vi "myRIO_BRig_RT_v0,86_PortC.vi"() -> ()   [LabVIEW 2014]
uses:
  myRIO_BRig_RT__Case_Exp_stateList.ctl
  myRIO_BRig_RT__Case_NonExp_stateList.ctl
  <vilib>/Platform/TimedLoop/XDataNode/timing_clust.ctl
  <vilib>/Platform/TimedLoop/XDataNode/nitl_modes.ctl
  <vilib>/Platform/TimedLoop/XDataNode/wakeup.ctl
  <vilib>/WebDAVClient/Advanced/SessionHandle.ctl
  <vilib>/myRIO/Common/Instrument Driver Framework/myRIO v1.0/UART/vis/myRIO v1.0 Close UART.vi
  <vilib>/FPGAPlugInAG/myRIO-1900/niLvFpga_Open_myRIO-1900.vi
  <vilib>/rvi/interface/common/dynamic/niFpgaDynamicAddResources.vi
  <vilib>/Utility/error.llb/Error Cluster From Error Code.vi
  <vilib>/rvi/errors/niLvFpgaAdjustHostInterfaceError.vi
  <vilib>/FPGAPlugInAG/Dynamic/niLvFpga_Close_Dynamic.vi
  <vilib>/myRIO/Common/Instrument Driver Framework/Utilities/vis/FPGA Ref Manager.vi
  <vilib>/myRIO/Common/Instrument Driver Framework/myRIO v1.0/myRIO v1.0 Reset FPGA.vi
  <vilib>/myRIO/Common/Instrument Driver Framework/myRIO v1.0/IRQ/vis/myRIO v1.0 IRQ Info FGV.vi
  <vilib>/myRIO/Common/Instrument Driver Framework/myRIO v1.0/IRQ/vis/myRIO v1.0 Timer IRQ Info FGV.vi
  <vilib>/myRIO/Common/Instrument Driver Framework/myRIO v1.0/IRQ/vis/myRIO v1.0 ISR Agent.vi
  <vilib>/rvi/interface/nirviOpenFPGA/nirviOpenFPGA.xnode
  myRIO_BRig_FPGA_v3,81__PortC__build.lvbitx
  myRIO_BRig_FPGA_v3,81__PortC.vi
  <vilib>/rvi/interface/nirviReadWriteControl/nirviReadWriteControl.xnode
  <vilib>/Platform/TimedLoop/XDataNode/XDataNode.xnode
  <vilib>/rvi/interface/nirviCloseFPGA/nirviCloseFPGA.xnode
  <vilib>/Platform/TimedLoop/XDataNode/XDNodeRunTimeDep.lvlib
  <vilib>/rvi/interface/Simulation/niFpgaSimulationCallBeginRW.vi
  <vilib>/myRIO/Instrument Drivers/Utilities/Utilities.lvlib
  <vilib>/WebDAVClient/NI_WebDAV.lvlib
  NiFpgaLv.dll
panel:
  in  "Laser2_baseline":bool
  in  "Laser1_baseline":bool
  in  "CueLed_baseline":bool
  out "allReward_R":bool
  out "allReward_L":bool
  in  "I_allReward":bool caption="NonSpecific Lick Direction"
  in  "Tcycle_Reward_max_R":u16=1000 caption="Max" min=5 max=5000 step=5
  in  "Tcycle_Reward_min_R":u16=1000 caption="Min" min=5 max=5000 step=5
  in  "Tcycle_Reward_step_R":u16=1000 caption="Penalty" min=1 max=10000 step=1
  in  "Tcycle_Reward_max_L":u16=1000 caption="Max" min=5 max=5000 step=5
  in  "Tcycle_Reward_min_L":u16=1000 caption="Min" min=5 max=5000 step=5
  in  "Tcycle_Reward_step_L":u16=1000 caption="Penalty" min=1 max=10000 step=1
  in  "MTrig_CueLed":bool
  out "Threshold":bool
  out "tLoop":dbl
  in  "Tcycle_Cue_LED_max":u16=1000 caption="Max" min=5 max=5000 step=5
  in  "Tcycle_Cue_LED_min":u16=1000 caption="Min" min=5 max=5000 step=5
  in  "Tcycle_CuePenalty_LED":u16=1000 caption="Penalty" min=1 max=10000 step=1
  out "power_l2":dbl
  in  "MTrig_Laser_Switch":bool
  in  "Cue1Param_AudioLed_Count_NS":u16
  in  "Cue1Param_AudioLed_Count_Switch":u16
  in  "Cue1Param_AudioLed_Probability_NS":u16
  in  "Cue1Param_CueType_NS":u16(slide) max=3 step=1 scale=0.0..3.0
  in  "Cue1Param_AudioLed_Probability_Switch":u16
  in  "Cue1Param_CueType_Switch":u16(slide) max=3 step=1 scale=0.0..3.0
  in  "CueLed_Freq":dbl=10.0
  in  "CueLed_Tpeak":dbl=2.0
  in  "Laser_power_step_l2":dbl
  in  "Laser_power_max_l2":dbl
  in  "Laser_power_min_l2":dbl
  in  "Laser_Tshutter_l2":dbl=2.0
  in  "Laser_Freq_l2":dbl=10.0
  in  "Laser_Tpeak_l2":dbl=2.0
  in  "Laser_duration_l2":u16
  in  "LC_Sel_Count_NS_l2":u16
  in  "LC_Sel_Count_Switch_l2":u16
  in  "LC_Sel_Probability_NS_l2":u16
  in  "LC_Sel_Block_NS_l2":u16(slide) max=2 step=1 scale=0.0..2.0
  in  "LC_Sel_OnOff_NS_l2":bool
  in  "LC_Sel_Probability_Switch_l2":u16
  in  "LC_Sel_Block_Switch_l2":u16(slide) max=2 step=1 scale=0.0..2.0
  in  "LC_Sel_OnOff_Switch_l2":bool
  in  "LC_Sel_Tdelay_NS_l2":u16
  in  "LC_Sel_Tdelay_Switch_l2":u16
  in  "LC_Cue1_Count_NS_l2":u16
  in  "LC_Cue1_Count_Switch_l2":u16
  in  "LC_Cue1_delayOpt_NS_l2":bool
  in  "LC_ENL1_delayOpt_NS_l2":bool
  in  "LC_ENL1_Count_NS_l2":u16
  in  "LC_ENL1_Count_Switch_l2":u16
  in  "LC_Cue1_delayOpt_Switch_l2":bool
  in  "LC_ENL1_delayOpt_Switch_l2":bool
  in  "LC_Cue1_Probability_NS_l2":u16
  in  "LC_Cue1_Block_NS_l2":u16(slide) max=2 step=1 scale=0.0..2.0
  in  "LC_Cue1_OnOff_NS_l2":bool
  in  "LC_Cue1_Probability_Switch_l2":u16
  in  "LC_Cue1_Block_Switch_l2":u16(slide) max=2 step=1 scale=0.0..2.0
  in  "LC_Cue1_OnOff_Switch_l2":bool
  in  "LC_ENL1_Probability_NS_l2":u16 max=100 step=1
  in  "LC_ENL1_Block_NS_l2":u16(slide) max=2 step=1 scale=0.0..2.0
  in  "LC_ENL1_OnOff_NS_l2":bool
  in  "LC_ENL1_Probability_Switch_l2":u16 max=100 step=1
  in  "LC_ENL1_Block_Switch_l2":u16(slide) max=2 step=1 scale=0.0..2.0
  in  "LC_Cue1_Tdelay_NS_l2":u16
  in  "LC_ENL1_Tdelay_NS_l2":u16
  in  "LC_Cue1_Tdelay_Switch_l2":u16
  in  "LC_ENL1_Tdelay_Switch_l2":u16
  in  "LC_ENL1_OnOff_Switch_l2":bool
  in  "LC_Wrong_Probability_l2":u16
  in  "LC_Wrong_Trial_l2":u16(slide) max=2 step=1 scale=0.0..2.0
  in  "LC_Wrong_Block_l2":u16(slide) max=2 step=1 scale=0.0..2.0
  in  "LC_Wrong_OnOff_l2":bool
  in  "LC_Reward_Probability_l2":u16
  in  "LC_Reward_Trial_l2":u16(slide) max=2 step=1 scale=0.0..2.0
  in  "LC_Reward_Block_l2":u16(slide) max=2 step=1 scale=0.0..2.0
  in  "LC_Reward_OnOff_l2":bool
  in  "LC_Wrong_Tdelay_l2":u16
  in  "LC_Reward_Tdelay_l2":u16
  in  "LC_Sel_Count_NS_l1":u16
  in  "LC_Sel_Count_Switch_l1":u16
  in  "LC_Sel_Probability_NS_l1":u16
  in  "LC_Sel_Block_NS_l1":u16(slide) max=2 step=1 scale=0.0..2.0
  in  "LC_Sel_OnOff_NS_l1":bool
  in  "LC_Sel_Probability_Switch_l1":u16
  in  "LC_Sel_Block_Switch_l1":u16(slide) max=2 step=1 scale=0.0..2.0
  in  "LC_Sel_OnOff_Switch_l1":bool
  in  "LC_Sel_Tdelay_NS_l1":u16
  in  "LC_Sel_Tdelay_Switch_l1":u16
  out "I_connect_TCP":bool
  in  "get_countPerMS":bool
  in  "count_warmup_R_reset":bool
  in  "count_warmup_L_reset":bool
  out "count_warmup_R":u16
  out "count_warmup_L":u16
  out "SolenoidReward":bool
  in  "SolenoidProbability_L":u16=100 caption="Reward Time [ms]" min=1 max=1000 step=1
  in  "SolenoidProbability_R":u16=100 caption="Reward Time [ms]" min=1 max=1000 step=1
  out "power_l1":dbl caption="LaserPower"
  in  "Laser_power_step_l1":dbl
  in  "Laser_power_max_l1":dbl
  in  "Recording":bool
  in  "Laser_power_min_l1":dbl
  in  "FPGA_count2ms":dbl=159.0
  in  "Laser_Tshutter_l1":dbl=2.0
  in  "Laser_Freq_l1":dbl=10.0
  in  "Laser_Tpeak_l1":dbl=2.0
  in  "Laser_duration_l1":u16
  out "error out":errorcluster
  in  "LC_Cue1_Count_NS_l1":u16
  in  "LC_Cue1_Count_Switch_l1":u16
  in  "LC_Cue1_delayOpt_NS_l1":bool
  in  "LC_ENL1_delayOpt_NS_l1":bool
  in  "LC_ENL1_Count_NS_l1":u16
  in  "LC_ENL1_Count_Switch_l1":u16
  in  "LC_Cue1_delayOpt_Switch_l1":bool
  in  "LC_ENL1_delayOpt_Switch_l1":bool
  in  "Tcycle_Cue_Audio_max":u16=1000 caption="Max" min=5 max=5000 step=5
  in  "Tcycle_Cue_Audio_min":u16=1000 caption="Min" min=5 max=5000 step=5
  in  "SendData":bool
  out "cSpout":enum16{"Left", "Right"}(ring) caption="Left or Right Spout"
  out "A4":u32 caption="LickCounter_Right"
  out "A2":u32 caption="LickCounter_Left"
  in  "LR_wrong_Event":bool
  out "SelectWrong":bool
  out "SelectReward":bool
  in  "Left(F)_or_Right(T)":bool
  in  "ignoreWrong":bool
  in  "SelectionState":bool
  in  "LR_wrong_Laser":bool
  in  "LR_reward_Laser":bool
  in  "LR_reward_Event":bool
  out "nRewards_Right":u16 caption="# Rewards Total (Right)"
  out "nRewards_Left":u16 caption="# Rewards Total (Left)"
  out "nRewards_cur":u16 caption="# Rewards in Current Block"
  out "TpB_target":u16 caption="Target Trials Per Block"
  out "cState_NonExp":T1 caption="WarmUp State"
  out "iBlock":u16 caption="Current Block"
  out "cState":T2 caption="Experimental State"
  out "iTrial":u16 caption="Current Trial"
  in  "warmupType":u8(slide) max=2 step=1 scale=0.0..2.0
  in  "TestConnection":bool
  in  "warmup":bool caption="WarmUp"
  in  "Data Set Prefix":string="Exp1_TM2"
  out "Connected To Host?":bool
  in  "Host Password":string="sabalab"
  in  "Host UserName":string="Test2"
  in  "sp_RightSpout":u16(slide)=2 max=2 step=1 scale=0.0..2.0
  in  "sp_LeftSpout":u16(slide)=2 max=2 step=1 scale=0.0..2.0
  in  "BUR_max":u16 caption="Count Reward Structure  (0 = off)"
  in  "LC_Wrong_Probability_l1":u16
  in  "LC_Wrong_Trial_l1":u16(slide) max=2 step=1 scale=0.0..2.0
  in  "LC_Wrong_Block_l1":u16(slide) max=2 step=1 scale=0.0..2.0
  in  "LC_Wrong_OnOff_l1":bool
  in  "LC_Reward_Probability_l1":u16
  in  "LC_Reward_Trial_l1":u16(slide) max=2 step=1 scale=0.0..2.0
  in  "LC_Reward_Block_l1":u16(slide) max=2 step=1 scale=0.0..2.0
  in  "LC_Reward_OnOff_l1":bool
  in  "LC_Cue1_Probability_NS_l1":u16
  in  "LC_Cue1_Block_NS_l1":u16(slide) max=2 step=1 scale=0.0..2.0
  in  "LC_Cue1_OnOff_NS_l1":bool
  in  "LC_Cue1_Probability_Switch_l1":u16
  in  "LC_Cue1_Block_Switch_l1":u16(slide) max=2 step=1 scale=0.0..2.0
  in  "LC_Cue1_OnOff_Switch_l1":bool
  in  "LC_ENL1_Probability_NS_l1":u16 max=100 step=1
  in  "LC_ENL1_Block_NS_l1":u16(slide) max=2 step=1 scale=0.0..2.0
  in  "LC_ENL1_OnOff_NS_l1":bool
  in  "LC_ENL1_Probability_Switch_l1":u16 max=100 step=1
  in  "LC_ENL1_Block_Switch_l1":u16(slide) max=2 step=1 scale=0.0..2.0
  in  "Tcycle_Timeout":u16=1000 caption="Timeout Time [ms]" min=10 max=10000 step=1
  in  "Tcycle_Wrong":u16=1000 caption="Wrong Time [ms]" min=10 max=10000 step=1
  in  "Tcycle_Selection":u16=1000 caption="Answer Time [ms]" min=1 max=10000 step=1
  in  "Tcycle_RewardPost":u16=1000 caption="Consumption Time [ms]" min=250 max=10000 step=250
  in  "TpB_Max_R":u16=4 caption="Max TrialsPerBlock" min=1 max=12 step=1
  in  "TpB_Min_R":u16=4 caption="Min TrialsPerBlock" min=1 max=12 step=1
  in  "TpB_Max_L":u16=4 caption="Max TrialsPerBlock" min=1 max=12 step=1
  in  "TpB_Min_L":u16=4 caption="Min TrialsPerBlock" min=1 max=12 step=1
  in  "BUR_min":u16 caption="Count Reward Structure\n(0 = off)"
  in  "TrialUntilReward":bool caption="Ignore Wrong Selection"
  in  "CueCycles":u16=1 caption="Cue Structure" min=1 max=1 step=1
  in  "MTrig_Laser_Tcycle":u16=10 caption="Time [ms]"
  in  "MTrig_Laser_trig":bool
  in  "MTrig_Audio_trig__R":bool caption="Trigger Audio"
  in  "MTrig_Audio_trig__L":bool caption="Trigger Audio"
  in  "RewCalib_Trig_R":bool caption="Calibrate_R"
  in  "RewCalib_Trig_L":bool caption="Calibrate_L"
  in  "MTrig_Solenoid_Tcycle__R":u16=300 caption="Time [ms]"
  in  "MTrig_Solenoid_Tcycle__L":u16=300 caption="Time [ms]"
  in  "MTrig_Solenoid_trig__R":bool caption="Solenoid"
  in  "MTrig_Solenoid_trig__L":bool caption="Solenoid"
  in  "STOP_abort":bool caption="Stop LabView\n(Stops myRio and FPGA)"
  in  "STOP_endBlock":bool caption="Stop Experiment\n@ End of Block"
  in  "STOP_endTrial":bool caption="Stop Experiment\n@ End of Trial"
  in  "START":bool caption="Start Experiment"
  in  "Tcycle_CuePenalty_Audio":u16=1000 caption="Penalty" min=1 max=10000 step=1
  in  "Audio_Amp__R":u16=100 caption="Amp"
  in  "Audio_Freq__R":u8=5 caption="Freq [kHz]" max=14 step=1
  in  "Audio_Amp__L":u16=100 caption="Amp"
  in  "Audio_Freq__L":u8=5 caption="Freq [kHz]" max=14 step=1
  in  "LC_Wrong_Tdelay_l1":u16
  in  "LC_Cue1_Tdelay_NS_l1":u16
  in  "LC_ENL1_Tdelay_NS_l1":u16
  in  "LC_Reward_Tdelay_l1":u16
  in  "LC_Cue1_Tdelay_Switch_l1":u16
  in  "LC_ENL1_Tdelay_Switch_l1":u16
  in  "LC_ENL1_OnOff_Switch_l1":bool
  in  "Tcycle_ENLPenalty":u16=100 caption="Penalty" min=10 max=10000 step=10
  in  "Tcycle_ENL_max":u16=1000 caption="Max" min=250 max=10000 step=250
  in  "Tcycle_ENL_min":u16=1000 caption="Min" min=250 max=10000 step=250
  # "Communication (Host PC)"
  # "Recording Rig"
  # "Experimental Run"
  # "Experiment Task Structure"
  # "STOP experiment at"
  # "(1) = Switching\n(2) = Two Choice"
  # "Min            Max            Penalty"
  # "Enforced\nNonLick"
  # "FPGA Count per [ms]"
  # "Cue Audio"
  # "Current State"
  # "Cue LED"
  # "Global Parameters                                                         Trial Parameters"
  # "Selection"
  # "WarmUp"
  # "Reward - Dispense Water"
  # "Left/Right        Give Reward?        Laser Power [V]"
  # "Min            Max            StepSize"
  # "Laser1      Laser2"
  # "Left"
  # "Cue then reward (no lick)\n \nLeft                    Right"
  # "Right"
  # "Min"
  # "Max"
  # "Dispense Water Probability"
  # "Block                   Trial            Target Trials       # Rewards \n                                                            Per Block             Current"
  # "%"
  # "Left"
  # "WarmUp State"
  # "Trial Per Block Structure \n               Left                        Right"
  # "Lick Counter"
  # "Right"
  # "%"
  # "Left           Right"
  # "Reward - Consumption"
  # "Manual Control"
  # "Min"
  # "# Rewards Total\n                                                                  Left                    Right"
  # "Experimental State"
  # "Penalty - Wrong Choice"
  # "Solenoid\n \nLeft              Right"
  # "Speaker\n \nLeft                    Right"
  # "Laser 1  |  Laser 2"
  # "Max"
  # "Penalty - Choice Timeout"
  # "Time\n[ms]"
  # "Time\n[ms]"
  # "Time = Cue Min"
  # "Cue LED"
  # "Power = Min"
  # "Cue1 Control\n                                  Cue Type           LED Probability [%]      Count"
  # "Laser1 Control\n                               On/Off      Block        Probability [%]   Delay [ms]                              Count"
  # "Laser2 Control\n                               On/Off      Block        Probability [%]   Delay [ms]                              Count"
  # "Audio or LED"
  # "Cue 1"
  # "Enforced\nNonLick\n      1"
  # "Enforced\nNonLick\n      1"
  # "from end"
  # "from end"
  # "Switch\nTrial"
  # "Switch\nTrial"
  # "Switch\nTrial"
  # "from start"
  # "from start"
  # "from end"
  # "from end"
  # "NonSwitch\nTrials"
  # "NonSwitch\nTrials"
  # "NonSwitch\nTrials"
  # "from start"
  # "from start"
  # "Cue 1"
  # "Cue 1"
  # "from end"
  # "from end"
  # "Switch\nTrial"
  # "Switch\nTrial"
  # "Cue Audio Parameters"
  # "Cue LED Parameters"
  # "from start"
  # "from start"
  # "Left                  Right"
  # "Frequency\n[Hz]"
  # "Frequency\n[kHz]"
  # "from end"
  # "from end"
  # "NonSwitch\nTrials"
  # "NonSwitch\nTrials"
  # "Timing [ms]\n                    Peak Width"
  # "from start"
  # "from start"
  # "Amp\n(0 - 32,000)"
  # "Selection"
  # "Selection"
  # "from start"
  # "from start"
  # "Switch\nTrial"
  # "Switch\nTrial"
  # "Speaker\nPattern\nDuring Cue"
  # "from start"
  # "from start"
  # "NonSwitch\nTrials"
  # "NonSwitch\nTrials"
  # "Laser1 Parameters"
  # "Laser2 Parameters"
  # "Laser1 Response\n                               On/Off      Block       Trial       Probability [%]   Delay [ms]"
  # "Laser2 Response\n                               On/Off      Block       Trial       Probability [%]   Delay [ms]"
  # "Frequency\n[Hz]"
  # "Frequency\n[Hz]"
  # "Timing [ms]\n Duration     Peak Width   Shutter"
  # "Timing [ms]\n Duration     Peak Width   Shutter"
  # "Selection Reward"
  # "Selection Reward"
  # "Laser Power [V]\nMin          Max              Step"
  # "Laser Power [V]\nMin          Max              Step"
  # "Selection Wrong"
  # "Selection Wrong"
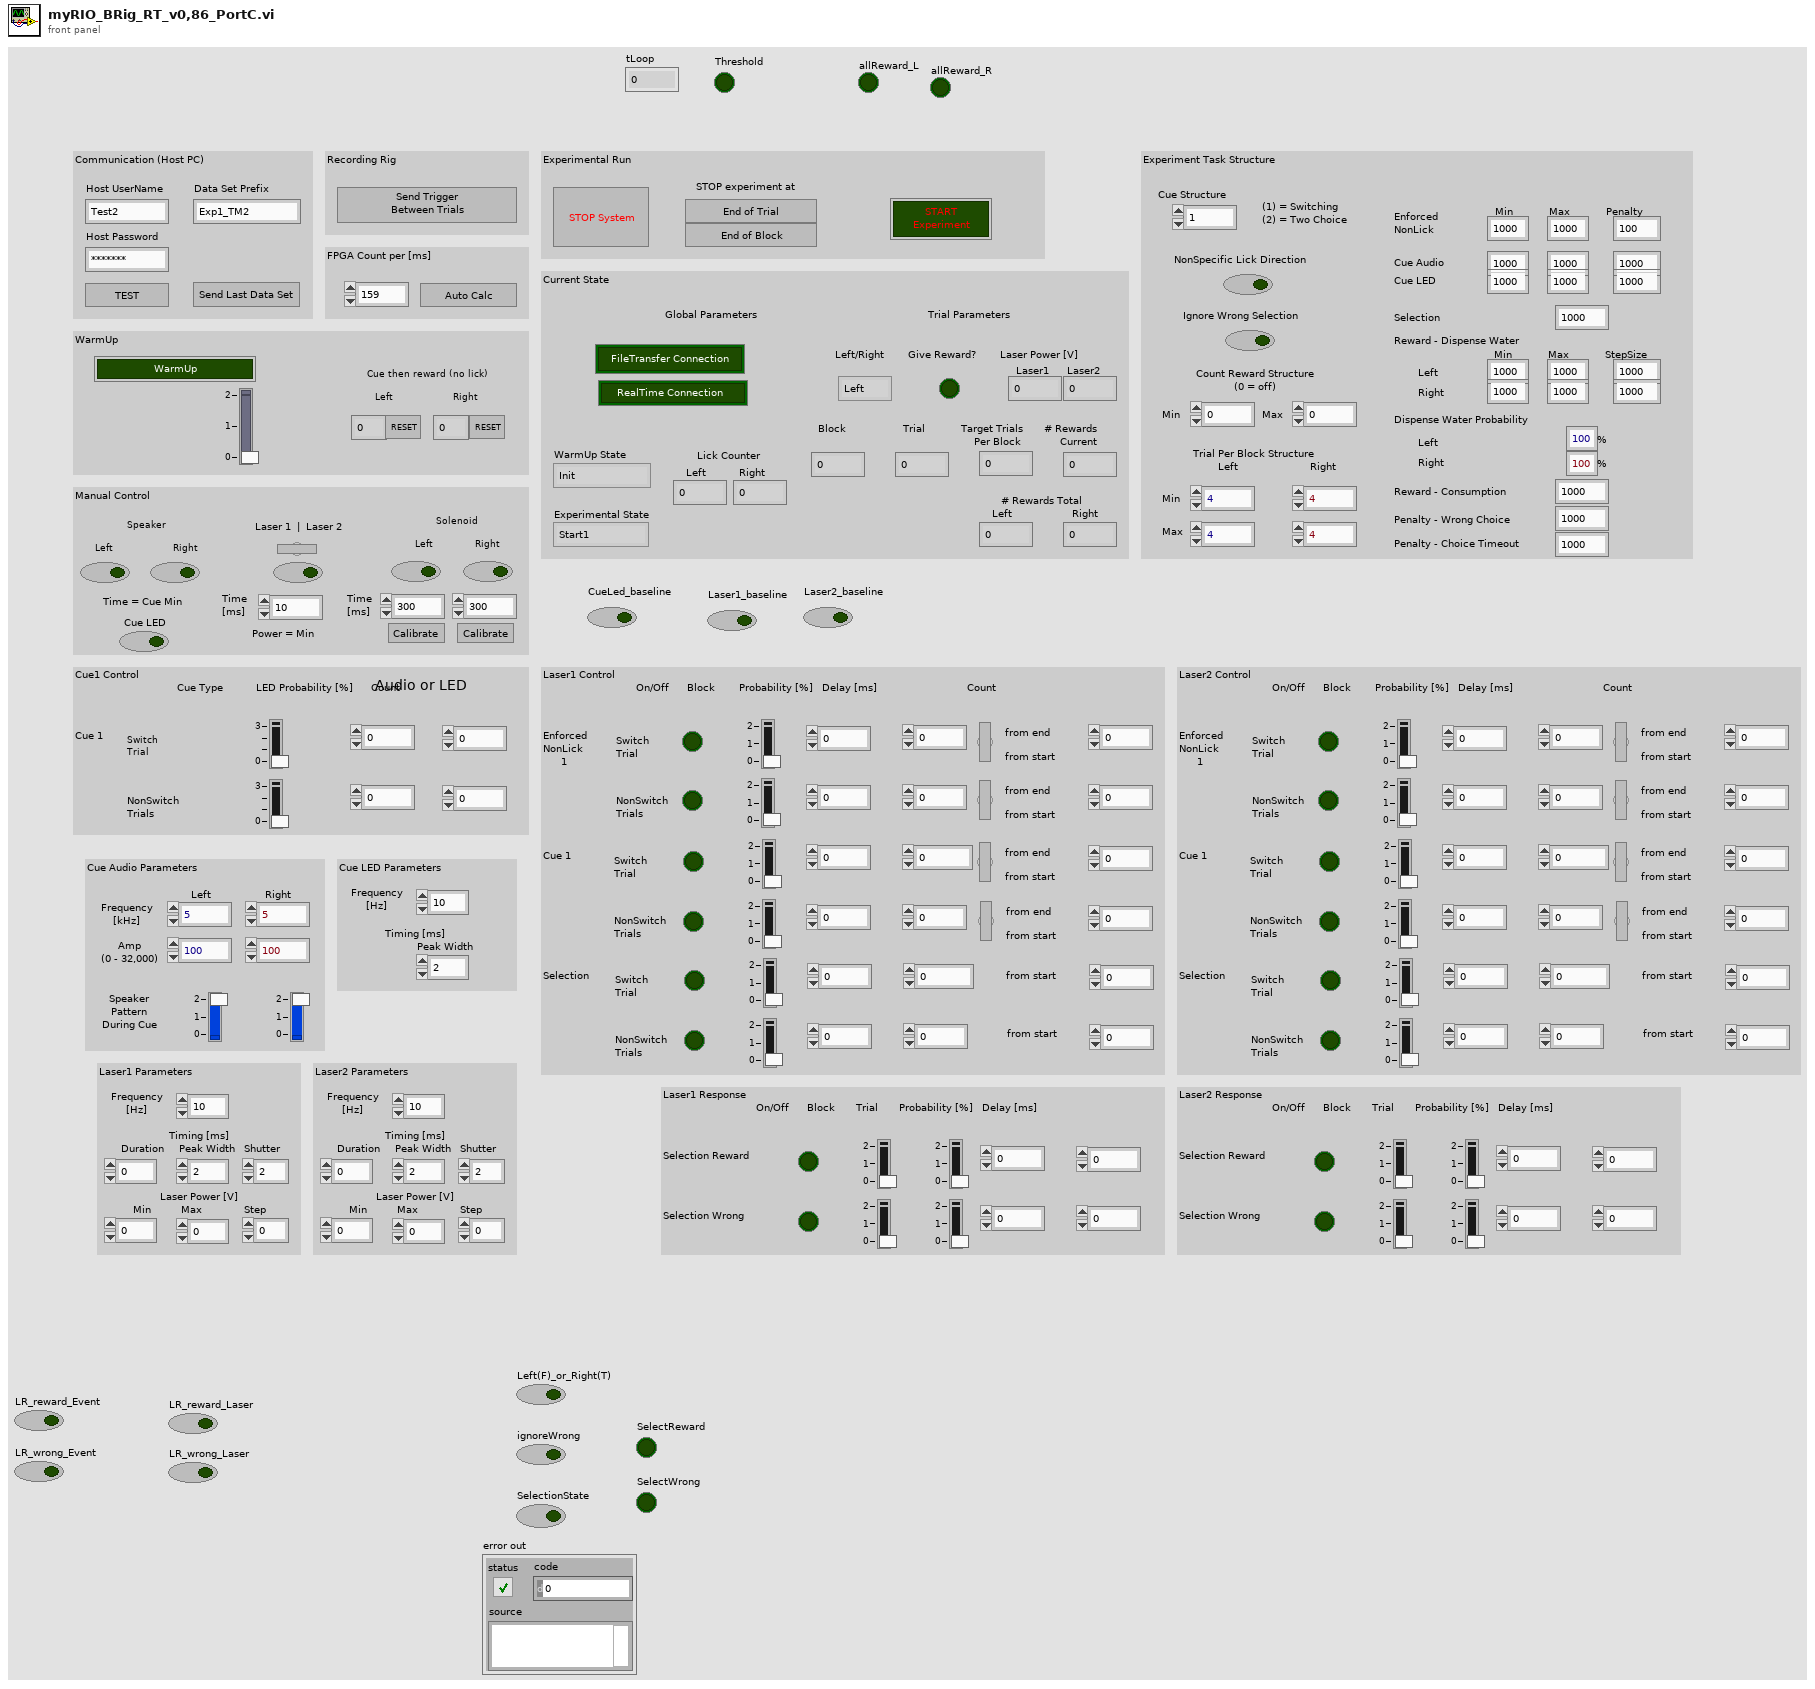
[diagram p1: front panel]
types:
  T1 = typedef "myRIO_BRig_RT__Case_NonExp_stateList.ctl" = enum16{"Init", "UploadSettings_pre", "UploadSettings_Read_dataExp", "UploadSettings_dataExp_1", "UploadSettings_dataExp_2", "UploadSettings_Read_dataLC", "UploadSettings_dataLC_1", "UploadSettings_dataLC_2", "UploadSettings_dataLC_3", "UploadSettings_dataLC_4", "UploadSettings_Read_dataMTrig", "UploadSettings_dataMTrig_1", "UploadSettings_post", "Idle_pre", "IdleEmpty", "IdleEmpty2", "IdleEmpty3", "IdleEmpty4", "Idle", "Idle_2", "Idle_3", "Idle_4", "Idle_5", "Idle_6", "Idle_post", "Cue_pre__pre", "Cue_pre", "Cue", "Cue_LED", "Cue_post", "RewardCalibration_pre", "DispenseWater_pre__pre", "DispenseWater_pre", "DispenseWater", "DispenseWater_post", "TestConnection", "SendData", "Get_FPGA_count_per_ms", "End"}
  T2 = typedef "myRIO_BRig_RT__Case_Exp_stateList.ctl" = enum16{"Start1", "Start2", "Start3", "saveSettings1", "saveSettings2", "saveSettings3", "saveSettings4", "saveSettings_LC_ENL_l1", "saveSettings_LC_ENL_l2", "saveSettings_LC_Cue_l1", "saveSettings_LC_Cue_l2", "saveSettings6_LC_l1_Other", "SaveSettings6_LC_l2_Other", "setSettings_Audio", "setSettings_Laser", "initBlock_pre", "initBlock", "initBlock2", "initBlock_post", "initTrial_pre", "initTrial", "initTrial2", "initTrial3", "initTrial4", "initTrial_LC_ENL1", "initTrial_LC_Cue1", "initTrial_LC_Cue1_2", "initTrial_LC_Sel", "initTrial_post", "ENL1_pre", "ENL1", "ENL1_post", "ENL1Penalty_pre", "ENL1Penalty", "ENL2_pre", "ENL2", "ENL2Penalty_pre", "ENL2Penalty", "Cue1_pre", "Cue1", "Cue1_post", "Cue1Penalty_pre", "Cue1Penalty", "Cue2_pre", "Cue2", "Cue2Penalty_pre", "Cue2Penalty", "Selection_pre", "Selection", "Select_post", "SelectReward_pre", "SelectReward", "SelectRewardPost_pre", "SelectRewardPost", "SelectWrong_pre", "SelectWrong", "SelectWrong_post", "SelectTimeout_pre", "SelectTimeout", "SelectTimeout_post", "endTrial_pre", "endTrial1", "endTrial2", "endTrial3", "endTrial_post", "endBlock_pre", "endBlock", "endBlock_post", "endExp", "commConnect", "commUpload_pre", "commUpload_dataBlock", "commUpload_dataCurrent", "commUpload_dataExp", "commUpload_dataLC", "commUpload_dataTrial", "commUpload_post", "saveData_pre", "saveData_dataBlock", "saveData_dataCurrent", "saveData_dataExp", "saveData_dataLC", "saveData_dataTrial", "saveData_post", "empty_endBlock1", "empty_endBlock2", "empty_endTrial1", "empty_endTrial2", "empty_endTrial3", "empty_endTrial4", "empty_endTrial5", "dummyState", "dummyState_endBlock"}
  T3 = typedef "XDNodeRunTimeDep.lvlib/timing_clust.ctl" = cluster{"Expected End [f-1]":u64, "Actual End [f-1]":u64, "Finished Late? [f-1]":bool, "Expected End [i-1]":u64, "Actual End [i-1]":u64, "Finished Late? [i-1]":bool, "Expected Start [i]":u64, "Actual Start [i]":u64, "Expected Start [f]":u64, "Actual Start [f]":u64, "Source Name":string, "Structure Name":string, "Period":i64, "Deadline":i64, "Offset":i64, "Start":i64, "Priority":i32, "Timeout":i32, "Mode":T4, "Wakeup Reason":T5, "Error":errorcluster, "Source Type":string, "Secondary Source Type":string, "Global End Time":u64, "Global Start Time":u64, "Frame Duration":u64, "Iteration Duration":u64, "Assigned CPU":i32, "I/O Scan Engine Mode":u32}
  T4 = typedef "XDNodeRunTimeDep.lvlib/nitl_modes.ctl" = enum32{"No Change", "Process missed periods, maintain original phase", "Discard missed periods, maintain original phase", "Process missed periods, ignore original phase", "Discard missed periods, ignore original phase"}
  T5 = typedef "XDNodeRunTimeDep.lvlib/wakeup.ctl" = enum32{"Normal", "Aborted", "Asynchronous wakeup", "Timing source error", "Timed loop error", "Timeout"}
  T6 = typedef "NI_WebDAV.lvlib/SessionHandle.ctl" = refnum<k1>
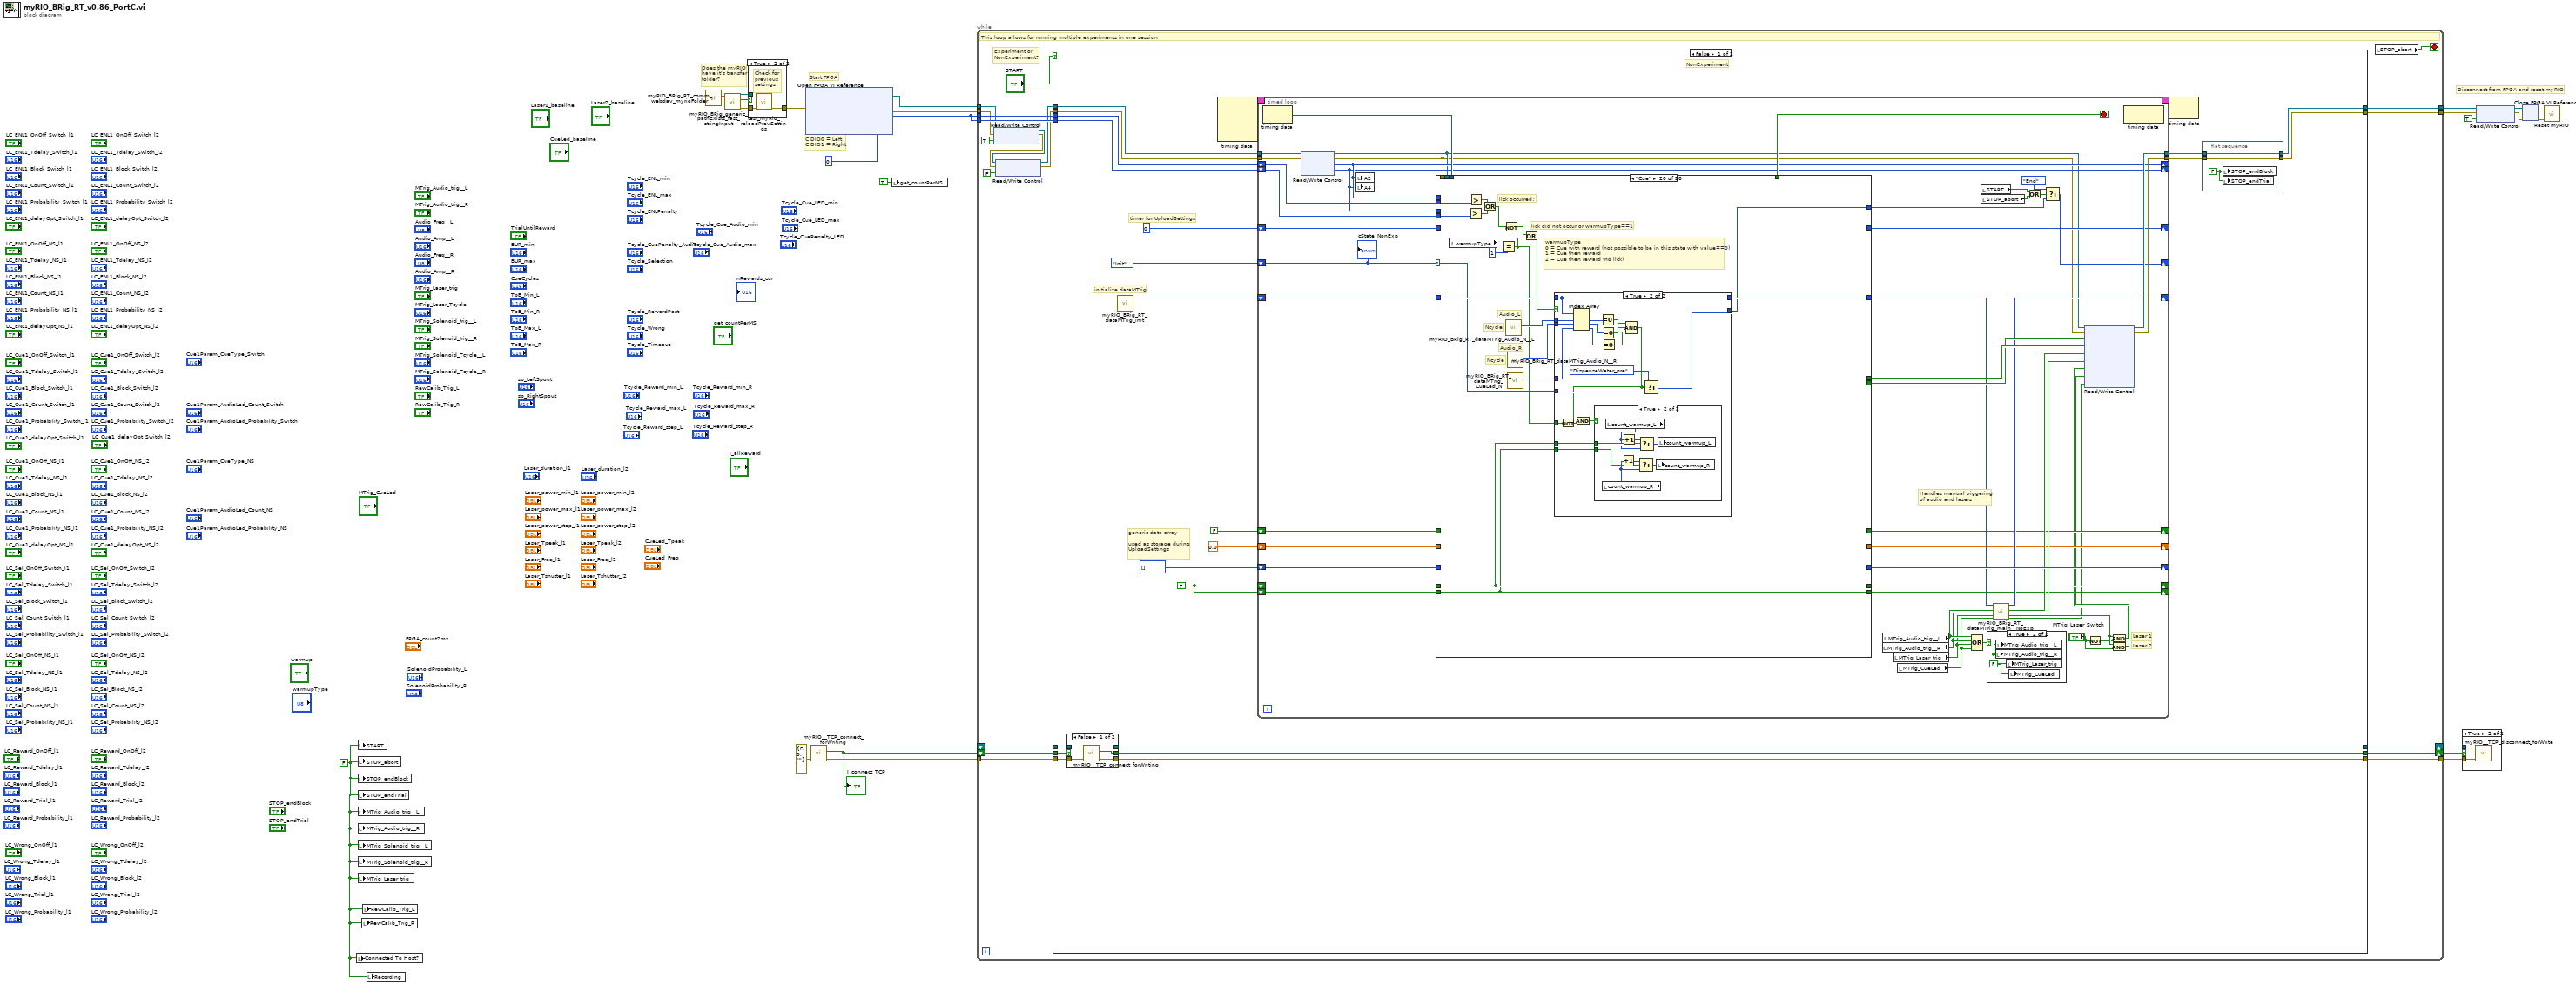
[diagram p0: block diagram]
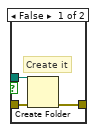
[diagram p3: hidden frame]
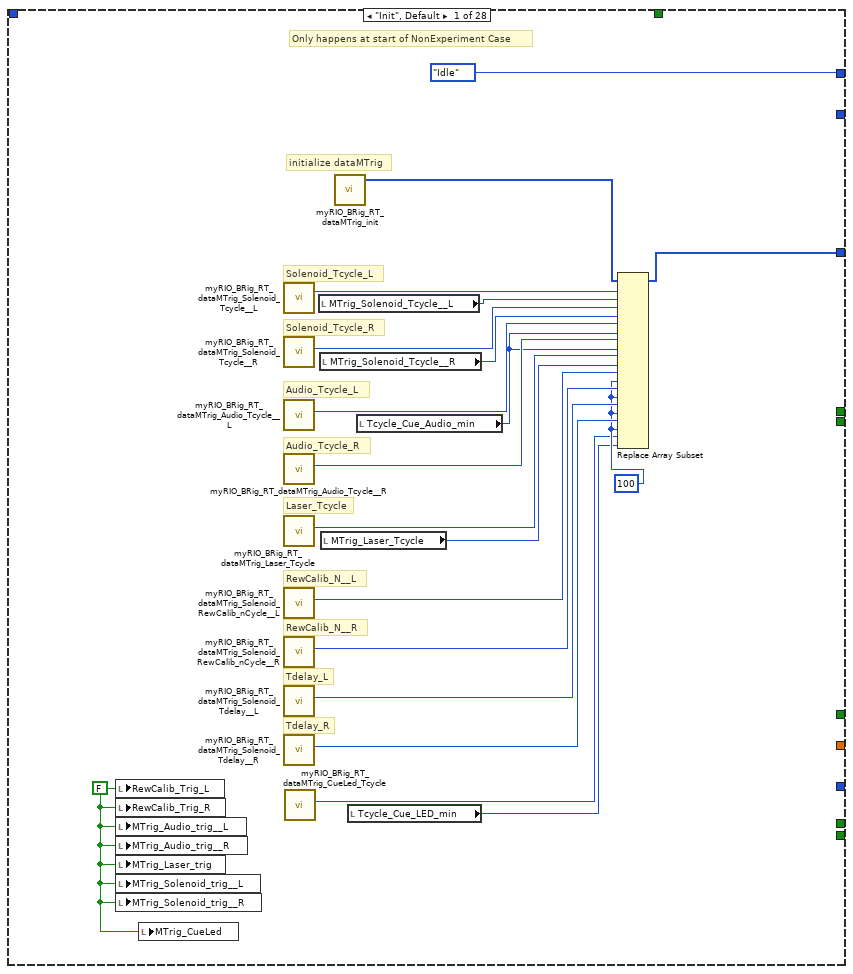
[diagram p6: hidden frame]
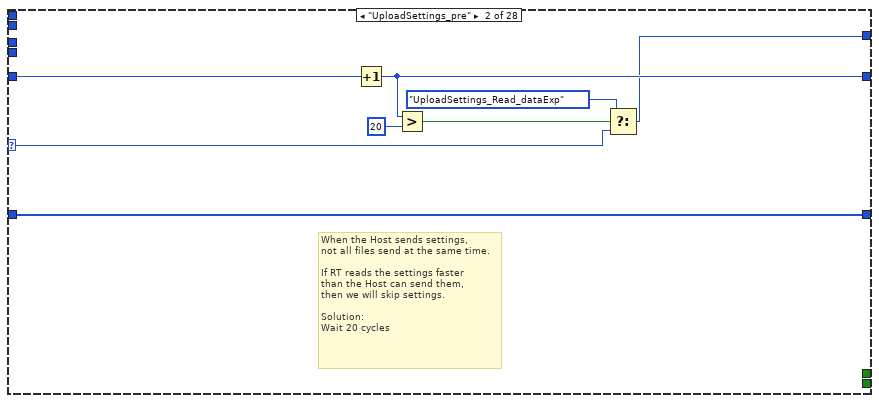
[diagram p7: hidden frame]
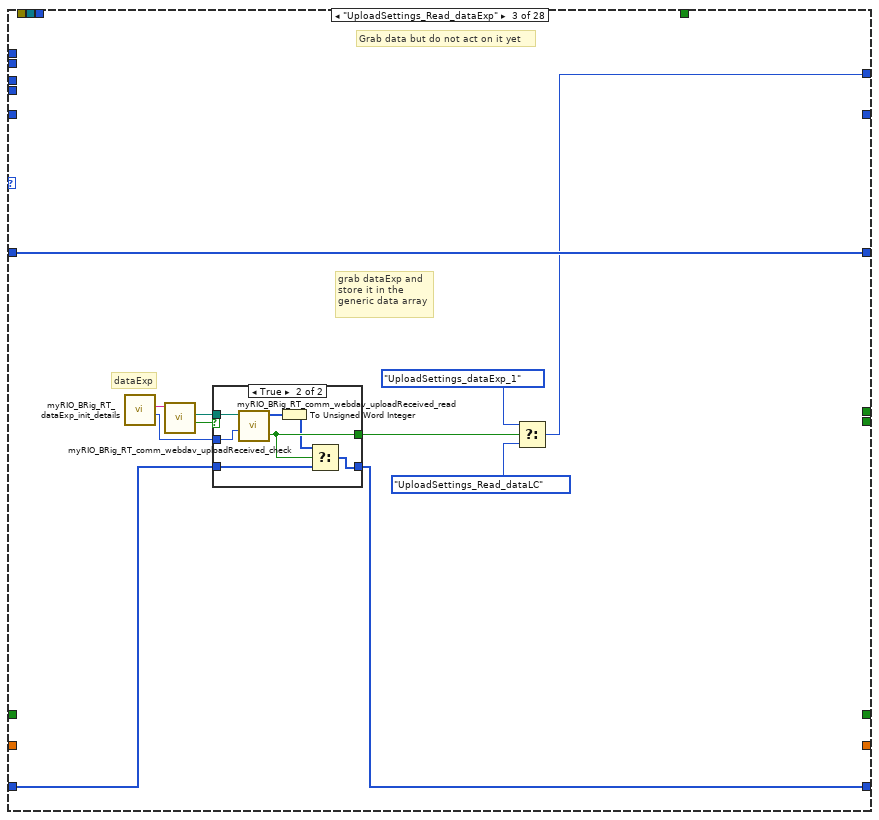
[diagram p8: hidden frame]
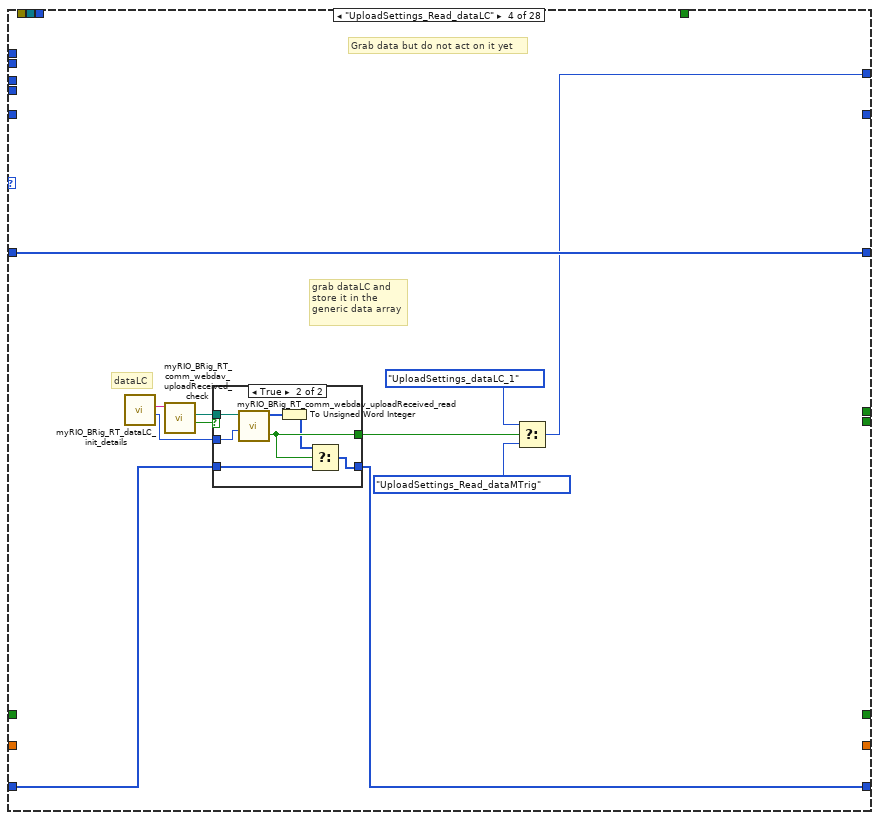
[diagram p10: hidden frame]
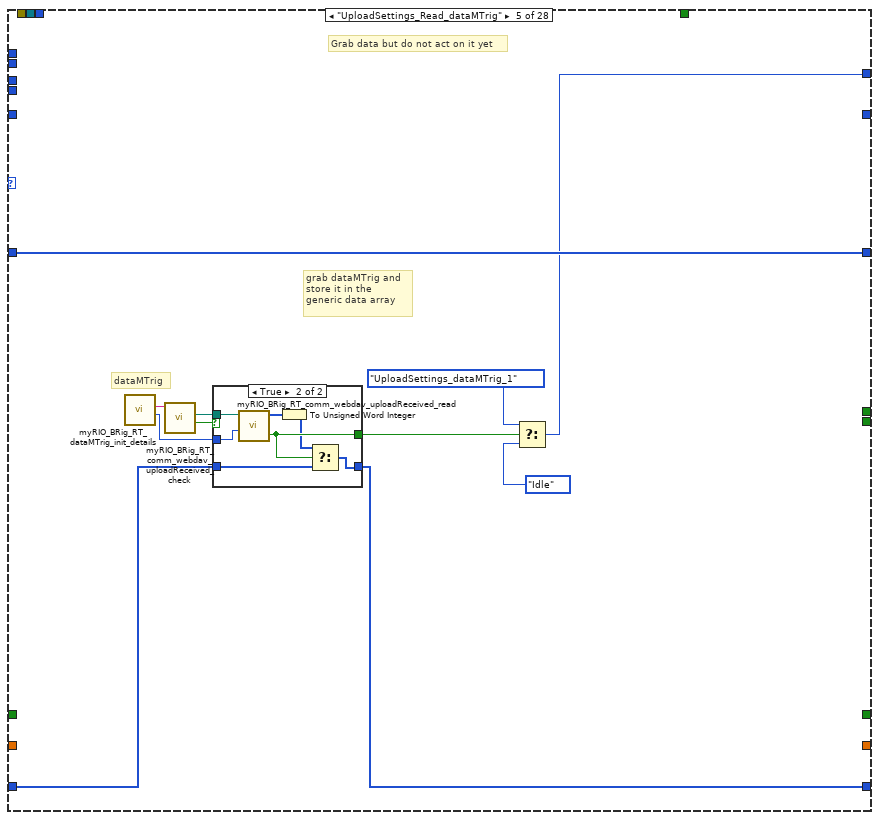
[diagram p12: hidden frame]
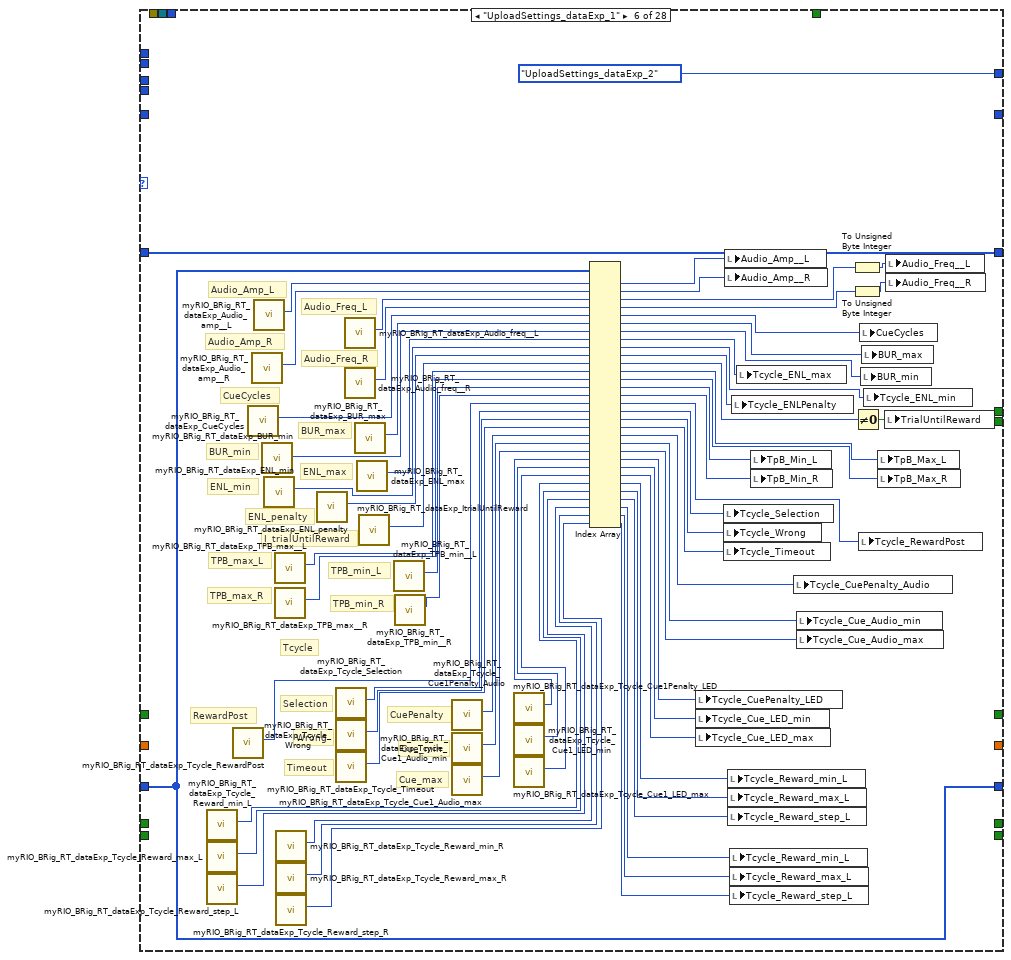
[diagram p14: hidden frame]
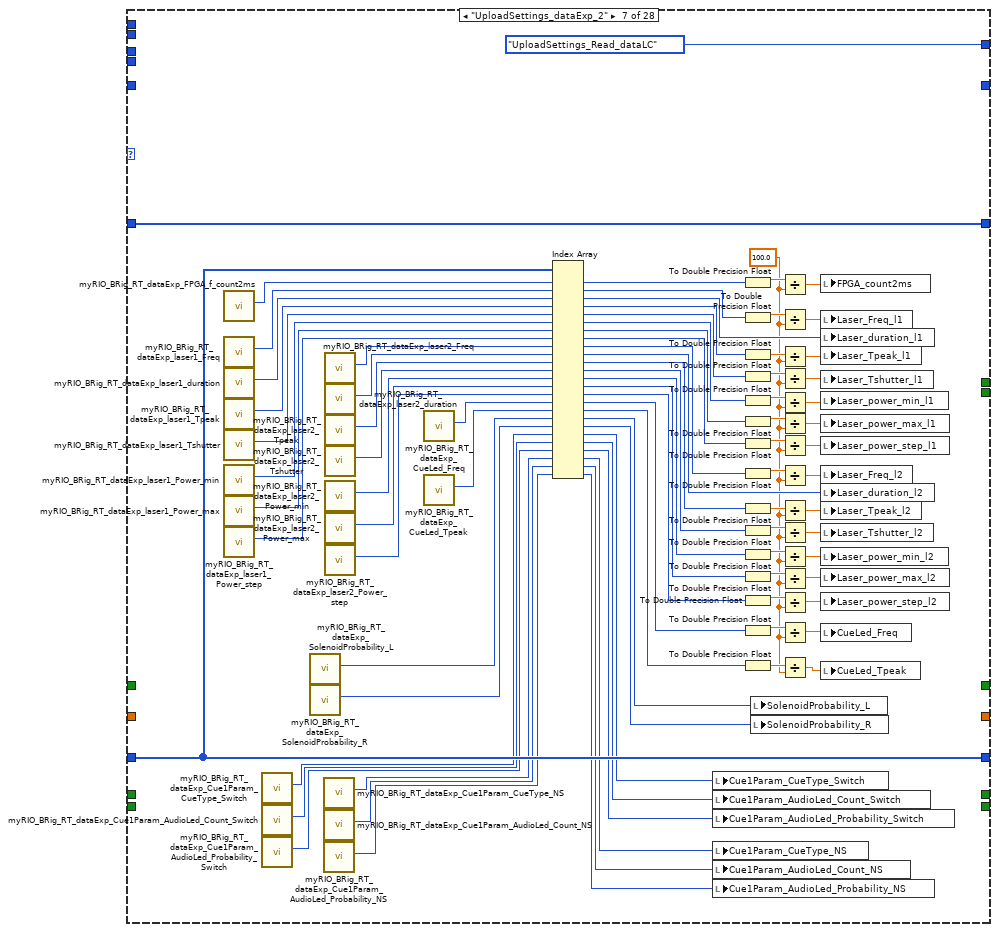
[diagram p15: hidden frame]
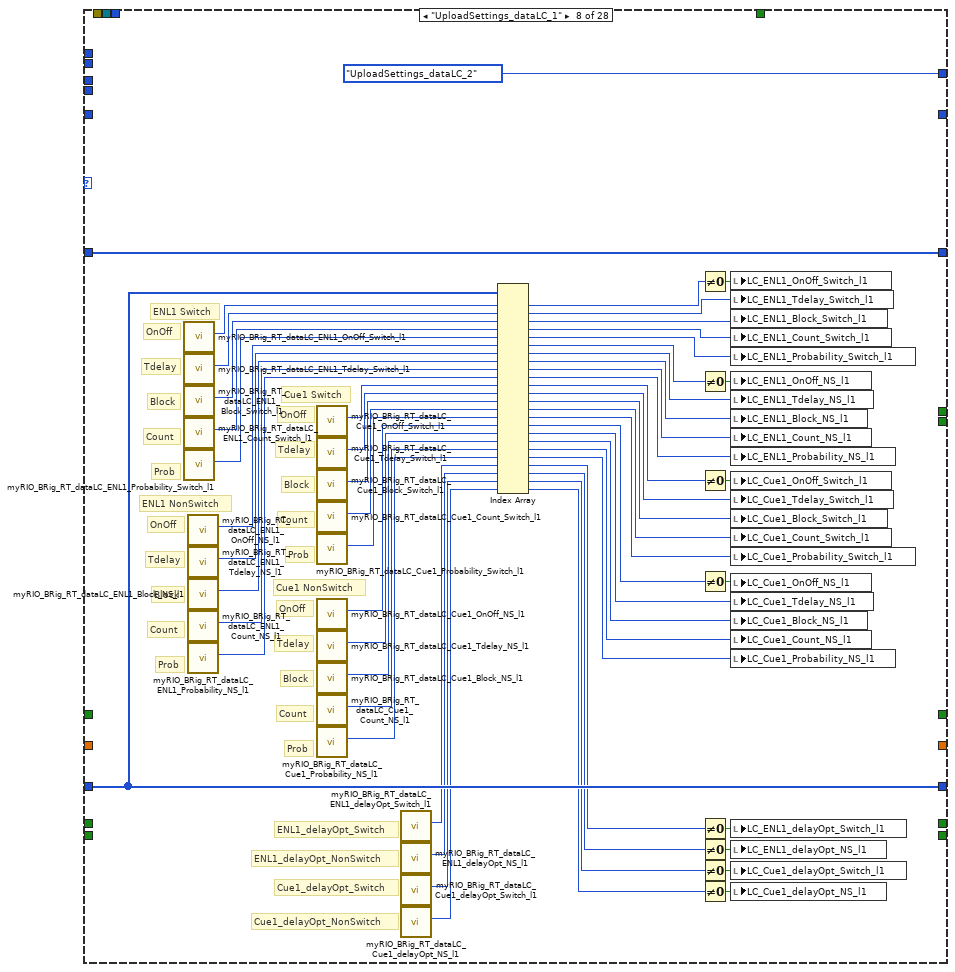
[diagram p16: hidden frame]
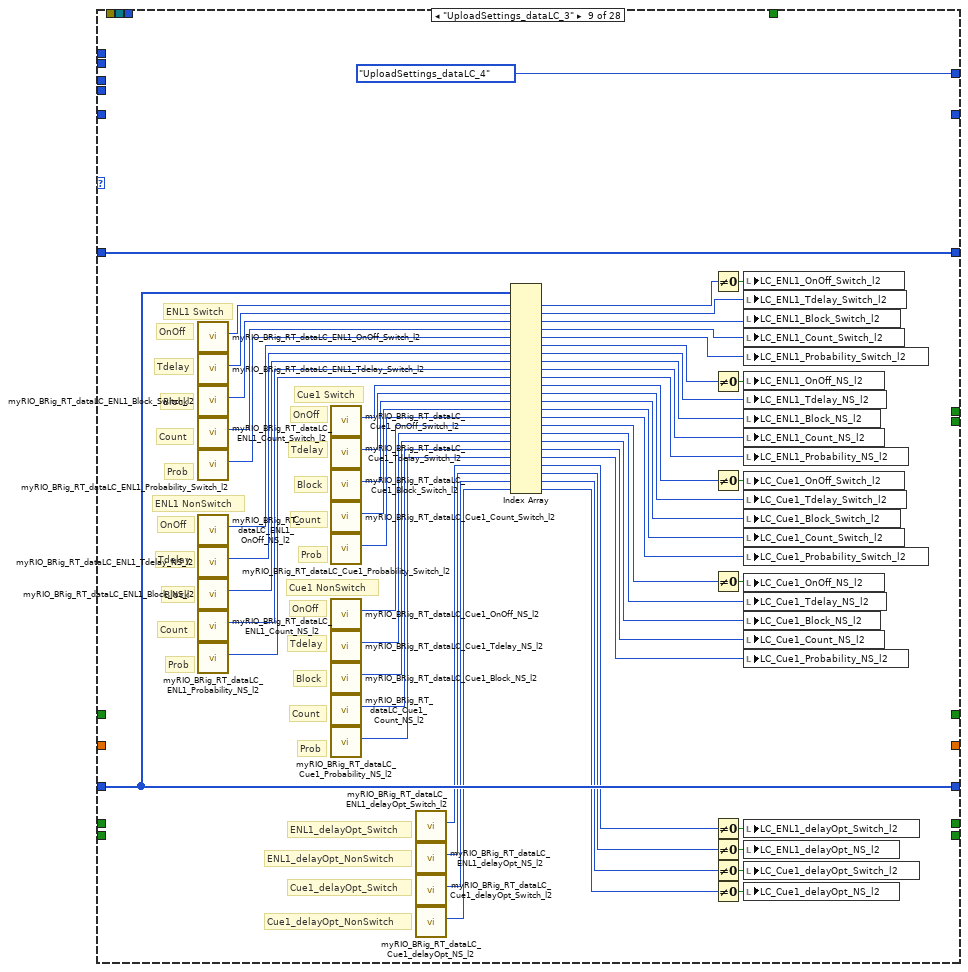
[diagram p17: hidden frame]
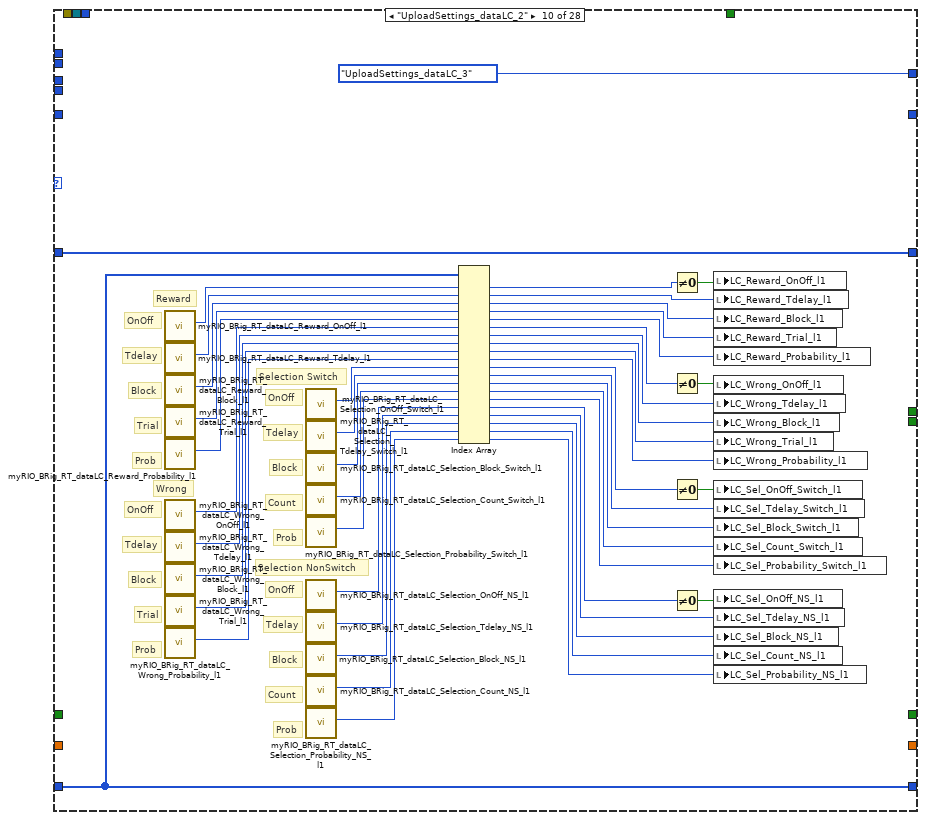
[diagram p18: hidden frame]
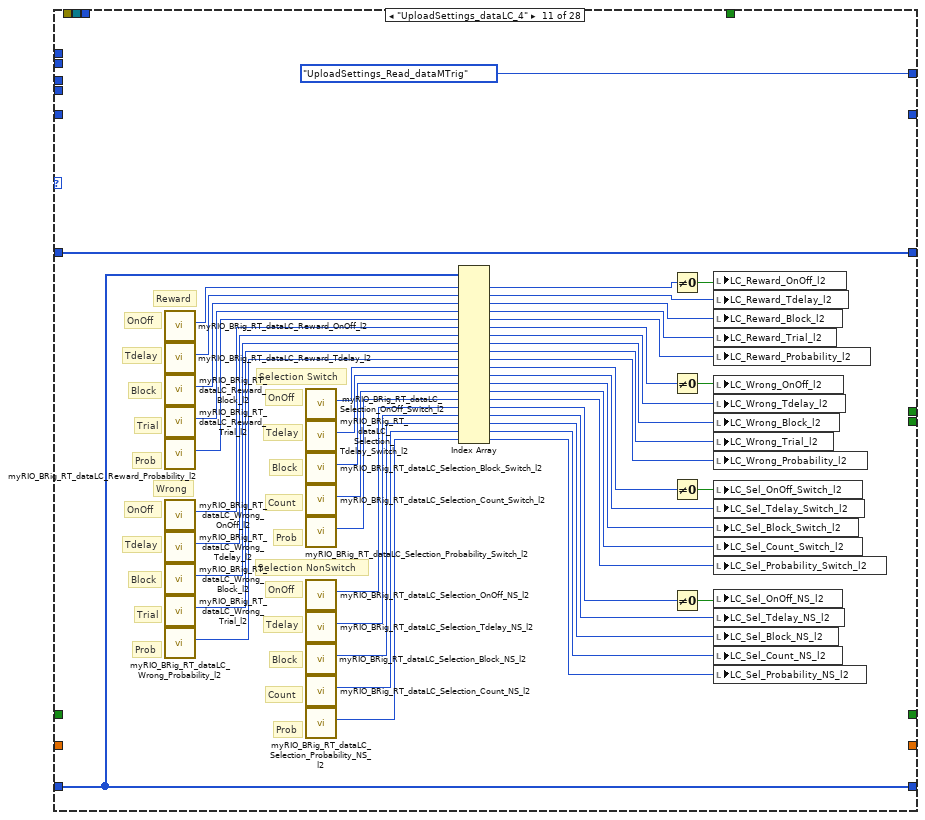
[diagram p19: hidden frame]
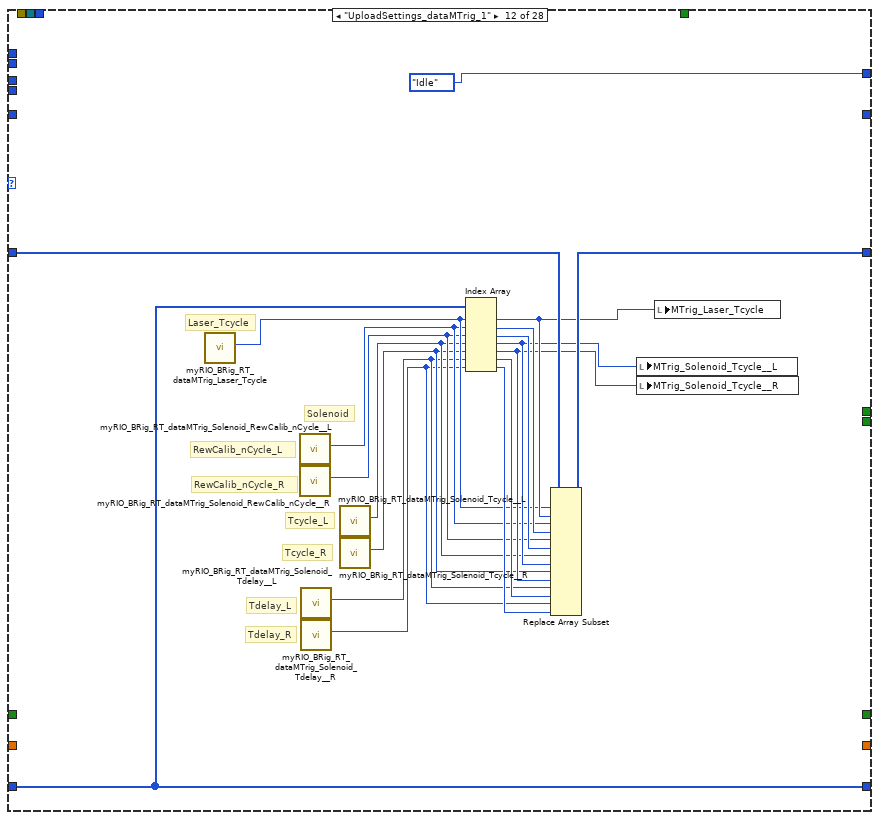
[diagram p20: hidden frame]
diagram:
  w17 = u32 0
  w1 = FALSE
  # "Does the myRIO\nhave it's transfer\nfolder?"
  # "C DIO0 = Left\nC DIO1 = Right"
  # "Start FPGA"
  # "Disconnect from FPGA and reset myRIO"
  n1 = local write "Connected To Host?"(w1) -> ()
  n2 = local write "START"(w1) -> ()
  n3 = local write "STOP_abort"(w1) -> ()
  n4 = local write "STOP_endBlock"(w1) -> ()
  n5 = local write "STOP_endTrial"(w1) -> ()
  n6 = local write "MTrig_Audio_trig__L"(w1) -> ()
  n7 = local write "MTrig_Audio_trig__R"(w1) -> ()
  n8 = local write "MTrig_Solenoid_trig__L"(w1) -> ()
  n9 = local write "MTrig_Solenoid_trig__R"(w1) -> ()
  n10 = local write "MTrig_Laser_trig"(w1) -> ()
  n11 = local write "RewCalib_Trig_R"(w1) -> ()
  n12 = local write "RewCalib_Trig_L"(w1) -> ()
  n13 = local write "Recording"(w1) -> ()
  n14 = call "myRIO_BRig_RT_comm_webdav_myrioFolder.vi"() -> ("output_myrioFolder"=w14:string)  [unwired: 11 in]
  n15 = call "myRIO_BRig_generic_pathExists_fast_stringInput.vi"("input_filePath"=w14) -> ("output_error"=w13:errorcluster, "output_Iexist"=w12:bool, "output_filePath"=w11:path)  [unwired: 8 in]
  n16 = case shown="True" w12 {
    tunnel: w11 -> [w26 _]
    tunnel: w13 -> [w25 w28]
    tunnel: [w24 w27] -> w9
    frame False {
      # "Create it"
      n17 = Create Folder(path (use dialog)=w26, error in=w25) -> (error out=w24:errorcluster)  [unwired: 1 in, 2 out]
    }
    frame True {
      # "Check for\nprevious\nsettings"
      n18 = call "test_myRio_reloadPrevSettings.vi"("input_error"=w28) -> ("output_error"=w27:errorcluster)  [unwired: 10 in]
    }
  }
  n19 = xnode "Open FPGA VI Reference"("error in"=w9) -> ("FPGA VI Reference Out"=w19:refnum<k20>, "error out"=w18:errorcluster)  [unwired: 1 in]
  n20 = call "myRIO__TCP_connect_forWriting.vi"("input_error"=errorcluster {"status"=FALSE, "code"=0, "source"=""}) -> ("output_error"=w7:errorcluster, "output_connected"=w6:bool, "output_hTCP"=w10:refnum<k5>)  [unwired: 8 in]
  "I_connect_TCP" <- w6
  n21 = local write "get_countPerMS"(TRUE ("get_countPerMS")) -> ()
  n22 = while {
    tunnel: w19 -> [w38]
    tunnel: w18 -> [w43]
    tunnel: w17 -> [w46]
    tunnel: w17 -> [w45]
    tunnel: [w36] -> w16
    tunnel: [w35] -> w15
    shift-right: [w32] -> w5
    shift-left: w6 -> [w33]
    tunnel: w7 -> [w31]
    shift-right: [w30] -> w4
    shift-left: w10 -> [w34]
    tunnel: [w29] -> w3
    stop <- w44 stop-if-true
    # "Experiment or\nNonExperiment?"
    # "This loop allows for running multiple experiments in one session"
    n23 = xnode "Read/Write Control"("FPGA VI Reference In"=w38, "error in"=w43, "Counts_Reset"=TRUE) -> ("FPGA VI Reference Out"=w40:refnum<k20>, "error out"=w41:errorcluster)
    n24 = xnode "Read/Write Control"("FPGA VI Reference In"=w40, "error in"=w41, "Counts_Reset"=FALSE) -> ("FPGA VI Reference Out"=w37:refnum<k20>, "error out"=w39:errorcluster)
    n25 = case shown="False" "START" {
      tunnel: w46 -> [w67 w1434]
      tunnel: w45 -> [w66 w1433]
      tunnel: w39 -> [w64 w1368]
      tunnel: w37 -> [w65 w1369]
      tunnel: [w62 w1430] -> w36
      tunnel: [w60 w1425] -> w35
      tunnel: w34 -> [w53 w1379]
      tunnel: [w51 w1383] -> w30
      tunnel: w33 -> [w52 w1381]
      tunnel: [w50 w1382] -> w32
      tunnel: w31 -> [w54 w1380]
      tunnel: [w49 w1378] -> w29
      frame False {
        w57 = FALSE
        # "generic data array\n\nused as storage during\nUploadSettings"
        # "timer for UploadSettings"
        # "initialize dataMTrig"
        # "NonExperiment"
        n26 = case shown="False" w52 {
          selector: w52 -> [_ w76]
          tunnel: w54 -> [w73 w78]
          tunnel: [w74 w78] -> w49
          tunnel: w53 -> [_ w77]
          tunnel: [w75 w77] -> w51
          tunnel: [w72 w76] -> w50
          frame False {
            n27 = call "myRIO__TCP_connect_forWriting.vi"("input_error"=w73) -> ("output_error"=w74:errorcluster, "output_connected"=w72:bool, "output_hTCP"=w75:refnum<k5>)  [unwired: 8 in]
          }
          frame True {
          }
        }
        n28 = call "myRIO_BRig_RT_dataMTrig_init.vi"() -> ("output_dataMTrig"=w68:u16[])  [unwired: 5 in]
        n29 = node-c288() -> (w71:T3)  [unwired: 4 in]
        n30 = timed-loop {
          timing: w71 -> [_]
          timing-out: [_] -> w70
          shift-right: [w117] -> _
          shift-left: w68 -> [w129]
          shift-right: [w111] -> _
          shift-left: myRIO_BRig_RT__Case_NonExp_stateList."Init" ("Enum") -> [w123]
          shift-right: [w105] -> _
          shift-left: w67 -> [w106]
          shift-right: [w103] -> _
          shift-left: w66 -> [w104]
          tunnel: [w125] -> w63
          tunnel: [w124] -> w61
          tunnel: w64 -> [w127]
          tunnel: w65 -> [w126]
          shift-right: [w122] -> _
          shift-left: u16[] [] ("output_data") -> [w121]
          shift-right: [w107] -> _
          shift-left: u16 0 ("Audio_Amp__L") -> [w108]
          shift-right: [w100] -> _
          shift-left: w57 -> [w102]
          shift-right: [w99] -> _
          shift-left: w57 -> [w101]
          shift-right: [w95] -> _
          shift-left: FALSE -> [w96]
          shift-right: [w93] -> _
          shift-left: 0.0 -> [w94]
          stop <- w130 stop-if-true
          # "Laser 2"
          # "Laser 1"
          # "Handles manual triggering\nof audio and lasers"
          n31 = node-c288() -> (w128:i64)  [unwired: 1 in]
          n32 = xnode "Read/Write Control"("FPGA VI Reference In"=w126, "error in"=w127) -> ("FPGA VI Reference Out"=w98:refnum<k20>, "error out"=w97:errorcluster, "A2_LickL"=w105:u32, "A4_LickR"=w103:u32)
          n33 = local write "A2"(w105) -> ()
          n34 = local write "A4"(w103) -> ()
          n35 = case shown="\"Cue\"" w123 {
            selector: w123 -> [_ w155 _ _ _ _ _ _ _ _ _ _ _ _ _ _ _ _ _ w1040 _ _ w1247 _ _ _ w1320 w1361]
            tunnel: [myRIO_BRig_RT__Case_NonExp_stateList."Idle" ("Enum") w153 w160 w179 w198 myRIO_BRig_RT__Case_NonExp_stateList."UploadSettings_dataExp_2" ("Enum") myRIO_BRig_RT__Case_NonExp_stateList."UploadSettings_Read_dataLC" ("Enum") myRIO_BRig_RT__Case_NonExp_stateList."UploadSettings_dataLC_2" ("Enum") myRIO_BRig_RT__Case_NonExp_stateList."UploadSettings_dataLC_4" ("Enum") myRIO_BRig_RT__Case_NonExp_stateList."UploadSettings_dataLC_3" ("f") myRIO_BRig_RT__Case_NonExp_stateList."UploadSettings_Read_dataMTrig" ("f") myRIO_BRig_RT__Case_NonExp_stateList."Idle" ("Enum") w619 w655 myRIO_BRig_RT__Case_NonExp_stateList."Idle_5" ("Enum") w728 w847 w976 myRIO_BRig_RT__Case_NonExp_stateList."Cue" ("t") w1035 myRIO_BRig_RT__Case_NonExp_stateList."DispenseWater_pre" ("Enum") w1193 w1245 w1267 myRIO_BRig_RT__Case_NonExp_stateList."Idle" ("Enum") myRIO_BRig_RT__Case_NonExp_stateList."Idle" ("Enum") w1319 w1361] -> w112
            tunnel: [w143 w152 w170 w189 w208 w284 w368 w421 w480 w533 w580 w596 w623 w670 w714 w733 w851 w974 w1012 w1041 w1104 w1230 w1252 w1278 w1312 w1317 w1329 w1359] -> w118
            tunnel: [_ _ _ _ _ _ _ _ _ _ _ _ _ _ _ _ _ _ _ _ _ _ _ _ _ _ _ TRUE] -> w130
            tunnel: w129 -> [_ w152 w170 w189 w208 w284 w368 w421 w480 w533 w580 w597 w622 w670 w714 w734 w852 w974 w1013 w1042 w1090 w1226 w1253 w1279 w1312 w1317 w1329 w1359]
            tunnel: w128 -> [_ _ _ _ _ _ _ _ _ _ _ _ _ _ _ _ _ _ _ _ _ _ w1257 _ _ _ _ _]
            tunnel: [_ _ w161 w180 w199 w249 w366 w422 w481 w529 w576 w581 _ _ _ _ _ _ w1004 _ _ _ _ _ _ _ _ _] -> w122
            tunnel: w121 -> [_ _ w162 w181 w200 w249 w366 w422 w481 w529 w576 w581 _ _ _ _ _ _ _ _ _ _ _ _ _ _ _ _]
            tunnel: [_ _ _ _ _ _ _ _ _ _ _ _ _ _ _ _ _ _ _ _ _ _ w1254 _ _ _ _ _] -> w120
            tunnel: [_ _ _ _ _ _ _ _ _ _ _ _ _ _ _ _ _ _ _ _ _ _ w1236 _ _ _ _ _] -> w119
            tunnel: w108 -> [_ w159 _ _ _ _ _ _ _ _ _ _ _ _ _ _ _ _ _ _ _ _ _ _ _ _ _ _]
            tunnel: [_ w158 _ _ _ _ _ _ _ _ _ _ _ _ _ _ _ _ _ _ _ _ _ _ _ _ _ _] -> w107
            tunnel: w106 -> [_ _ _ _ _ _ _ _ _ _ _ _ _ _ _ _ _ _ _ w1046 _ _ _ _ _ _ _ _]
            tunnel: w105 -> [_ _ _ _ _ _ _ _ _ _ _ _ _ _ _ _ _ _ _ w1047 _ _ _ _ _ _ _ _]
            tunnel: w104 -> [_ _ _ _ _ _ _ _ _ _ _ _ _ _ _ _ _ _ _ w1044 _ _ _ _ _ _ _ _]
            tunnel: w103 -> [_ _ _ _ _ _ _ _ _ _ _ _ _ _ _ _ _ _ _ w1045 _ _ _ _ _ _ _ _]
            tunnel: w102 -> [_ _ _ _ _ _ _ _ _ _ _ _ _ _ _ _ _ _ _ w1032 _ _ _ _ _ _ _ _]
            tunnel: w101 -> [_ _ _ _ _ _ _ _ _ _ _ _ _ _ _ _ _ _ _ w1031 _ _ _ _ _ _ _ _]
            tunnel: [_ _ _ _ _ _ _ _ _ _ _ _ _ _ _ _ _ _ w1006 w1032 _ _ _ _ _ _ _ _] -> w100
            tunnel: [_ _ _ _ _ _ _ _ _ _ _ _ _ _ _ _ _ _ w1005 w1031 _ _ _ _ _ _ _ _] -> w99
            tunnel: w98 -> [_ _ _ _ _ _ _ _ _ _ _ _ w612 w628 w716 _ _ _ _ _ _ _ _ _ _ _ w1324 _]
            tunnel: w97 -> [_ _ _ _ _ _ _ _ _ _ _ _ w611 w629 w715 _ _ _ _ _ _ _ _ _ _ _ w1323 _]
            tunnel: w96 -> [_ _ _ _ _ _ _ _ _ _ _ _ _ _ _ _ _ _ _ _ _ _ _ _ _ _ w1328 _]
            tunnel: [_ _ _ _ _ _ _ _ _ _ _ _ _ _ _ _ _ _ _ _ _ _ _ _ _ _ TRUE _] -> w95
            tunnel: w94 -> [_ _ _ _ _ _ _ _ _ _ _ _ _ _ _ _ _ _ _ _ _ _ _ _ _ _ w1326 _]
            tunnel: [_ _ _ _ _ _ _ _ _ _ _ _ _ _ _ _ _ _ _ _ _ _ _ _ _ _ w1325 _] -> w93
            frame "Init", Default {
              w134 = FALSE ("RewCalib_Trig_L")
              w135 = u16 100 ("new element/subarray")
              # "Only happens at start of NonExperiment Case"
              # "Tdelay_R"
              # "Tdelay_L"
              # "RewCalib_N__R"
              # "RewCalib_N__L"
              # "Solenoid_Tcycle_R"
              # "Solenoid_Tcycle_L"
              # "Laser_Tcycle"
              # "Audio_Tcycle_R"
              # "Audio_Tcycle_L"
              # "initialize dataMTrig"
              n36 = local write "RewCalib_Trig_L"(w134) -> ()
              n37 = local write "RewCalib_Trig_R"(w134) -> ()
              n38 = local write "MTrig_Audio_trig__L"(w134) -> ()
              n39 = local write "MTrig_Audio_trig__R"(w134) -> ()
              n40 = local write "MTrig_Laser_trig"(w134) -> ()
              n41 = local write "MTrig_Solenoid_trig__L"(w134) -> ()
              n42 = local write "MTrig_Solenoid_trig__R"(w134) -> ()
              n43 = local write "MTrig_CueLed"(w134) -> ()
              n44 = call "myRIO_BRig_RT_dataMTrig_Solenoid_Tcycle__L.vi"() -> ("output_Solenoid_Tcycle__L"=w145:i32)  [unwired: 11 in]
              n45 = call "myRIO_BRig_RT_dataMTrig_Solenoid_Tcycle__R.vi"() -> ("output_Solenoid_Tcycle__R"=w146:i32)  [unwired: 11 in]
              n46 = call "myRIO_BRig_RT_dataMTrig_Audio_Tcycle__L.vi"() -> ("output_Audio_Tcycle__L"=w147:i32)  [unwired: 11 in]
              n47 = call "myRIO_BRig_RT_dataMTrig_Audio_Tcycle__R.vi"() -> ("output_Audio_Tcycle__R"=w148:i32)  [unwired: 11 in]
              n48 = call "myRIO_BRig_RT_dataMTrig_Laser_Tcycle.vi"() -> ("output_Laser_Tcycle"=w149:i32)  [unwired: 11 in]
              n49 = call "myRIO_BRig_RT_dataMTrig_Solenoid_RewCalib_nCycle__L.vi"() -> ("output_Solenoid_RewCalib_nCycle__L"=w141:i32)  [unwired: 11 in]
              n50 = call "myRIO_BRig_RT_dataMTrig_Solenoid_RewCalib_nCycle__R.vi"() -> ("output_Solenoid_RewCalib_nCycle__R"=w140:i32)  [unwired: 11 in]
              n51 = call "myRIO_BRig_RT_dataMTrig_Solenoid_Tdelay__L.vi"() -> ("output_Solenoid_Tdelay__L"=w139:i32)  [unwired: 11 in]
              n52 = call "myRIO_BRig_RT_dataMTrig_Solenoid_Tdelay__R.vi"() -> ("output_Solenoid_Tdelay__R"=w138:i32)  [unwired: 11 in]
              n53 = call "myRIO_BRig_RT_dataMTrig_CueLed_Tcycle.vi"() -> ("output_CueLed_Tcycle"=w133:i32)  [unwired: 11 in]
              n54 = local read "MTrig_Solenoid_Tcycle__L"() -> (w150:u16)
              n55 = local read "MTrig_Solenoid_Tcycle__R"() -> (w151:u16)
              n56 = local read "MTrig_Laser_Tcycle"() -> (w136:u16)
              n57 = call "myRIO_BRig_RT_dataMTrig_init.vi"() -> ("output_dataMTrig"=w144:u16[])  [unwired: 5 in]
              n58 = local read "Tcycle_Cue_LED_min"() -> (w132:u16)
              n59 = local read "Tcycle_Cue_Audio_min"() -> (w137:u16)
              n60 = Replace Array Subset(array=w144, new element #1=w150, index #1=w145, new element #2=w151, index #2=w146, new element #3=w137, index #3=w147, new element #4=w137, index #4=w148, new element #5=w136, index #5=w149, new element #6=w135, index #6=w141, new element #7=w135, index #7=w140, new element #8=w135, index #8=w139, new element #9=w135, index #9=w138, new element #10=w132, index #10=w133) -> (w143:u16[])
            }
            frame "UploadSettings_pre" {
              # "When the Host sends settings,\nnot all files send at the same time.\n\nIf RT reads the settings faster\nthan the Host can send them,\nthen we will skip settings.\n\nSolution:\nWait 20 cycles"
              n61 = Increment(x=w159) -> (x+1=w158:u16)
              n62 = Greater?(x=w158, y=u16 20) -> (0:w156:bool)
              n63 = Select(t=myRIO_BRig_RT__Case_NonExp_stateList."UploadSettings_Read_dataExp", s=w156, f=w155) -> (s? t:f=w153:T1)
            }
            frame "UploadSettings_Read_dataExp" {
              # "Grab data but do not act on it yet"
              # "grab dataExp and\nstore it in the\ngeneric data array"
              # "dataExp"
              n64 = call "myRIO_BRig_RT_dataExp_init_details.vi"() -> ("output_dataSize"=w166:i32, "output_dataName"=w169:string)  [unwired: 10 in]
              n65 = call "myRIO_BRig_RT_comm_webdav_uploadReceived_check.vi"("input_dataName"=w169) -> ("output_Iexist"=w168:bool, "output_dataPath"=w167:path)  [unwired: 9 in]
              n66 = case shown="True" w168 {
                tunnel: w167 -> [_ w178]
                tunnel: w166 -> [_ w177]
                tunnel: [_ w176] -> w165
                tunnel: w162 -> [w171 w175]
                tunnel: [w171 w172] -> w161
                frame False {
                }
                frame True {
                  n67 = call "myRIO_BRig_RT_comm_webdav_uploadReceived_read.vi"("input_dataSize"=w177, "input_filePath"=w178) -> ("output_Ivalid"=w176:bool, "output_data"=w174:i64[])  [unwired: 8 in]
                  n68 = To Unsigned Word Integer(number=w174) -> (unsigned 16bit integer=w173:u16[])
                  n69 = Select(t=w173, s=w176, f=w175) -> (s? t:f=w172:u16[])
                }
              }
              n70 = Select(t=myRIO_BRig_RT__Case_NonExp_stateList."UploadSettings_dataExp_1", s=w165, f=myRIO_BRig_RT__Case_NonExp_stateList."UploadSettings_Read_dataLC" ("t")) -> (s? t:f=w160:T1)
            }
            frame "UploadSettings_Read_dataLC" {
              # "Grab data but do not act on it yet"
              # "grab dataLC and\nstore it in the\ngeneric data array"
              # "dataLC"
              n71 = call "myRIO_BRig_RT_dataLC_init_details.vi"() -> ("output_dataSize"=w185:i32, "output_dataName"=w188:string)  [unwired: 10 in]
              n72 = call "myRIO_BRig_RT_comm_webdav_uploadReceived_check.vi"("input_dataName"=w188) -> ("output_Iexist"=w187:bool, "output_dataPath"=w186:path)  [unwired: 9 in]
              n73 = case shown="True" w187 {
                tunnel: w186 -> [_ w197]
                tunnel: w185 -> [_ w196]
                tunnel: [_ w195] -> w184
                tunnel: w181 -> [w190 w194]
                tunnel: [w190 w191] -> w180
                frame False {
                }
                frame True {
                  n74 = call "myRIO_BRig_RT_comm_webdav_uploadReceived_read.vi"("input_dataSize"=w196, "input_filePath"=w197) -> ("output_Ivalid"=w195:bool, "output_data"=w193:i64[])  [unwired: 8 in]
                  n75 = To Unsigned Word Integer(number=w193) -> (unsigned 16bit integer=w192:u16[])
                  n76 = Select(t=w192, s=w195, f=w194) -> (s? t:f=w191:u16[])
                }
              }
              n77 = Select(t=myRIO_BRig_RT__Case_NonExp_stateList."UploadSettings_dataLC_1", s=w184, f=myRIO_BRig_RT__Case_NonExp_stateList."UploadSettings_Read_dataMTrig" ("t")) -> (s? t:f=w179:T1)
            }
            frame "UploadSettings_Read_dataMTrig" {
              # "Grab data but do not act on it yet"
              # "grab dataMTrig and\nstore it in the\ngeneric data array"
              # "dataMTrig"
              n78 = call "myRIO_BRig_RT_dataMTrig_init_details.vi"() -> ("output_dataSize"=w204:i32, "output_dataName"=w207:string)  [unwired: 10 in]
              n79 = call "myRIO_BRig_RT_comm_webdav_uploadReceived_check.vi"("input_dataName"=w207) -> ("output_Iexist"=w206:bool, "output_dataPath"=w205:path)  [unwired: 9 in]
              n80 = case shown="True" w206 {
                tunnel: w205 -> [_ w216]
                tunnel: w204 -> [_ w215]
                tunnel: [_ w214] -> w203
                tunnel: w200 -> [w209 w213]
                tunnel: [w209 w210] -> w199
                frame False {
                }
                frame True {
                  n81 = call "myRIO_BRig_RT_comm_webdav_uploadReceived_read.vi"("input_dataSize"=w215, "input_filePath"=w216) -> ("output_Ivalid"=w214:bool, "output_data"=w212:i64[])  [unwired: 8 in]
                  n82 = To Unsigned Word Integer(number=w212) -> (unsigned 16bit integer=w211:u16[])
                  n83 = Select(t=w211, s=w214, f=w213) -> (s? t:f=w210:u16[])
                }
              }
              n84 = Select(t=myRIO_BRig_RT__Case_NonExp_stateList."UploadSettings_dataMTrig_1", s=w203, f=myRIO_BRig_RT__Case_NonExp_stateList."Idle" ("t")) -> (s? t:f=w198:T1)
            }
            frame "UploadSettings_dataExp_1" {
              # "Cue_max"
              # "Cue_min"
              # "CuePenalty"
              # "Timeout"
              # "Wrong"
              # "Selection"
              # "RewardPost"
              # "Tcycle"
              # "TPB_min_R"
              # "TPB_min_L"
              # "TPB_max_R"
              # "TPB_max_L"
              # "I_trialUntilReward"
              # "ENL_penalty"
              # "ENL_min"
              # "ENL_max"
              # "BUR_max"
              # "BUR_min"
              # "CueCycles"
              # "Audio_Freq_R"
              # "Audio_Freq_L"
              # "Audio_Amp_R"
              # "Audio_Amp_L"
              n85 = call "myRIO_BRig_RT_dataExp_Tcycle_Reward_min_L.vi"() -> ("output_Tcycle_Reward_min_L"=w228:i32)  [unwired: 11 in]
              n86 = call "myRIO_BRig_RT_dataExp_Tcycle_Reward_max_L.vi"() -> ("output_Tcycle_Reward_max_L"=w227:i32)  [unwired: 11 in]
              n87 = call "myRIO_BRig_RT_dataExp_Tcycle_Reward_step_L.vi"() -> ("output_Tcycle_Reward_step_L"=w226:i32)  [unwired: 11 in]
              n88 = call "myRIO_BRig_RT_dataExp_Tcycle_RewardPost.vi"() -> ("output_Tcycle_RewardPost"=w248:i32)  [unwired: 11 in]
              n89 = call "myRIO_BRig_RT_dataExp_CueCycles.vi"() -> ("output_CueCycles"=w276:i32)  [unwired: 11 in]
              n90 = call "myRIO_BRig_RT_dataExp_Audio_amp__R.vi"() -> ("output_Audio_amp__R"=w280:i32)  [unwired: 11 in]
              n91 = call "myRIO_BRig_RT_dataExp_Audio_amp__L.vi"() -> ("output_Audio_amp__L"=w282:i32)  [unwired: 11 in]
              n92 = call "myRIO_BRig_RT_dataExp_BUR_min.vi"() -> ("output_BUR_min"=w273:i32)  [unwired: 11 in]
              n93 = call "myRIO_BRig_RT_dataExp_ENL_min.vi"() -> ("output_ENL_min"=w269:i32)  [unwired: 11 in]
              n94 = call "myRIO_BRig_RT_dataExp_TPB_max__L.vi"() -> ("output_TPB_max__L"=w261:i32)  [unwired: 11 in]
              n95 = call "myRIO_BRig_RT_dataExp_TPB_max__R.vi"() -> ("output_TPB_max__R"=w260:i32)  [unwired: 11 in]
              n96 = call "myRIO_BRig_RT_dataExp_Tcycle_Reward_min_R.vi"() -> ("output_Tcycle_Reward_min_R"=w225:i32)  [unwired: 11 in]
              n97 = call "myRIO_BRig_RT_dataExp_Tcycle_Reward_max_R.vi"() -> ("output_Tcycle_Reward_max_R"=w224:i32)  [unwired: 11 in]
              n98 = call "myRIO_BRig_RT_dataExp_Tcycle_Reward_step_R.vi"() -> ("output_Tcycle_Reward_step_R"=w223:i32)  [unwired: 11 in]
              n99 = call "myRIO_BRig_RT_dataExp_ENL_penalty.vi"() -> ("output_ENL_penalty"=w268:i32)  [unwired: 11 in]
              n100 = call "myRIO_BRig_RT_dataExp_Tcycle_Selection.vi"() -> ("output_Tcycle_Selection"=w247:i32)  [unwired: 11 in]
              n101 = call "myRIO_BRig_RT_dataExp_Tcycle_Wrong.vi"() -> ("output_Tcycle_Wrong"=w246:i32)  [unwired: 11 in]
              n102 = call "myRIO_BRig_RT_dataExp_Tcycle_Timeout.vi"() -> ("output_Tcycle_Timeout"=w242:i32)  [unwired: 11 in]
              n103 = call "myRIO_BRig_RT_dataExp_Audio_freq__L.vi"() -> ("output_Audio_freq__L"=w278:i32)  [unwired: 11 in]
              n104 = call "myRIO_BRig_RT_dataExp_Audio_freq__R.vi"() -> ("output_Audio_freq__R"=w277:i32)  [unwired: 11 in]
              n105 = call "myRIO_BRig_RT_dataExp_BUR_max.vi"() -> ("output_BUR_max"=w274:i32)  [unwired: 11 in]
              n106 = call "myRIO_BRig_RT_dataExp_ENL_max.vi"() -> ("output_ENL_max"=w270:i32)  [unwired: 11 in]
              n107 = call "myRIO_BRig_RT_dataExp_ItrialUntilReward.vi"() -> ("output_I_trialUntilReward"=w264:i32)  [unwired: 11 in]
              n108 = call "myRIO_BRig_RT_dataExp_TPB_min__L.vi"() -> ("output_TPB_min__L"=w259:i32)  [unwired: 11 in]
              n109 = call "myRIO_BRig_RT_dataExp_TPB_min__R.vi"() -> ("output_TPB_min__R"=w258:i32)  [unwired: 11 in]
              n110 = call "myRIO_BRig_RT_dataExp_Tcycle_Cue1Penalty_Audio.vi"() -> ("output_Tcycle_Cue1Penalty_Audio"=w240:i32)  [unwired: 11 in]
              n111 = call "myRIO_BRig_RT_dataExp_Tcycle_Cue1_Audio_min.vi"() -> ("output_Tcycle_Cue1_Audio_min"=w238:i32)  [unwired: 11 in]
              n112 = call "myRIO_BRig_RT_dataExp_Tcycle_Cue1_Audio_max.vi"() -> ("output_Tcycle_Cue1_Audio_max"=w236:i32)  [unwired: 11 in]
              n113 = call "myRIO_BRig_RT_dataExp_Tcycle_Cue1Penalty_LED.vi"() -> ("output_Tcycle_Cue1Penalty_LED"=w234:i32)  [unwired: 11 in]
              n114 = call "myRIO_BRig_RT_dataExp_Tcycle_Cue1_LED_min.vi"() -> ("output_Tcycle_Cue1_LED_min"=w233:i32)  [unwired: 11 in]
              n115 = call "myRIO_BRig_RT_dataExp_Tcycle_Cue1_LED_max.vi"() -> ("output_Tcycle_Cue1_LED_max"=w232:i32)  [unwired: 11 in]
              n116 = Index Array(array=w249, index #1=w282, index #2=w280, index #3=w278, index #4=w277, index #5=w276, index #6=w274, index #7=w273, index #8=w270, index #9=w269, index #10=w268, index #11=w264, index #12=w261, index #13=w260, index #14=w259, index #15=w258, index #16=w248, index #17=w247, index #18=w246, index #19=w242, index #20=w240, index #21=w238, index #22=w236, index #23=w234, index #24=w233, index #25=w232, index #26=w228, index #27=w227, index #28=w226, index #29=w225, index #30=w224, index #31=w223) -> (element #1=w281:u16, element #2=w279:u16, element #3=w252:u16, element #4=w251:u16, element #5=w275:u16, element #6=w272:u16, element #7=w271:u16, element #8=w267:u16, element #9=w266:u16, element #10=w265:u16, element #11=w262:u16, element #12=w257:u16, element #13=w256:u16, element #14=w255:u16, element #15=w254:u16, element #16=w245:u16, element #17=w244:u16, element #18=w243:u16, element #19=w241:u16, element #20=w239:u16, element #21=w237:u16, element #22=w235:u16, element #23=w231:u16, element #24=w230:u16, element #25=w229:u16, element #26=w222:u16, element #27=w221:u16, element #28=w220:u16, element #29=w219:u16, element #30=w218:u16, element #31=w217:u16)
              n117 = local write "Tcycle_CuePenalty_LED"(w231) -> ()
              n118 = local write "Tcycle_Cue_LED_min"(w230) -> ()
              n119 = local write "Tcycle_Cue_LED_max"(w229) -> ()
              n120 = local write "Tcycle_Selection"(w244) -> ()
              n121 = local write "Tcycle_Wrong"(w243) -> ()
              n122 = local write "Tcycle_Timeout"(w241) -> ()
              n123 = local write "Audio_Amp__L"(w281) -> ()
              n124 = local write "Audio_Amp__R"(w279) -> ()
              n125 = local write "Tcycle_Reward_min_L"(w222) -> ()
              n126 = local write "Tcycle_Reward_max_L"(w221) -> ()
              n127 = local write "Tcycle_Reward_step_L"(w220) -> ()
              n128 = local write "Tcycle_Reward_min_L"(w219) -> ()
              n129 = local write "Tcycle_Reward_max_L"(w218) -> ()
              n130 = local write "Tcycle_Reward_step_L"(w217) -> ()
              n131 = local write "Tcycle_ENLPenalty"(w265) -> ()
              n132 = local write "Tcycle_ENL_max"(w267) -> ()
              n133 = local write "TpB_Min_L"(w255) -> ()
              n134 = local write "TpB_Min_R"(w254) -> ()
              n135 = local write "Tcycle_CuePenalty_Audio"(w239) -> ()
              n136 = local write "Tcycle_Cue_Audio_min"(w237) -> ()
              n137 = local write "Tcycle_Cue_Audio_max"(w235) -> ()
              n138 = To Unsigned Byte Integer(number=w252) -> (unsigned 8bit integer=w253:u8)
              n139 = To Unsigned Byte Integer(number=w251) -> (unsigned 8bit integer=w250:u8)
              n140 = Not Equal To 0?(x=w262) -> (x != 0?=w263:bool)
              n141 = local write "Tcycle_RewardPost"(w245) -> ()
              n142 = local write "CueCycles"(w275) -> ()
              n143 = local write "BUR_min"(w271) -> ()
              n144 = local write "BUR_max"(w272) -> ()
              n145 = local write "Tcycle_ENL_min"(w266) -> ()
              n146 = local write "TpB_Max_L"(w257) -> ()
              n147 = local write "TpB_Max_R"(w256) -> ()
              n148 = local write "TrialUntilReward"(w263) -> ()
              n149 = local write "Audio_Freq__L"(w253) -> ()
              n150 = local write "Audio_Freq__R"(w250) -> ()
            }
            frame "UploadSettings_dataExp_2" {
              w304 = 100.0 ("y")
              n151 = call "myRIO_BRig_RT_dataExp_FPGA_f_count2ms.vi"() -> ("output_FPGA_f_count2ms"=w365:i32)  [unwired: 11 in]
              n152 = call "myRIO_BRig_RT_dataExp_laser1_Freq.vi"() -> ("output_laser1_Freq"=w353:i32)  [unwired: 11 in]
              n153 = call "myRIO_BRig_RT_dataExp_laser1_duration.vi"() -> ("output_laser1_duration"=w352:i32)  [unwired: 11 in]
              n154 = call "myRIO_BRig_RT_dataExp_laser1_Tpeak.vi"() -> ("output_laser1_Tpeak"=w351:i32)  [unwired: 11 in]
              n155 = call "myRIO_BRig_RT_dataExp_laser1_Tshutter.vi"() -> ("output_laser1_Tshutter"=w350:i32)  [unwired: 11 in]
              n156 = call "myRIO_BRig_RT_dataExp_laser1_Power_min.vi"() -> ("output_laser1_Power_min"=w349:i32)  [unwired: 11 in]
              n157 = call "myRIO_BRig_RT_dataExp_laser1_Power_max.vi"() -> ("output_laser1_Power_max"=w348:i32)  [unwired: 11 in]
              n158 = call "myRIO_BRig_RT_dataExp_laser1_Power_step.vi"() -> ("output_laser1_Power_step"=w347:i32)  [unwired: 11 in]
              n159 = call "myRIO_BRig_RT_dataExp_Cue1Param_CueType_Switch.vi"() -> ("output_Cue1Param_CueType_Switch"=w298:i32)  [unwired: 11 in]
              n160 = call "myRIO_BRig_RT_dataExp_Cue1Param_AudioLed_Count_Switch.vi"() -> ("output_Cue1Param_AudioLed_Count_Switch"=w297:i32)  [unwired: 11 in]
              n161 = call "myRIO_BRig_RT_dataExp_Cue1Param_AudioLed_Probability_Switch.vi"() -> ("output_Cue1Param_AudioLed_Probability_Switch"=w296:i32)  [unwired: 11 in]
              n162 = call "myRIO_BRig_RT_dataExp_SolenoidProbability_L.vi"() -> ("output_SolenoidProbability_L"=w300:i32)  [unwired: 11 in]
              n163 = call "myRIO_BRig_RT_dataExp_SolenoidProbability_R.vi"() -> ("output_SolenoidProbability_R"=w299:i32)  [unwired: 11 in]
              n164 = call "myRIO_BRig_RT_dataExp_Cue1Param_CueType_NS.vi"() -> ("output_Cue1Param_CueType_NS"=w295:i32)  [unwired: 11 in]
              n165 = call "myRIO_BRig_RT_dataExp_Cue1Param_AudioLed_Count_NS.vi"() -> ("output_Cue1Param_AudioLed_Count_NS"=w294:i32)  [unwired: 11 in]
              n166 = call "myRIO_BRig_RT_dataExp_Cue1Param_AudioLed_Probability_NS.vi"() -> ("output_Cue1Param_AudioLed_Probability_NS"=w293:i32)  [unwired: 11 in]
              n167 = call "myRIO_BRig_RT_dataExp_laser2_Freq.vi"() -> ("output_laser2_Freq"=w346:i32)  [unwired: 11 in]
              n168 = call "myRIO_BRig_RT_dataExp_laser2_duration.vi"() -> ("output_laser2_duration"=w345:i32)  [unwired: 11 in]
              n169 = call "myRIO_BRig_RT_dataExp_laser2_Tpeak.vi"() -> ("output_laser2_Tpeak"=w344:i32)  [unwired: 11 in]
              n170 = call "myRIO_BRig_RT_dataExp_laser2_Tshutter.vi"() -> ("output_laser2_Tshutter"=w343:i32)  [unwired: 11 in]
              n171 = call "myRIO_BRig_RT_dataExp_laser2_Power_min.vi"() -> ("output_laser2_Power_min"=w342:i32)  [unwired: 11 in]
              n172 = call "myRIO_BRig_RT_dataExp_laser2_Power_max.vi"() -> ("output_laser2_Power_max"=w341:i32)  [unwired: 11 in]
              n173 = call "myRIO_BRig_RT_dataExp_laser2_Power_step.vi"() -> ("output_laser2_Power_step"=w340:i32)  [unwired: 11 in]
              n174 = call "myRIO_BRig_RT_dataExp_CueLed_Freq.vi"() -> ("output_CueLed_Freq"=w309:i32)  [unwired: 11 in]
              n175 = call "myRIO_BRig_RT_dataExp_CueLed_Tpeak.vi"() -> ("output_CueLed_Tpeak"=w302:i32)  [unwired: 11 in]
              n176 = Index Array(array=w366, index #1=w365, index #2=w353, index #3=w352, index #4=w351, index #5=w350, index #6=w349, index #7=w348, index #8=w347, index #9=w346, index #10=w345, index #11=w344, index #12=w343, index #13=w342, index #14=w341, index #15=w340, index #16=w309, index #17=w302, index #18=w300, index #19=w299, index #20=w298, index #21=w297, index #22=w296, index #23=w295, index #24=w294, index #25=w293) -> (element #1=w364:u16, element #2=w339:u16, element #3=w338:u16, element #4=w337:u16, element #5=w336:u16, element #6=w335:u16, element #7=w325:u16, element #8=w324:u16, element #9=w320:u16, element #10=w319:u16, element #11=w318:u16, element #12=w317:u16, element #13=w316:u16, element #14=w311:u16, element #15=w310:u16, element #16=w303:u16, element #17=w301:u16, element #18=w292:u16, element #19=w291:u16, element #20=w290:u16, element #21=w289:u16, element #22=w288:u16, element #23=w287:u16, element #24=w286:u16, element #25=w285:u16)
              n177 = local write "Cue1Param_CueType_Switch"(w290) -> ()
              n178 = local write "Cue1Param_AudioLed_Count_Switch"(w289) -> ()
              n179 = local write "Cue1Param_AudioLed_Probability_Switch"(w288) -> ()
              n180 = local write "Cue1Param_CueType_NS"(w287) -> ()
              n181 = local write "Cue1Param_AudioLed_Count_NS"(w286) -> ()
              n182 = local write "Cue1Param_AudioLed_Probability_NS"(w285) -> ()
              n183 = To Double Precision Float(number=w364) -> (double precision float=w363:dbl)
              n184 = To Double Precision Float(number=w339) -> (double precision float=w361:dbl)
              n185 = To Double Precision Float(number=w337) -> (double precision float=w358:dbl)
              n186 = To Double Precision Float(number=w336) -> (double precision float=w357:dbl)
              n187 = To Double Precision Float(number=w335) -> (double precision float=w359:dbl)
              n188 = To Double Precision Float(number=w325) -> (double precision float=w330:dbl)
              n189 = To Double Precision Float(number=w324) -> (double precision float=w326:dbl)
              n190 = To Double Precision Float(number=w320) -> (double precision float=w331:dbl)
              n191 = To Double Precision Float(number=w318) -> (double precision float=w333:dbl)
              n192 = To Double Precision Float(number=w317) -> (double precision float=w334:dbl)
              n193 = To Double Precision Float(number=w316) -> (double precision float=w332:dbl)
              n194 = To Double Precision Float(number=w311) -> (double precision float=w314:dbl)
              n195 = To Double Precision Float(number=w310) -> (double precision float=w315:dbl)
              n196 = To Double Precision Float(number=w303) -> (double precision float=w308:dbl)
              n197 = To Double Precision Float(number=w301) -> (double precision float=w307:dbl)
              n198 = local write "SolenoidProbability_L"(w292) -> ()
              n199 = local write "SolenoidProbability_R"(w291) -> ()
              n200 = Divide(x=w363, y=w304) -> (x/y=w362:dbl)
              n201 = Divide(x=w361, y=w304) -> (x/y=w360:dbl)
              n202 = Divide(x=w358, y=w304) -> (x/y=w355:dbl)
              n203 = Divide(x=w357, y=w304) -> (x/y=w354:dbl)
              n204 = Divide(x=w359, y=w304) -> (x/y=w356:dbl)
              n205 = Divide(x=w330, y=w304) -> (x/y=w328:dbl)
              n206 = Divide(x=w326, y=w304) -> (x/y=w327:dbl)
              n207 = Divide(x=w331, y=w304) -> (x/y=w329:dbl)
              n208 = Divide(x=w333, y=w304) -> (x/y=w323:dbl)
              n209 = Divide(x=w334, y=w304) -> (x/y=w322:dbl)
              n210 = Divide(x=w332, y=w304) -> (x/y=w321:dbl)
              n211 = Divide(x=w314, y=w304) -> (x/y=w313:dbl)
              n212 = Divide(x=w315, y=w304) -> (x/y=w312:dbl)
              n213 = Divide(x=w308, y=w304) -> (x/y=w306:dbl)
              n214 = Divide(x=w307, y=w304) -> (x/y=w305:dbl)
              n215 = local write "FPGA_count2ms"(w362) -> ()
              n216 = local write "Laser_Freq_l1"(w360) -> ()
              n217 = local write "Laser_duration_l1"(w338) -> ()
              n218 = local write "Laser_Tpeak_l1"(w355) -> ()
              n219 = local write "Laser_Tshutter_l1"(w354) -> ()
              n220 = local write "Laser_power_min_l1"(w356) -> ()
              n221 = local write "Laser_power_max_l1"(w328) -> ()
              n222 = local write "Laser_power_step_l1"(w327) -> ()
              n223 = local write "Laser_Freq_l2"(w329) -> ()
              n224 = local write "Laser_duration_l2"(w319) -> ()
              n225 = local write "Laser_Tpeak_l2"(w323) -> ()
              n226 = local write "Laser_Tshutter_l2"(w322) -> ()
              n227 = local write "Laser_power_min_l2"(w321) -> ()
              n228 = local write "Laser_power_max_l2"(w313) -> ()
              n229 = local write "Laser_power_step_l2"(w312) -> ()
              n230 = local write "CueLed_Freq"(w306) -> ()
              n231 = local write "CueLed_Tpeak"(w305) -> ()
            }
            frame "UploadSettings_dataLC_1" {
              # "Cue1_delayOpt_NonSwitch"
              # "ENL1_delayOpt_NonSwitch"
              # "Cue1_delayOpt_Switch"
              # "ENL1_delayOpt_Switch"
              # "Count"
              # "Tdelay"
              # "Prob"
              # "OnOff"
              # "Block"
              # "Count"
              # "Tdelay"
              # "Prob"
              # "OnOff"
              # "Block"
              # "Count"
              # "Tdelay"
              # "Prob"
              # "OnOff"
              # "Block"
              # "ENL1 Switch"
              # "Cue1 NonSwitch"
              # "Cue1 Switch"
              # "ENL1 NonSwitch"
              # "Count"
              # "Tdelay"
              # "Prob"
              # "OnOff"
              # "Block"
              n232 = call "myRIO_BRig_RT_dataLC_ENL1_OnOff_Switch_l1.vi"() -> ("output_ENL1_OnOff_Switch_l1"=w420:i32)  [unwired: 11 in]
              n233 = call "myRIO_BRig_RT_dataLC_ENL1_Tdelay_Switch_l1.vi"() -> ("output_ENL1_Tdelay_Switch_l1"=w419:i32)  [unwired: 11 in]
              n234 = call "myRIO_BRig_RT_dataLC_ENL1_Block_Switch_l1.vi"() -> ("output_ENL1_Block_Switch_l1"=w418:i32)  [unwired: 11 in]
              n235 = call "myRIO_BRig_RT_dataLC_ENL1_Count_Switch_l1.vi"() -> ("output_ENL1_Count_Switch_l1"=w417:i32)  [unwired: 11 in]
              n236 = call "myRIO_BRig_RT_dataLC_ENL1_Probability_Switch_l1.vi"() -> ("output_ENL1_Probability_Switch_l1"=w416:i32)  [unwired: 11 in]
              n237 = call "myRIO_BRig_RT_dataLC_ENL1_OnOff_NS_l1.vi"() -> ("output_ENL1_OnOff_NS_l1"=w415:i32)  [unwired: 11 in]
              n238 = call "myRIO_BRig_RT_dataLC_ENL1_Tdelay_NS_l1.vi"() -> ("output_ENL1_Tdelay_NS_l1"=w414:i32)  [unwired: 11 in]
              n239 = call "myRIO_BRig_RT_dataLC_ENL1_Block_NS_l1.vi"() -> ("output_ENL1_All_Block"=w413:i32)  [unwired: 11 in]
              n240 = call "myRIO_BRig_RT_dataLC_ENL1_Count_NS_l1.vi"() -> ("output_ENL1_Count_NS_l1"=w412:i32)  [unwired: 11 in]
              n241 = call "myRIO_BRig_RT_dataLC_ENL1_Probability_NS_l1.vi"() -> ("output_ENL1_Probability_NS_l1"=w411:i32)  [unwired: 11 in]
              n242 = call "myRIO_BRig_RT_dataLC_Cue1_OnOff_Switch_l1.vi"() -> ("output_Cue1_OnOff_Switch_l1"=w410:i32)  [unwired: 11 in]
              n243 = call "myRIO_BRig_RT_dataLC_Cue1_Tdelay_Switch_l1.vi"() -> ("output_Cue1_Tdelay_Switch_l1"=w409:i32)  [unwired: 11 in]
              n244 = call "myRIO_BRig_RT_dataLC_Cue1_Block_Switch_l1.vi"() -> ("output_Cue1_Block_Switch_l1"=w408:i32)  [unwired: 11 in]
              n245 = call "myRIO_BRig_RT_dataLC_Cue1_Count_Switch_l1.vi"() -> ("output_Cue1_Count_Switch_l1"=w407:i32)  [unwired: 11 in]
              n246 = call "myRIO_BRig_RT_dataLC_Cue1_Probability_Switch_l1.vi"() -> ("output_Cue1_Probability_Switch_l1"=w406:i32)  [unwired: 11 in]
              n247 = call "myRIO_BRig_RT_dataLC_Cue1_OnOff_NS_l1.vi"() -> ("output_Cue1_OnOff_NS_l1"=w405:i32)  [unwired: 11 in]
              n248 = call "myRIO_BRig_RT_dataLC_Cue1_Tdelay_NS_l1.vi"() -> ("output_Cue1_Tdelay_NS_l1"=w404:i32)  [unwired: 11 in]
              n249 = call "myRIO_BRig_RT_dataLC_Cue1_Block_NS_l1.vi"() -> ("output_Cue1_Block_NS_l1"=w403:i32)  [unwired: 11 in]
              n250 = call "myRIO_BRig_RT_dataLC_Cue1_Count_NS_l1.vi"() -> ("output_Cue1_Count_NS_l1"=w402:i32)  [unwired: 11 in]
              n251 = call "myRIO_BRig_RT_dataLC_Cue1_Probability_NS_l1.vi"() -> ("output_Cue1_l1_All_Probability"=w401:i32)  [unwired: 11 in]
              n252 = call "myRIO_BRig_RT_dataLC_ENL1_delayOpt_Switch_l1.vi"() -> ("output_ENL1_delayOpt_Switch_l1"=w380:i32)  [unwired: 11 in]
              n253 = call "myRIO_BRig_RT_dataLC_ENL1_delayOpt_NS_l1.vi"() -> ("output_ENL1_delayOpt_NS_l1"=w379:i32)  [unwired: 11 in]
              n254 = call "myRIO_BRig_RT_dataLC_Cue1_delayOpt_Switch_l1.vi"() -> ("output_Cue1_delayOpt_Switch_l1"=w378:i32)  [unwired: 11 in]
              n255 = call "myRIO_BRig_RT_dataLC_Cue1_delayOpt_NS_l1.vi"() -> ("output_Cue1_delayOpt_NS_l1"=w377:i32)  [unwired: 11 in]
              n256 = Index Array(array=w422, index #1=w420, index #2=w419, index #3=w418, index #4=w417, index #5=w416, index #6=w415, index #7=w414, index #8=w413, index #9=w412, index #10=w411, index #11=w410, index #12=w409, index #13=w408, index #14=w407, index #15=w406, index #16=w405, index #17=w404, index #18=w403, index #19=w402, index #20=w401, index #21=w380, index #22=w379, index #23=w378, index #24=w377) -> (element #1=w400:u16, element #2=w399:u16, element #3=w398:u16, element #4=w397:u16, element #5=w396:u16, element #6=w395:u16, element #7=w394:u16, element #8=w393:u16, element #9=w392:u16, element #10=w391:u16, element #11=w390:u16, element #12=w389:u16, element #13=w388:u16, element #14=w387:u16, element #15=w386:u16, element #16=w385:u16, element #17=w384:u16, element #18=w383:u16, element #19=w382:u16, element #20=w381:u16, element #21=w372:u16, element #22=w371:u16, element #23=w370:u16, element #24=w369:u16)
              n257 = Not Equal To 0?(x=w400) -> (x != 0?=w424:bool)
              n258 = Not Equal To 0?(x=w395) -> (x != 0?=w423:bool)
              n259 = Not Equal To 0?(x=w390) -> (x != 0?=w426:bool)
              n260 = Not Equal To 0?(x=w385) -> (x != 0?=w425:bool)
              n261 = Not Equal To 0?(x=w372) -> (x != 0?=w374:bool)
              n262 = Not Equal To 0?(x=w371) -> (x != 0?=w375:bool)
              n263 = Not Equal To 0?(x=w370) -> (x != 0?=w376:bool)
              n264 = Not Equal To 0?(x=w369) -> (x != 0?=w373:bool)
              n265 = local write "LC_ENL1_OnOff_Switch_l1"(w424) -> ()
              n266 = local write "LC_ENL1_Tdelay_Switch_l1"(w399) -> ()
              n267 = local write "LC_ENL1_Block_Switch_l1"(w398) -> ()
              n268 = local write "LC_ENL1_Count_Switch_l1"(w397) -> ()
              n269 = local write "LC_ENL1_Probability_Switch_l1"(w396) -> ()
              n270 = local write "LC_ENL1_OnOff_NS_l1"(w423) -> ()
              n271 = local write "LC_ENL1_Tdelay_NS_l1"(w394) -> ()
              n272 = local write "LC_ENL1_Block_NS_l1"(w393) -> ()
              n273 = local write "LC_ENL1_Count_NS_l1"(w392) -> ()
              n274 = local write "LC_ENL1_Probability_NS_l1"(w391) -> ()
              n275 = local write "LC_Cue1_OnOff_Switch_l1"(w426) -> ()
              n276 = local write "LC_Cue1_Tdelay_Switch_l1"(w389) -> ()
              n277 = local write "LC_Cue1_Block_Switch_l1"(w388) -> ()
              n278 = local write "LC_Cue1_Count_Switch_l1"(w387) -> ()
              n279 = local write "LC_Cue1_Probability_Switch_l1"(w386) -> ()
              n280 = local write "LC_Cue1_OnOff_NS_l1"(w425) -> ()
              n281 = local write "LC_Cue1_Tdelay_NS_l1"(w384) -> ()
              n282 = local write "LC_Cue1_Block_NS_l1"(w383) -> ()
              n283 = local write "LC_Cue1_Count_NS_l1"(w382) -> ()
              n284 = local write "LC_Cue1_Probability_NS_l1"(w381) -> ()
              n285 = local write "LC_ENL1_delayOpt_Switch_l1"(w374) -> ()
              n286 = local write "LC_ENL1_delayOpt_NS_l1"(w375) -> ()
              n287 = local write "LC_Cue1_delayOpt_Switch_l1"(w376) -> ()
              n288 = local write "LC_Cue1_delayOpt_NS_l1"(w373) -> ()
            }
            frame "UploadSettings_dataLC_3" {
              # "Cue1_delayOpt_NonSwitch"
              # "ENL1_delayOpt_NonSwitch"
              # "Cue1_delayOpt_Switch"
              # "ENL1_delayOpt_Switch"
              # "Count"
              # "Tdelay"
              # "Prob"
              # "OnOff"
              # "Block"
              # "Count"
              # "Tdelay"
              # "Prob"
              # "OnOff"
              # "Block"
              # "Count"
              # "Tdelay"
              # "Prob"
              # "OnOff"
              # "Block"
              # "ENL1 Switch"
              # "Cue1 NonSwitch"
              # "Cue1 Switch"
              # "ENL1 NonSwitch"
              # "Count"
              # "Tdelay"
              # "Prob"
              # "OnOff"
              # "Block"
              n289 = call "myRIO_BRig_RT_dataLC_ENL1_OnOff_Switch_l2.vi"() -> ("output_ENL1_OnOff_Switch_l2"=w447:i32)  [unwired: 11 in]
              n290 = call "myRIO_BRig_RT_dataLC_ENL1_Tdelay_Switch_l2.vi"() -> ("output_ENL1_Tdelay_Switch_l2"=w448:i32)  [unwired: 11 in]
              n291 = call "myRIO_BRig_RT_dataLC_ENL1_Block_Switch_l2.vi"() -> ("output_ENL1_Block_Switch_l2"=w449:i32)  [unwired: 11 in]
              n292 = call "myRIO_BRig_RT_dataLC_ENL1_Count_Switch_l2.vi"() -> ("output_ENL1_Count_Switch_l2"=w450:i32)  [unwired: 11 in]
              n293 = call "myRIO_BRig_RT_dataLC_ENL1_Probability_Switch_l2.vi"() -> ("output_ENL1_Probability_Switch_l2"=w451:i32)  [unwired: 11 in]
              n294 = call "myRIO_BRig_RT_dataLC_ENL1_OnOff_NS_l2.vi"() -> ("output_ENL1_OnOff_NS_l2"=w442:i32)  [unwired: 11 in]
              n295 = call "myRIO_BRig_RT_dataLC_ENL1_Tdelay_NS_l2.vi"() -> ("output_ENL1_Tdelay_NS_l2"=w443:i32)  [unwired: 11 in]
              n296 = call "myRIO_BRig_RT_dataLC_ENL1_Block_NS_l2.vi"() -> ("output_ENL1_Block_NS_l2"=w444:i32)  [unwired: 11 in]
              n297 = call "myRIO_BRig_RT_dataLC_ENL1_Count_NS_l2.vi"() -> ("output_ENL1_Count_NS_l2"=w445:i32)  [unwired: 11 in]
              n298 = call "myRIO_BRig_RT_dataLC_ENL1_Probability_NS_l2.vi"() -> ("output_ENL1_Probability_NS_l2"=w446:i32)  [unwired: 11 in]
              n299 = call "myRIO_BRig_RT_dataLC_Cue1_OnOff_Switch_l2.vi"() -> ("output_Cue1_OnOff_Switch_l2"=w437:i32)  [unwired: 11 in]
              n300 = call "myRIO_BRig_RT_dataLC_Cue1_Tdelay_Switch_l2.vi"() -> ("output_Cue1_Tdelay_Switch_l2"=w438:i32)  [unwired: 11 in]
              n301 = call "myRIO_BRig_RT_dataLC_Cue1_Block_Switch_l2.vi"() -> ("output_Cue1_Block_Switch_l2"=w439:i32)  [unwired: 11 in]
              n302 = call "myRIO_BRig_RT_dataLC_Cue1_Count_Switch_l2.vi"() -> ("output_Cue1_Count_Switch_l2"=w440:i32)  [unwired: 11 in]
              n303 = call "myRIO_BRig_RT_dataLC_Cue1_Probability_Switch_l2.vi"() -> ("output_Cue1_l2_First_Probability"=w441:i32)  [unwired: 11 in]
              n304 = call "myRIO_BRig_RT_dataLC_Cue1_OnOff_NS_l2.vi"() -> ("output_Cue1_OnOff_NS_l2"=w432:i32)  [unwired: 11 in]
              n305 = call "myRIO_BRig_RT_dataLC_Cue1_Tdelay_NS_l2.vi"() -> ("output_Cue1_Tdelay_NS_l2"=w433:i32)  [unwired: 11 in]
              n306 = call "myRIO_BRig_RT_dataLC_Cue1_Block_NS_l2.vi"() -> ("output_Cue1_Block_NS_l2"=w434:i32)  [unwired: 11 in]
              n307 = call "myRIO_BRig_RT_dataLC_Cue1_Count_NS_l2.vi"() -> ("output_Cue1_Count_NS_l2"=w435:i32)  [unwired: 11 in]
              n308 = call "myRIO_BRig_RT_dataLC_Cue1_Probability_NS_l2.vi"() -> ("output_Cue1_l2_All_Probability"=w436:i32)  [unwired: 11 in]
              n309 = call "myRIO_BRig_RT_dataLC_ENL1_delayOpt_Switch_l2.vi"() -> ("output_ENL1_delayOpt_Switch_l2"=w428:i32)  [unwired: 11 in]
              n310 = call "myRIO_BRig_RT_dataLC_ENL1_delayOpt_NS_l2.vi"() -> ("output_ENL1_delayOpt_NS_l2"=w429:i32)  [unwired: 11 in]
              n311 = call "myRIO_BRig_RT_dataLC_Cue1_delayOpt_Switch_l2.vi"() -> ("output_Cue1_delayOpt_Switch_l2"=w430:i32)  [unwired: 11 in]
              n312 = call "myRIO_BRig_RT_dataLC_Cue1_delayOpt_NS_l2.vi"() -> ("output_Cue1_delayOpt_NS_l2"=w431:i32)  [unwired: 11 in]
              n313 = Index Array(array=w481, index #1=w447, index #2=w448, index #3=w449, index #4=w450, index #5=w451, index #6=w442, index #7=w443, index #8=w444, index #9=w445, index #10=w446, index #11=w437, index #12=w438, index #13=w439, index #14=w440, index #15=w441, index #16=w432, index #17=w433, index #18=w434, index #19=w435, index #20=w436, index #21=w428, index #22=w429, index #23=w430, index #24=w431) -> (element #1=w479:u16, element #2=w478:u16, element #3=w477:u16, element #4=w476:u16, element #5=w475:u16, element #6=w474:u16, element #7=w473:u16, element #8=w472:u16, element #9=w471:u16, element #10=w470:u16, element #11=w469:u16, element #12=w468:u16, element #13=w467:u16, element #14=w466:u16, element #15=w465:u16, element #16=w464:u16, element #17=w463:u16, element #18=w462:u16, element #19=w461:u16, element #20=w460:u16, element #21=w455:u16, element #22=w454:u16, element #23=w453:u16, element #24=w452:u16)
              n314 = Not Equal To 0?(x=w479) -> (x != 0?=w483:bool)
              n315 = Not Equal To 0?(x=w474) -> (x != 0?=w482:bool)
              n316 = Not Equal To 0?(x=w469) -> (x != 0?=w485:bool)
              n317 = Not Equal To 0?(x=w464) -> (x != 0?=w484:bool)
              n318 = Not Equal To 0?(x=w455) -> (x != 0?=w457:bool)
              n319 = Not Equal To 0?(x=w454) -> (x != 0?=w458:bool)
              n320 = Not Equal To 0?(x=w453) -> (x != 0?=w459:bool)
              n321 = Not Equal To 0?(x=w452) -> (x != 0?=w456:bool)
              n322 = local write "LC_ENL1_OnOff_Switch_l2"(w483) -> ()
              n323 = local write "LC_ENL1_Tdelay_Switch_l2"(w478) -> ()
              n324 = local write "LC_ENL1_Block_Switch_l2"(w477) -> ()
              n325 = local write "LC_ENL1_Count_Switch_l2"(w476) -> ()
              n326 = local write "LC_ENL1_Probability_Switch_l2"(w475) -> ()
              n327 = local write "LC_ENL1_OnOff_NS_l2"(w482) -> ()
              n328 = local write "LC_ENL1_Tdelay_NS_l2"(w473) -> ()
              n329 = local write "LC_ENL1_Block_NS_l2"(w472) -> ()
              n330 = local write "LC_ENL1_Count_NS_l2"(w471) -> ()
              n331 = local write "LC_ENL1_Probability_NS_l2"(w470) -> ()
              n332 = local write "LC_Cue1_OnOff_Switch_l2"(w485) -> ()
              n333 = local write "LC_Cue1_Tdelay_Switch_l2"(w468) -> ()
              n334 = local write "LC_Cue1_Block_Switch_l2"(w467) -> ()
              n335 = local write "LC_Cue1_Count_Switch_l2"(w466) -> ()
              n336 = local write "LC_Cue1_Probability_Switch_l2"(w465) -> ()
              n337 = local write "LC_Cue1_OnOff_NS_l2"(w484) -> ()
              n338 = local write "LC_Cue1_Tdelay_NS_l2"(w463) -> ()
              n339 = local write "LC_Cue1_Block_NS_l2"(w462) -> ()
              n340 = local write "LC_Cue1_Count_NS_l2"(w461) -> ()
              n341 = local write "LC_Cue1_Probability_NS_l2"(w460) -> ()
              n342 = local write "LC_ENL1_delayOpt_Switch_l2"(w457) -> ()
              n343 = local write "LC_ENL1_delayOpt_NS_l2"(w458) -> ()
              n344 = local write "LC_Cue1_delayOpt_Switch_l2"(w459) -> ()
              n345 = local write "LC_Cue1_delayOpt_NS_l2"(w456) -> ()
            }
            frame "UploadSettings_dataLC_2" {
              # "Count"
              # "Tdelay"
              # "Prob"
              # "OnOff"
              # "Block"
              # "Selection NonSwitch"
              # "Count"
              # "Tdelay"
              # "Prob"
              # "OnOff"
              # "Block"
              # "Selection Switch"
              # "Trial"
              # "Tdelay"
              # "Prob"
              # "OnOff"
              # "Block"
              # "Wrong"
              # "Reward"
              # "Trial"
              # "Tdelay"
              # "Prob"
              # "OnOff"
              # "Block"
              n346 = call "myRIO_BRig_RT_dataLC_Reward_OnOff_l1.vi"() -> ("output_Reward_OnOff_l1"=w528:i32)  [unwired: 11 in]
              n347 = call "myRIO_BRig_RT_dataLC_Reward_Tdelay_l1.vi"() -> ("output_Reward_Tdelay_l1"=w527:i32)  [unwired: 11 in]
              n348 = call "myRIO_BRig_RT_dataLC_Reward_Block_l1.vi"() -> ("output_Reward_Block_l1"=w526:i32)  [unwired: 11 in]
              n349 = call "myRIO_BRig_RT_dataLC_Reward_Trial_l1.vi"() -> ("output_Reward_Trial_l1"=w525:i32)  [unwired: 11 in]
              n350 = call "myRIO_BRig_RT_dataLC_Reward_Probability_l1.vi"() -> ("output_Reward_Probability_l1"=w524:i32)  [unwired: 11 in]
              n351 = call "myRIO_BRig_RT_dataLC_Wrong_OnOff_l1.vi"() -> ("output_Wrong_OnOff_l1"=w517:i32)  [unwired: 11 in]
              n352 = call "myRIO_BRig_RT_dataLC_Wrong_Tdelay_l1.vi"() -> ("output_Wrong_Tdelay_l1"=w516:i32)  [unwired: 11 in]
              n353 = call "myRIO_BRig_RT_dataLC_Wrong_Block_l1.vi"() -> ("output_Wrong_Block_l1"=w515:i32)  [unwired: 11 in]
              n354 = call "myRIO_BRig_RT_dataLC_Wrong_Trial_l1.vi"() -> ("output_Wrong_Trial_l1"=w514:i32)  [unwired: 11 in]
              n355 = call "myRIO_BRig_RT_dataLC_Wrong_Probability_l1.vi"() -> ("output_Wrong_Probability_l1"=w513:i32)  [unwired: 11 in]
              n356 = call "myRIO_BRig_RT_dataLC_Selection_OnOff_Switch_l1.vi"() -> ("output_Selection_OnOff_Switch_l1"=w508:i32)  [unwired: 11 in]
              n357 = call "myRIO_BRig_RT_dataLC_Selection_Tdelay_Switch_l1.vi"() -> ("output_Selection_Tdelay_Switch_l1"=w507:i32)  [unwired: 11 in]
              n358 = call "myRIO_BRig_RT_dataLC_Selection_Block_Switch_l1.vi"() -> ("output_Selection_Block_Switch_l1"=w506:i32)  [unwired: 11 in]
              n359 = call "myRIO_BRig_RT_dataLC_Selection_Count_Switch_l1.vi"() -> ("output_Selection_Count_Switch_l1"=w505:i32)  [unwired: 11 in]
              n360 = call "myRIO_BRig_RT_dataLC_Selection_Probability_Switch_l1.vi"() -> ("output_Selection_Probability_Switch_l1"=w504:i32)  [unwired: 11 in]
              n361 = call "myRIO_BRig_RT_dataLC_Selection_OnOff_NS_l1.vi"() -> ("output_Selection_OnOff_NS_l1"=w503:i32)  [unwired: 11 in]
              n362 = call "myRIO_BRig_RT_dataLC_Selection_Tdelay_NS_l1.vi"() -> ("output_Selection_Tdelay_NS_l1"=w502:i32)  [unwired: 11 in]
              n363 = call "myRIO_BRig_RT_dataLC_Selection_Block_NS_l1.vi"() -> ("output_Selection_Block_NS_l1"=w501:i32)  [unwired: 11 in]
              n364 = call "myRIO_BRig_RT_dataLC_Selection_Count_NS_l1.vi"() -> ("output_Selection_Count_NS_l1"=w500:i32)  [unwired: 11 in]
              n365 = call "myRIO_BRig_RT_dataLC_Selection_Probability_NS_l1.vi"() -> ("output_Selection_Probability_NS_l1"=w499:i32)  [unwired: 11 in]
              n366 = Index Array(array=w529, index #1=w528, index #2=w527, index #3=w526, index #4=w525, index #5=w524, index #6=w517, index #7=w516, index #8=w515, index #9=w514, index #10=w513, index #11=w508, index #12=w507, index #13=w506, index #14=w505, index #15=w504, index #16=w503, index #17=w502, index #18=w501, index #19=w500, index #20=w499) -> (element #1=w523:u16, element #2=w522:u16, element #3=w521:u16, element #4=w520:u16, element #5=w519:u16, element #6=w518:u16, element #7=w512:u16, element #8=w511:u16, element #9=w510:u16, element #10=w509:u16, element #11=w496:u16, element #12=w495:u16, element #13=w494:u16, element #14=w493:u16, element #15=w492:u16, element #16=w491:u16, element #17=w490:u16, element #18=w489:u16, element #19=w488:u16, element #20=w487:u16)
              n367 = Not Equal To 0?(x=w523) -> (x != 0?=w531:bool)
              n368 = Not Equal To 0?(x=w518) -> (x != 0?=w530:bool)
              n369 = Not Equal To 0?(x=w496) -> (x != 0?=w498:bool)
              n370 = Not Equal To 0?(x=w491) -> (x != 0?=w497:bool)
              n371 = local write "LC_Reward_OnOff_l1"(w531) -> ()
              n372 = local write "LC_Reward_Tdelay_l1"(w522) -> ()
              n373 = local write "LC_Reward_Block_l1"(w521) -> ()
              n374 = local write "LC_Reward_Trial_l1"(w520) -> ()
              n375 = local write "LC_Reward_Probability_l1"(w519) -> ()
              n376 = local write "LC_Wrong_OnOff_l1"(w530) -> ()
              n377 = local write "LC_Wrong_Tdelay_l1"(w512) -> ()
              n378 = local write "LC_Wrong_Block_l1"(w511) -> ()
              n379 = local write "LC_Wrong_Trial_l1"(w510) -> ()
              n380 = local write "LC_Wrong_Probability_l1"(w509) -> ()
              n381 = local write "LC_Sel_OnOff_Switch_l1"(w498) -> ()
              n382 = local write "LC_Sel_Tdelay_Switch_l1"(w495) -> ()
              n383 = local write "LC_Sel_Block_Switch_l1"(w494) -> ()
              n384 = local write "LC_Sel_Count_Switch_l1"(w493) -> ()
              n385 = local write "LC_Sel_Probability_Switch_l1"(w492) -> ()
              n386 = local write "LC_Sel_OnOff_NS_l1"(w497) -> ()
              n387 = local write "LC_Sel_Tdelay_NS_l1"(w490) -> ()
              n388 = local write "LC_Sel_Block_NS_l1"(w489) -> ()
              n389 = local write "LC_Sel_Count_NS_l1"(w488) -> ()
              n390 = local write "LC_Sel_Probability_NS_l1"(w487) -> ()
            }
            frame "UploadSettings_dataLC_4" {
              # "Count"
              # "Tdelay"
              # "Prob"
              # "OnOff"
              # "Block"
              # "Selection NonSwitch"
              # "Count"
              # "Tdelay"
              # "Prob"
              # "OnOff"
              # "Block"
              # "Selection Switch"
              # "Trial"
              # "Tdelay"
              # "Prob"
              # "OnOff"
              # "Block"
              # "Wrong"
              # "Reward"
              # "Trial"
              # "Tdelay"
              # "Prob"
              # "OnOff"
              # "Block"
              n391 = call "myRIO_BRig_RT_dataLC_Reward_OnOff_l2.vi"() -> ("output_Reward_OnOff_l2"=w539:i32)  [unwired: 11 in]
              n392 = call "myRIO_BRig_RT_dataLC_Reward_Tdelay_l2.vi"() -> ("output_Reward_Tdelay_l2"=w540:i32)  [unwired: 11 in]
              n393 = call "myRIO_BRig_RT_dataLC_Reward_Block_l2.vi"() -> ("output_Reward_Block_l2"=w541:i32)  [unwired: 11 in]
              n394 = call "myRIO_BRig_RT_dataLC_Reward_Trial_l2.vi"() -> ("output_Reward_Trial_l2"=w542:i32)  [unwired: 11 in]
              n395 = call "myRIO_BRig_RT_dataLC_Reward_Probability_l2.vi"() -> ("output_Reward_Probability_l2"=w543:i32)  [unwired: 11 in]
              n396 = call "myRIO_BRig_RT_dataLC_Wrong_OnOff_l2.vi"() -> ("output_Wrong_OnOff_l2"=w534:i32)  [unwired: 11 in]
              n397 = call "myRIO_BRig_RT_dataLC_Wrong_Tdelay_l2.vi"() -> ("output_Wrong_Tdelay_l2"=w535:i32)  [unwired: 11 in]
              n398 = call "myRIO_BRig_RT_dataLC_Wrong_Block_l2.vi"() -> ("output_Wrong_Block_l2"=w536:i32)  [unwired: 11 in]
              n399 = call "myRIO_BRig_RT_dataLC_Wrong_Trial_l2.vi"() -> ("output_Wrong_Trial_l2"=w537:i32)  [unwired: 11 in]
              n400 = call "myRIO_BRig_RT_dataLC_Wrong_Probability_l2.vi"() -> ("output_Wrong_Probability_l2"=w538:i32)  [unwired: 11 in]
              n401 = call "myRIO_BRig_RT_dataLC_Selection_OnOff_Switch_l2.vi"() -> ("output_Selection_OnOff_Switch_l2"=w549:i32)  [unwired: 11 in]
              n402 = call "myRIO_BRig_RT_dataLC_Selection_Tdelay_Switch_l2.vi"() -> ("output_Selection_Tdelay_Switch_l2"=w550:i32)  [unwired: 11 in]
              n403 = call "myRIO_BRig_RT_dataLC_Selection_Block_Switch_l2.vi"() -> ("output_Selection_Block_Switch_l2"=w551:i32)  [unwired: 11 in]
              n404 = call "myRIO_BRig_RT_dataLC_Selection_Count_Switch_l2.vi"() -> ("output_Selection_Count_Switch_l2"=w552:i32)  [unwired: 11 in]
              n405 = call "myRIO_BRig_RT_dataLC_Selection_Probability_Switch_l2.vi"() -> ("output_Selection_Probability_Switch_l1"=w553:i32)  [unwired: 11 in]
              n406 = call "myRIO_BRig_RT_dataLC_Selection_OnOff_NS_l2.vi"() -> ("output_Selection_OnOff_NS_l2"=w544:i32)  [unwired: 11 in]
              n407 = call "myRIO_BRig_RT_dataLC_Selection_Tdelay_NS_l2.vi"() -> ("output_Selection_Tdelay_NS_l2"=w545:i32)  [unwired: 11 in]
              n408 = call "myRIO_BRig_RT_dataLC_Selection_Block_NS_l2.vi"() -> ("output_Selection_Block_NS_l2"=w546:i32)  [unwired: 11 in]
              n409 = call "myRIO_BRig_RT_dataLC_Selection_Count_NS_l2.vi"() -> ("output_Selection_Count_NS_l2"=w547:i32)  [unwired: 11 in]
              n410 = call "myRIO_BRig_RT_dataLC_Selection_Probability_NS_l2.vi"() -> ("output_Selection_Probability_NS_l2"=w548:i32)  [unwired: 11 in]
              n411 = Index Array(array=w576, index #1=w539, index #2=w540, index #3=w541, index #4=w542, index #5=w543, index #6=w534, index #7=w535, index #8=w536, index #9=w537, index #10=w538, index #11=w549, index #12=w550, index #13=w551, index #14=w552, index #15=w553, index #16=w544, index #17=w545, index #18=w546, index #19=w547, index #20=w548) -> (element #1=w575:u16, element #2=w574:u16, element #3=w573:u16, element #4=w572:u16, element #5=w571:u16, element #6=w570:u16, element #7=w569:u16, element #8=w568:u16, element #9=w567:u16, element #10=w566:u16, element #11=w563:u16, element #12=w562:u16, element #13=w561:u16, element #14=w560:u16, element #15=w559:u16, element #16=w558:u16, element #17=w557:u16, element #18=w556:u16, element #19=w555:u16, element #20=w554:u16)
              n412 = Not Equal To 0?(x=w575) -> (x != 0?=w578:bool)
              n413 = Not Equal To 0?(x=w570) -> (x != 0?=w577:bool)
              n414 = Not Equal To 0?(x=w563) -> (x != 0?=w565:bool)
              n415 = Not Equal To 0?(x=w558) -> (x != 0?=w564:bool)
              n416 = local write "LC_Reward_OnOff_l2"(w578) -> ()
              n417 = local write "LC_Reward_Tdelay_l2"(w574) -> ()
              n418 = local write "LC_Reward_Block_l2"(w573) -> ()
              n419 = local write "LC_Reward_Trial_l2"(w572) -> ()
              n420 = local write "LC_Reward_Probability_l2"(w571) -> ()
              n421 = local write "LC_Wrong_OnOff_l2"(w577) -> ()
              n422 = local write "LC_Wrong_Tdelay_l2"(w569) -> ()
              n423 = local write "LC_Wrong_Block_l2"(w568) -> ()
              n424 = local write "LC_Wrong_Trial_l2"(w567) -> ()
              n425 = local write "LC_Wrong_Probability_l2"(w566) -> ()
              n426 = local write "LC_Sel_OnOff_Switch_l2"(w565) -> ()
              n427 = local write "LC_Sel_Tdelay_Switch_l2"(w562) -> ()
              n428 = local write "LC_Sel_Block_Switch_l2"(w561) -> ()
              n429 = local write "LC_Sel_Count_Switch_l2"(w560) -> ()
              n430 = local write "LC_Sel_Probability_Switch_l2"(w559) -> ()
              n431 = local write "LC_Sel_OnOff_NS_l2"(w564) -> ()
              n432 = local write "LC_Sel_Tdelay_NS_l2"(w557) -> ()
              n433 = local write "LC_Sel_Block_NS_l2"(w556) -> ()
              n434 = local write "LC_Sel_Count_NS_l2"(w555) -> ()
              n435 = local write "LC_Sel_Probability_NS_l2"(w554) -> ()
            }
            frame "UploadSettings_dataMTrig_1" {
              # "Tdelay_R"
              # "Tdelay_L"
              # "Tcycle_R"
              # "Tcycle_L"
              # "RewCalib_nCycle_R"
              # "RewCalib_nCycle_L"
              # "Solenoid"
              # "Laser_Tcycle"
              n436 = call "myRIO_BRig_RT_dataMTrig_Laser_Tcycle.vi"() -> ("output_Laser_Tcycle"=w588:i32)  [unwired: 11 in]
              n437 = call "myRIO_BRig_RT_dataMTrig_Solenoid_RewCalib_nCycle__L.vi"() -> ("output_Solenoid_RewCalib_nCycle__L"=w587:i32)  [unwired: 11 in]
              n438 = call "myRIO_BRig_RT_dataMTrig_Solenoid_RewCalib_nCycle__R.vi"() -> ("output_Solenoid_RewCalib_nCycle__R"=w586:i32)  [unwired: 11 in]
              n439 = call "myRIO_BRig_RT_dataMTrig_Solenoid_Tdelay__L.vi"() -> ("output_Solenoid_Tdelay__L"=w583:i32)  [unwired: 11 in]
              n440 = call "myRIO_BRig_RT_dataMTrig_Solenoid_Tdelay__R.vi"() -> ("output_Solenoid_Tdelay__R"=w582:i32)  [unwired: 11 in]
              n441 = call "myRIO_BRig_RT_dataMTrig_Solenoid_Tcycle__L.vi"() -> ("output_Solenoid_Tcycle__L"=w585:i32)  [unwired: 11 in]
              n442 = call "myRIO_BRig_RT_dataMTrig_Solenoid_Tcycle__R.vi"() -> ("output_Solenoid_Tcycle__R"=w584:i32)  [unwired: 11 in]
              n443 = Index Array(array=w581, index #1=w588, index #2=w587, index #3=w586, index #4=w585, index #5=w584, index #6=w583, index #7=w582) -> (element #1=w595:u16, element #2=w594:u16, element #3=w593:u16, element #4=w592:u16, element #5=w591:u16, element #6=w590:u16, element #7=w589:u16)
              n444 = Replace Array Subset(array=w597, new element #1=w595, index #1=w588, new element #2=w594, index #2=w587, new element #3=w593, index #3=w586, new element #4=w592, index #4=w585, new element #5=w591, index #5=w584, new element #6=w590, index #6=w583, new element #7=w589, index #7=w582) -> (w596:u16[])
              n445 = local write "MTrig_Solenoid_Tcycle__L"(w592) -> ()
              n446 = local write "MTrig_Solenoid_Tcycle__R"(w591) -> ()
              n447 = local write "MTrig_Laser_Tcycle"(w595) -> ()
            }
            frame "Idle" {
              # "There are a number of tasks we need to perform\nwhile idling. To preserve our timing loop, we\nbreak up the IDLE state into smaller states"
              # "Laser_Tcycle"
              # "Audio_Tcycle_R"
              # "Audio_Tcycle_L"
              n448 = local read "Laser_power_min_l1"() -> (w606:dbl)
              n449 = local read "Laser_power_min_l2"() -> (w605:dbl)
              n450 = local read "Audio_Amp__R"() -> (w608:u16)
              n451 = local read "Audio_Amp__L"() -> (w610:u16)
              n452 = local read "Audio_Freq__R"() -> (w607:u8)
              n453 = local read "Audio_Freq__L"() -> (w609:u8)
              n454 = local read "CueLed_baseline"() -> (w601:bool)
              n455 = Select(t=myRIO_BRig_RT__Case_NonExp_stateList."SendData" ("Enum"), s="SendData", f=myRIO_BRig_RT__Case_NonExp_stateList."Idle_2" ("Enum")) -> (s? t:f=w615:T1)
              n456 = call "myRIO__convert__Voltage_to_FPGAvalue.vi"("input_voltage"=w606) -> ("output_PortC"=w599:i16)  [unwired: 9 in, 1 out]
              n457 = call "myRIO__convert__Voltage_to_FPGAvalue.vi"("input_voltage"=w605) -> ("output_PortC"=w600:i16)  [unwired: 9 in, 1 out]
              n458 = Select(t=myRIO_BRig_RT__Case_NonExp_stateList."TestConnection" ("Enum"), s="TestConnection", f=w615) -> (s? t:f=w619:T1)
              n459 = xnode "Read/Write Control"("FPGA VI Reference In"=w612, "error in"=w611, "audioAmp_L"=w610, "audioFreq_L_kHz"=w609, "audioAmp_R"=w608, "audioFreq_R_kHz"=w607, "AnaOut_0"=w599, "AnaOut_1"=w600, "CueLed_Baseline"=w601) -> ("error out"=w604:errorcluster)  [unwired: 1 out]
              n460 = call "myRIO_BRig_RT_dataMTrig_Audio_Tcycle__L.vi"() -> ("output_Audio_Tcycle__L"=w626:i32)  [unwired: 11 in]
              n461 = call "myRIO_BRig_RT_dataMTrig_Audio_Tcycle__R.vi"() -> ("output_Audio_Tcycle__R"=w625:i32)  [unwired: 11 in]
              n462 = call "myRIO_BRig_RT_dataMTrig_Laser_Tcycle.vi"() -> ("output_Laser_Tcycle"=w624:i32)  [unwired: 11 in]
              n463 = call "myRIO_BRig_RT_dataMTrig_CueLed_Tcycle.vi"() -> ("output_CueLed_Tcycle"=w603:i32)  [unwired: 11 in]
              n464 = local write "error out"(w604) -> ()
              n465 = local read "Tcycle_Cue_Audio_min"() -> (w614:u16)
              n466 = local read "MTrig_Laser_Tcycle"() -> (w613:u16)
              n467 = local read "Tcycle_Cue_LED_min"() -> (w602:u16)
              n468 = Replace Array Subset(array=w622, new element #1=w614, index #1=w626, new element #2=w614, index #2=w625, new element #3=w613, index #3=w624, new element #4=w602, index #4=w603) -> (w623:u16[])
            }
            frame "Idle_2" {
              w649 = u16 0 ("t")
              # "There are a number of tasks we need to perform\nwhile idling. To preserve our timing loop, we\nbreak up the IDLE state into smaller states"
              # "Ncycles"
              # "Ncycles"
              # "RewCalib"
              # "RewCalib"
              # "Solenoid R"
              # "Solenoid L"
              n469 = local read "MTrig_Laser_Switch"() -> (w642:bool)
              n470 = local read "count_warmup_R"() -> (w648:u16)
              n471 = local read "count_warmup_L"() -> (w653:u16)
              n472 = call "myRIO_BRig_RT_dataMTrig_Solenoid_RewCalib_OnOff__R.vi"() -> ("output_Solenoid_RewCalib_OnOff__R"=w664:i32)  [unwired: 11 in]
              n473 = call "myRIO_BRig_RT_dataMTrig_Solenoid_N__R.vi"() -> ("output_Solenoid_N__R"=w663:i32)  [unwired: 11 in]
              n474 = call "myRIO_BRig_RT_dataMTrig_Solenoid_RewCalib_OnOff__L.vi"() -> ("output_Solenoid_RewCalib_OnOff__L"=w679:i32)  [unwired: 11 in]
              n475 = call "myRIO_BRig_RT_dataMTrig_Solenoid_N__L.vi"() -> ("output_Solenoid_N__L"=w667:i32)  [unwired: 11 in]
              n476 = case shown="False" w642 {
                tunnel: "LR_reward_Event" -> [w685 w689]
                tunnel: "LR_wrong_Event" -> [w684 w688]
                tunnel: "LR_reward_Laser" -> [w683 w687]
                tunnel: "LR_wrong_Laser" -> [w682 w686]
                tunnel: [w685 _] -> w637
                tunnel: [w684 _] -> w636
                tunnel: [w683 _] -> w635
                tunnel: [w682 _] -> w634
                tunnel: [_ w689] -> w633
                tunnel: [_ w688] -> w632
                tunnel: [_ w687] -> w631
                tunnel: [_ w686] -> w630
                frame False {
                }
                frame True {
                }
              }
              n477 = Index Array(array=w670, index #1=w679, index #2=w667, index #3=w664, index #4=w663) -> (element #1=w666:u16, element #2=w661:u16, element #3=w662:u16, element #4=w660:u16)
              n478 = Select(t=w649, s="count_warmup_L_reset", f=w653) -> (s? t:f=→"count_warmup_L":u16)
              n479 = Select(t=w649, s="count_warmup_R_reset", f=w648) -> (s? t:f=→"count_warmup_R":u16)
              n480 = local read "RewCalib_Trig_L"() -> (w659:bool)
              n481 = local read "RewCalib_Trig_R"() -> (w658:bool)
              n482 = Equal To 0?(x=w661) -> (x = 0?=w669:bool)
              n483 = Equal To 0?(x=w660) -> (x = 0?=w668:bool)
              n484 = Not Equal To 0?(x=w662) -> (x != 0?=w680:bool)
              n485 = Not Equal To 0?(x=w666) -> (x != 0?=w681:bool)
              n486 = And(x=w669, y=w668) -> (x .and. y?=w673:bool)
              n487 = Or(x=w659, y=w658) -> (x .or. y?=w674:bool)
              n488 = Not Exclusive Or(1:w681, 2:w659) -> (0:w676:bool)
              n489 = xnode "Read/Write Control"("FPGA VI Reference In"=w628, "error in"=w629, "Left(F)_or_Right(T)"="Left(F)_or_Right(T)", "SelectionState"="SelectionState", "ignoreWrong"="ignoreWrong", "LR_reward_Event_l1"=w637, "LR_wrong_Event_l1"=w636, "LR_reward_Laser_l1"=w635, "LR_wrong_Laser_l1"=w634, "LR_reward_Event_l2"=w633, "LR_wrong_Event_l2"=w632, "LR_reward_Laser_l2"=w631, "LR_wrong_laser_l2"=w630) -> ("error out"=w627:errorcluster, "SelectReward"=→"SelectReward":bool, "SelectWrong"=→"SelectWrong":bool)  [unwired: 1 out]
              n490 = Not Exclusive Or(1:w680, 2:w658) -> (0:w678:bool)
              n491 = And(x=w674, y=w673) -> (x .and. y?=w656:bool)
              n492 = Not(x=w676) -> (.not. x?=w675:bool)
              n493 = Not(x=w678) -> (.not. x?=w677:bool)
              n494 = Or(x=w675, y=w677) -> (x .or. y?=w657:bool)
              n495 = Or(x=w656, y=w657) -> (x .or. y?=w672:bool)
              n496 = local write "error out"(w627) -> ()
              n497 = Select(t=myRIO_BRig_RT__Case_NonExp_stateList."RewardCalibration_pre" ("Enum"), s=w672, f=myRIO_BRig_RT__Case_NonExp_stateList."Idle_3" ("Enum")) -> (s? t:f=w655:T1)
            }
            frame "Idle_3" {
              # "There are a number of tasks we need to perform\nwhile idling. To preserve our timing loop, we\nbreak up the IDLE state into smaller states"
              n498 = local read "Laser_Tshutter_l1"() -> (w708:dbl)
              n499 = local read "Laser_duration_l1"() -> (w707:u16)
              n500 = local read "Laser_Tshutter_l2"() -> (w704:dbl)
              n501 = local read "Laser_duration_l2"() -> (w703:u16)
              n502 = local read "Laser_Tpeak_l1"() -> (w710:dbl)
              n503 = local read "Laser_Tpeak_l2"() -> (w706:dbl)
              n504 = local read "CueLed_Tpeak"() -> (w701:dbl)
              n505 = local read "Laser_Freq_l1"() -> (w709:dbl)
              n506 = local read "Laser_Freq_l2"() -> (w705:dbl)
              n507 = local read "CueLed_Freq"() -> (w700:dbl)
              n508 = local read "FPGA_count2ms"() -> (w702:dbl)
              n509 = To Unsigned Word Integer(number=w702) -> (unsigned 16bit integer=w711:u16)
              n510 = call "myRIO_BRig_RT__calc_laser_FPGA_N.vi"("input_FPGA_ms2count"=w702, "input_Tpeak"=w710, "input_Freq"=w709, "input_Tshutter"=w708, "input_duration"=w707) -> ("output_laser_Npeak"=w699:u32, "output_laser_Nvalley"=w697:u32, "output_laser_Nshutter"=w695:u32, "output_laser_Nduration"=w693:u32)  [unwired: 6 in, 1 out]
              n511 = call "myRIO_BRig_RT__calc_laser_FPGA_N.vi"("input_FPGA_ms2count"=w702, "input_Tpeak"=w706, "input_Freq"=w705, "input_Tshutter"=w704, "input_duration"=w703) -> ("output_laser_Npeak"=w698:u32, "output_laser_Nvalley"=w696:u32, "output_laser_Nshutter"=w694:u32, "output_laser_Nduration"=w692:u32)  [unwired: 6 in, 1 out]
              n512 = call "myRIO_BRig_RT__calc_laser_FPGA_N__CueLed.vi"("input_FPGA_ms2count"=w702, "input_Tpeak"=w701, "input_Freq"=w700) -> ("output_laser_Npeak"=w691:u32, "output_laser_Nvalley"=w690:u32)  [unwired: 11 in]
              n513 = xnode "Read/Write Control"("FPGA VI Reference In"=w716, "error in"=w715, "k1__counter_per_ms"=w711, "LC_nPeak_l1"=w699, "LC_nPeak_l2"=w698, "LC_nValley_l1"=w697, "LC_nValley_l2"=w696, "LC_nShutter_l1"=w695, "LC_nShutter_l2"=w694, "LR_reward_nTotal_l1"=w693, "LR_wrong_nTotal_l1"=w693, "LR_reward_nTotal_l2"=w692, "LR_wrong_nTotal_l2"=w692, "CueLed_nPeak"=w691, "CueLed_nValley"=w690) -> ("error out"=w712:errorcluster)  [unwired: 1 out]
              n514 = local write "error out"(w712) -> ()
            }
            frame "Idle_4" {
              w738 = u8 0 ("f")
              # "There are a number of tasks we need to perform\nwhile idling. To preserve our timing loop, we\nbreak up the IDLE state into smaller states"
              n515 = local read "MTrig_Solenoid_trig__L"() -> (w729:bool)
              n516 = local read "MTrig_Solenoid_trig__R"() -> (w739:bool)
              n517 = local read "warmupType"() -> (w722:u8)
              n518 = local read "warmup"() -> (w731:bool)
              n519 = Not Equal To 0?(x=w722) -> (x != 0?=w721:bool)
              n520 = Not(x=w721) -> (.not. x?=w732:bool)
              n521 = Select(t=u8 1, s=w729, f=w738) -> (s? t:f=w737:u8)
              n522 = Select(t=u8 2, s=w739, f=w738) -> (s? t:f=w736:u8)
              n523 = And(x=w731, y=w732) -> (x .and. y?=w730:bool)
              n524 = And(x=w731, y=w721) -> (x .and. y?=w725:bool)
              n525 = Add(x=w737, y=w736) -> (x+y=w735:u8)
              n526 = case shown="3" w735 {
                tunnel: w734 -> [w742 w746 w779 w810]
                tunnel: [w742 w745 w778 w809] -> w733
                tunnel: w730 -> [_ w744 w777 w808]
                tunnel: [_ TRUE TRUE TRUE] -> w727
                frame 0, Default {
                }
                frame 1 {
                  n527 = case shown="False" w744 {
                    tunnel: w746 -> [w759 w774]
                    tunnel: [w758 w773] -> w745
                    frame True {
                      # "Audio_L"
                      # "Solenoid_L"
                      n528 = call "myRIO_BRig_RT_dataMTrig_Solenoid_N__L.vi"() -> ("output_Solenoid_N__L"=w756:i32)  [unwired: 11 in]
                      n529 = call "myRIO_BRig_RT_dataMTrig_Audio_N__L.vi"() -> ("output_Audio_N__L"=w754:i32)  [unwired: 11 in]
                      n530 = call "myRIO_BRig_RT_dataMTrig_Audio_N__R.vi"() -> ("output_Audio_N__R"=w749:i32)  [unwired: 11 in]
                      n531 = local read "sp_LeftSpout"() -> (w753:u16)
                      n532 = Index Array(array=w759, index #1=w756, index #2=w754, index #3=w749) -> (element #1=w757:u16, element #2=w752:u16, element #3=w751:u16)
                      n533 = Increment(x=w757) -> (x+1=w755:u16)
                      n534 = case shown="2" w753 {
                        tunnel: w752 -> [w762 w765 w767]
                        tunnel: w751 -> [w760 w764 w769]
                        tunnel: [w761 w765 w766] -> w750
                        tunnel: [w760 w763 w768] -> w748
                        frame 0, Default {
                          n535 = Increment(x=w762) -> (x+1=w761:u16)
                        }
                        frame 1 {
                          n536 = Increment(x=w764) -> (x+1=w763:u16)
                        }
                        frame 2 {
                          n537 = Increment(x=w769) -> (x+1=w768:u16)
                          n538 = Increment(x=w767) -> (x+1=w766:u16)
                        }
                      }
                      n539 = Replace Array Subset(array=w759, new element #1=w755, index #1=w756, new element #2=w750, index #2=w754, new element #3=w748, index #3=w749) -> (w758:u16[])
                    }
                    frame False {
                      # "Solenoid_L"
                      n540 = call "myRIO_BRig_RT_dataMTrig_Solenoid_N__L.vi"() -> ("output_Solenoid_N__L"=w771:i32)  [unwired: 11 in]
                      n541 = Index Array(array=w774, index=w771) -> (element=w772:u16)
                      n542 = Increment(x=w772) -> (x+1=w770:u16)
                      n543 = Replace Array Subset(array=w774, new element=w770, index=w771) -> (w773:u16[])
                    }
                  }
                  n544 = local write "MTrig_Solenoid_trig__L"(FALSE) -> ()
                }
                frame 2 {
                  n545 = case shown="True" w777 {
                    tunnel: w779 -> [w791 w806]
                    tunnel: [w790 w805] -> w778
                    frame True {
                      # "Solenoid_R"
                      n546 = call "myRIO_BRig_RT_dataMTrig_Solenoid_N__R.vi"() -> ("output_Solenoid_N__R"=w780:i32)  [unwired: 11 in]
                      n547 = call "myRIO_BRig_RT_dataMTrig_Audio_N__L.vi"() -> ("output_Audio_N__L"=w787:i32)  [unwired: 11 in]
                      n548 = call "myRIO_BRig_RT_dataMTrig_Audio_N__R.vi"() -> ("output_Audio_N__R"=w782:i32)  [unwired: 11 in]
                      n549 = local read "sp_RightSpout"() -> (w786:u16)
                      n550 = Index Array(array=w791, index #1=w780, index #2=w787, index #3=w782) -> (element #1=w789:u16, element #2=w785:u16, element #3=w784:u16)
                      n551 = Increment(x=w789) -> (x+1=w788:u16)
                      n552 = case shown="2" w786 {
                        tunnel: w785 -> [w794 w797 w799]
                        tunnel: w784 -> [w792 w796 w801]
                        tunnel: [w793 w797 w798] -> w783
                        tunnel: [w792 w795 w800] -> w781
                        frame 0, Default {
                          n553 = Increment(x=w794) -> (x+1=w793:u16)
                        }
                        frame 1 {
                          n554 = Increment(x=w796) -> (x+1=w795:u16)
                        }
                        frame 2 {
                          n555 = Increment(x=w801) -> (x+1=w800:u16)
                          n556 = Increment(x=w799) -> (x+1=w798:u16)
                        }
                      }
                      n557 = Replace Array Subset(array=w791, new element #1=w788, index #1=w780, new element #2=w783, index #2=w787, new element #3=w781, index #3=w782) -> (w790:u16[])
                    }
                    frame False {
                      # "Solenoid_R"
                      n558 = call "myRIO_BRig_RT_dataMTrig_Solenoid_N__R.vi"() -> ("output_Solenoid_N__R"=w802:i32)  [unwired: 11 in]
                      n559 = Index Array(array=w806, index=w802) -> (element=w804:u16)
                      n560 = Increment(x=w804) -> (x+1=w803:u16)
                      n561 = Replace Array Subset(array=w806, new element=w803, index=w802) -> (w805:u16[])
                    }
                  }
                  n562 = local write "MTrig_Solenoid_trig__R"(FALSE) -> ()
                }
                frame 3 {
                  w811 = FALSE
                  n563 = case shown="True" w808 {
                    tunnel: w810 -> [w825 w833]
                    tunnel: [w824 w832] -> w809
                    frame True {
                      # "Audio_R"
                      # "Solenoid_R"
                      # "Audio_L"
                      # "Solenoid_L"
                      n564 = call "myRIO_BRig_RT_dataMTrig_Solenoid_N__L.vi"() -> ("output_Solenoid_N__L"=w819:i32)  [unwired: 11 in]
                      n565 = call "myRIO_BRig_RT_dataMTrig_Audio_N__L.vi"() -> ("output_Audio_N__L"=w817:i32)  [unwired: 11 in]
                      n566 = call "myRIO_BRig_RT_dataMTrig_Solenoid_N__R.vi"() -> ("output_Solenoid_N__R"=w815:i32)  [unwired: 11 in]
                      n567 = call "myRIO_BRig_RT_dataMTrig_Audio_N__R.vi"() -> ("output_Audio_N__R"=w814:i32)  [unwired: 11 in]
                      n568 = Index Array(array=w825, index #1=w819, index #2=w817, index #3=w815, index #4=w814) -> (element #1=w823:u16, element #2=w822:u16, element #3=w821:u16, element #4=w820:u16)
                      n569 = Increment(x=w820) -> (x+1=w812:u16)
                      n570 = Increment(x=w823) -> (x+1=w818:u16)
                      n571 = Increment(x=w822) -> (x+1=w816:u16)
                      n572 = Increment(x=w821) -> (x+1=w813:u16)
                      n573 = Replace Array Subset(array=w825, new element #1=w818, index #1=w819, new element #2=w816, index #2=w817, new element #3=w813, index #3=w815, new element #4=w812, index #4=w814) -> (w824:u16[])
                    }
                    frame False {
                      # "Solenoid_R"
                      # "Solenoid_L"
                      n574 = call "myRIO_BRig_RT_dataMTrig_Solenoid_N__L.vi"() -> ("output_Solenoid_N__L"=w829:i32)  [unwired: 11 in]
                      n575 = call "myRIO_BRig_RT_dataMTrig_Solenoid_N__R.vi"() -> ("output_Solenoid_N__R"=w826:i32)  [unwired: 11 in]
                      n576 = Index Array(array=w833, index #1=w829, index #2=w826) -> (element #1=w831:u16, element #2=w830:u16)
                      n577 = Increment(x=w831) -> (x+1=w828:u16)
                      n578 = Increment(x=w830) -> (x+1=w827:u16)
                      n579 = Replace Array Subset(array=w833, new element #1=w828, index #1=w829, new element #2=w827, index #2=w826) -> (w832:u16[])
                    }
                  }
                  n580 = local write "MTrig_Solenoid_trig__L"(w811) -> ()
                  n581 = local write "MTrig_Solenoid_trig__R"(w811) -> ()
                }
              }
              n582 = local read "get_countPerMS"() -> (w720:bool)
              n583 = Select(t=myRIO_BRig_RT__Case_NonExp_stateList."Get_FPGA_count_per_ms" ("Enum"), s=w720, f=myRIO_BRig_RT__Case_NonExp_stateList."Idle_6" ("Enum")) -> (s? t:f=w718:T1)
              n584 = Select(t=myRIO_BRig_RT__Case_NonExp_stateList."Cue_pre", s=w725, f=myRIO_BRig_RT__Case_NonExp_stateList."DispenseWater_pre" ("Enum")) -> (s? t:f=w723:T1)
              n585 = Select(t=w723, s=w727, f=w718) -> (s? t:f=w728:T1)
            }
            frame "Idle_5" {
              w856 = u8 0 ("f")
              # "There are a number of tasks we need to perform\nwhile idling. To preserve our timing loop, we\nbreak up the IDLE state into smaller states"
              n586 = local read "MTrig_Solenoid_trig__L"() -> (w848:bool)
              n587 = local read "MTrig_Solenoid_trig__R"() -> (w857:bool)
              n588 = local read "warmup"() -> (w835:bool)
              n589 = local read "warmupType"() -> (w837:u8)
              n590 = local read "Cue1Param_CueType_Switch"() -> (w836:u16)
              n591 = Not Equal To 0?(x=w837) -> (x != 0?=w834:bool)
              n592 = Not(x=w834) -> (.not. x?=w850:bool)
              n593 = And(x=w834, y=w835) -> (x .and. y?=w844:bool)
              n594 = Select(t=u8 1, s=w848, f=w856) -> (s? t:f=w855:u8)
              n595 = Select(t=u8 2, s=w857, f=w856) -> (s? t:f=w854:u8)
              n596 = And(x=w835, y=w850) -> (x .and. y?=w849:bool)
              n597 = Add(x=w855, y=w854) -> (x+y=w853:u8)
              n598 = case shown="1" w853 {
                tunnel: w852 -> [w860 w865 w902 w939]
                tunnel: [w860 w864 w903 w940] -> w851
                tunnel: w849 -> [_ w863 w901 w942]
                tunnel: [_ TRUE TRUE TRUE] -> w846
                tunnel: w836 -> [_ w861 w900 w941]
                frame 0, Default {
                }
                frame 1 {
                  n599 = case shown="True" w863 {
                    tunnel: w865 -> [w887 w899]
                    tunnel: [w888 w898] -> w864
                    tunnel: w861 -> [w867 _]
                    frame True {
                      n600 = case shown="2" w867 {
                        tunnel: [TRUE _ w892 w894] -> w876
                        tunnel: [_ TRUE w891 w894] -> w883
                        frame 0, Default {
                          # "Audio"
                        }
                        frame 1 {
                          # "LED"
                        }
                        frame 2 {
                          # "Audio or LED"
                          n601 = local read "Cue1Param_AudioLed_Probability_Switch"() -> (w893:u16)
                          n602 = call "myRIO__convert__Probability_to_TrueFalse.vi"("input_probability_u16"=w893) -> ("output_TF"=w891:bool)  [unwired: 10 in]
                          n603 = Not(x=w891) -> (.not. x?=w892:bool)
                        }
                        frame 3 {
                          w894 = TRUE
                          # "Audio and LED"
                        }
                      }
                      n604 = local read "sp_LeftSpout"() -> (w879:u16)
                      n605 = call "myRIO_BRig_RT_dataMTrig_Solenoid_N__L.vi"() -> ("output_Solenoid_N__L"=w886:i32)  [unwired: 11 in]
                      n606 = call "myRIO_BRig_RT_dataMTrig_CueLed_N.vi"() -> ("output_CueLed_N"=w884:i32)  [unwired: 11 in]
                      n607 = call "myRIO_BRig_RT_dataMTrig_Audio_N__L.vi"() -> ("output_Audio_N__L"=w871:i32)  [unwired: 11 in]
                      n608 = call "myRIO_BRig_RT_dataMTrig_Audio_N__R.vi"() -> ("output_Audio_N__R"=w869:i32)  [unwired: 11 in]
                      n609 = Boolean To (0,1)(Boolean=w883) -> (0, 1=w882:i16)
                      n610 = To Unsigned Word Integer(number=w882) -> (unsigned 16bit integer=w881:u16)
                      n611 = Not Equal?(x=u16 1, y=w879) -> (x != y?=w878:bool)
                      n612 = Not Equal To 0?(x=w879) -> (x != 0?=w877:bool)
                      n613 = And(x=w878, y=w876) -> (x .and. y?=w874:bool)
                      n614 = And(x=w877, y=w876) -> (x .and. y?=w872:bool)
                      n615 = Boolean To (0,1)(Boolean=w874) -> (0, 1=w875:i16)
                      n616 = Boolean To (0,1)(Boolean=w872) -> (0, 1=w873:i16)
                      n617 = To Unsigned Word Integer(number=w875) -> (unsigned 16bit integer=w870:u16)
                      n618 = To Unsigned Word Integer(number=w873) -> (unsigned 16bit integer=w868:u16)
                      n619 = Replace Array Subset(array=w887, new element #1=u16 1 ("new element/subarray"), index #1=w886, new element #2=w881, index #2=w884, new element #3=w870, index #3=w871, new element #4=w868, index #4=w869) -> (w888:u16[])
                    }
                    frame False {
                      n620 = call "myRIO_BRig_RT_dataMTrig_Solenoid_N__L.vi"() -> ("output_Solenoid_N__L"=w896:i32)  [unwired: 11 in]
                      n621 = Index Array(array=w899, index=w896) -> (element=w897:u16)
                      n622 = Increment(x=w897) -> (x+1=w895:u16)
                      n623 = Replace Array Subset(array=w899, new element=w895, index=w896) -> (w898:u16[])
                    }
                  }
                  n624 = local write "MTrig_Solenoid_trig__L"(FALSE) -> ()
                }
                frame 2 {
                  n625 = case shown="True" w901 {
                    tunnel: [w927 w938] -> w903
                    tunnel: w902 -> [w907 w934]
                    tunnel: w900 -> [w906 _]
                    frame True {
                      n626 = case shown="2" w906 {
                        tunnel: [TRUE _ w931 w933] -> w916
                        tunnel: [_ TRUE w930 w933] -> w923
                        frame 0, Default {
                          # "Audio"
                        }
                        frame 1 {
                          # "LED"
                        }
                        frame 2 {
                          # "Audio or LED"
                          n627 = local read "Cue1Param_AudioLed_Probability_Switch"() -> (w932:u16)
                          n628 = call "myRIO__convert__Probability_to_TrueFalse.vi"("input_probability_u16"=w932) -> ("output_TF"=w930:bool)  [unwired: 10 in]
                          n629 = Not(x=w930) -> (.not. x?=w931:bool)
                        }
                        frame 3 {
                          w933 = TRUE
                          # "Audio and LED"
                        }
                      }
                      n630 = local read "sp_RightSpout"() -> (w919:u16)
                      n631 = call "myRIO_BRig_RT_dataMTrig_Solenoid_N__R.vi"() -> ("output_Solenoid_N__R"=w926:i32)  [unwired: 11 in]
                      n632 = call "myRIO_BRig_RT_dataMTrig_CueLed_N.vi"() -> ("output_CueLed_N"=w924:i32)  [unwired: 11 in]
                      n633 = call "myRIO_BRig_RT_dataMTrig_Audio_N__L.vi"() -> ("output_Audio_N__L"=w911:i32)  [unwired: 11 in]
                      n634 = call "myRIO_BRig_RT_dataMTrig_Audio_N__R.vi"() -> ("output_Audio_N__R"=w909:i32)  [unwired: 11 in]
                      n635 = Boolean To (0,1)(Boolean=w923) -> (0, 1=w922:i16)
                      n636 = To Unsigned Word Integer(number=w922) -> (unsigned 16bit integer=w921:u16)
                      n637 = Not Equal?(x=u16 1, y=w919) -> (x != y?=w918:bool)
                      n638 = Not Equal To 0?(x=w919) -> (x != 0?=w917:bool)
                      n639 = And(x=w918, y=w916) -> (x .and. y?=w914:bool)
                      n640 = And(x=w917, y=w916) -> (x .and. y?=w912:bool)
                      n641 = Boolean To (0,1)(Boolean=w914) -> (0, 1=w915:i16)
                      n642 = Boolean To (0,1)(Boolean=w912) -> (0, 1=w913:i16)
                      n643 = To Unsigned Word Integer(number=w915) -> (unsigned 16bit integer=w910:u16)
                      n644 = To Unsigned Word Integer(number=w913) -> (unsigned 16bit integer=w908:u16)
                      n645 = Replace Array Subset(array=w907, new element #1=u16 1 ("new element/subarray"), index #1=w926, new element #2=w921, index #2=w924, new element #3=w910, index #3=w911, new element #4=w908, index #4=w909) -> (w927:u16[])
                    }
                    frame False {
                      n646 = call "myRIO_BRig_RT_dataMTrig_Solenoid_N__R.vi"() -> ("output_Solenoid_N__R"=w936:i32)  [unwired: 11 in]
                      n647 = Index Array(array=w934, index=w936) -> (element=w935:u16)
                      n648 = Increment(x=w935) -> (x+1=w937:u16)
                      n649 = Replace Array Subset(array=w934, new element=w937, index=w936) -> (w938:u16[])
                    }
                  }
                  n650 = local write "MTrig_Solenoid_trig__R"(FALSE) -> ()
                }
                frame 3 {
                  w943 = FALSE
                  n651 = case shown="True" w942 {
                    tunnel: [w959 w973] -> w940
                    tunnel: w941 -> [w950 _]
                    tunnel: w939 -> [w949 w969]
                    frame True {
                      w945 = u16 1 ("new element/subarray")
                      n652 = case shown="3" w950 {
                        tunnel: [TRUE _ w963 w965] -> w948
                        tunnel: [_ TRUE w962 w965] -> w956
                        frame 0, Default {
                          # "Audio"
                        }
                        frame 1 {
                          # "LED"
                        }
                        frame 2 {
                          # "Audio or LED"
                          n653 = local read "Cue1Param_AudioLed_Probability_Switch"() -> (w964:u16)
                          n654 = call "myRIO__convert__Probability_to_TrueFalse.vi"("input_probability_u16"=w964) -> ("output_TF"=w962:bool)  [unwired: 10 in]
                          n655 = Not(x=w962) -> (.not. x?=w963:bool)
                        }
                        frame 3 {
                          w965 = TRUE
                          # "Audio and LED"
                        }
                      }
                      n656 = call "myRIO_BRig_RT_dataMTrig_Solenoid_N__R.vi"() -> ("output_Solenoid_N__R"=w946:i32)  [unwired: 11 in]
                      n657 = call "myRIO_BRig_RT_dataMTrig_Solenoid_N__L.vi"() -> ("output_Solenoid_N__L"=w958:i32)  [unwired: 11 in]
                      n658 = call "myRIO_BRig_RT_dataMTrig_CueLed_N.vi"() -> ("output_CueLed_N"=w957:i32)  [unwired: 11 in]
                      n659 = call "myRIO_BRig_RT_dataMTrig_Audio_N__L.vi"() -> ("output_Audio_N__L"=w952:i32)  [unwired: 11 in]
                      n660 = call "myRIO_BRig_RT_dataMTrig_Audio_N__R.vi"() -> ("output_Audio_N__R"=w951:i32)  [unwired: 11 in]
                      n661 = Boolean To (0,1)(Boolean=w956) -> (0, 1=w955:i16)
                      n662 = To Unsigned Word Integer(number=w955) -> (unsigned 16bit integer=w954:u16)
                      n663 = Boolean To (0,1)(Boolean=w948) -> (0, 1=w953:i16)
                      n664 = To Unsigned Word Integer(number=w953) -> (unsigned 16bit integer=w947:u16)
                      n665 = Replace Array Subset(array=w949, new element #1=w945, index #1=w946, new element #2=w945, index #2=w958, new element #3=w954, index #3=w957, new element #4=w947, index #4=w952, new element #5=w947, index #5=w951) -> (w959:u16[])
                    }
                    frame False {
                      n666 = call "myRIO_BRig_RT_dataMTrig_Solenoid_N__L.vi"() -> ("output_Solenoid_N__L"=w972:i32)  [unwired: 11 in]
                      n667 = call "myRIO_BRig_RT_dataMTrig_Solenoid_N__R.vi"() -> ("output_Solenoid_N__R"=w968:i32)  [unwired: 11 in]
                      n668 = Index Array(array=w969, index #1=w972, index #2=w968) -> (element #1=w970:u16, element #2=w967:u16)
                      n669 = Increment(x=w970) -> (x+1=w971:u16)
                      n670 = Increment(x=w967) -> (x+1=w966:u16)
                      n671 = Replace Array Subset(array=w969, new element #1=w971, index #1=w972, new element #2=w966, index #2=w968) -> (w973:u16[])
                    }
                  }
                  n672 = local write "MTrig_Solenoid_trig__L"(w943) -> ()
                  n673 = local write "MTrig_Solenoid_trig__R"(w943) -> ()
                }
              }
              n674 = local read "get_countPerMS"() -> (w841:bool)
              n675 = Select(t=myRIO_BRig_RT__Case_NonExp_stateList."Cue_pre", s=w844, f=myRIO_BRig_RT__Case_NonExp_stateList."DispenseWater_pre" ("Enum")) -> (s? t:f=w842:T1)
              n676 = Select(t=myRIO_BRig_RT__Case_NonExp_stateList."Get_FPGA_count_per_ms" ("Enum"), s=w841, f=myRIO_BRig_RT__Case_NonExp_stateList."Idle_6" ("Enum")) -> (s? t:f=w839:T1)
              n677 = Select(t=w842, s=w846, f=w839) -> (s? t:f=w847:T1)
            }
            frame "Idle_6" {
              # "There are a number of tasks we need to perform\nwhile idling. To preserve our timing loop, we\nbreak up the IDLE state into smaller states"
              # "use dataMTrig as it is one of the last to transfer"
              n678 = call "myRIO_BRig_RT_comm_webdav_uploadReceived_check_v2,0.vi"("input_dataName"="dataMTrig") -> ("output_Iexist"=w978:bool)  [unwired: 9 in, 1 out]
              n679 = Select(t=myRIO_BRig_RT__Case_NonExp_stateList."UploadSettings_pre" ("Enum"), s=w978, f=myRIO_BRig_RT__Case_NonExp_stateList."Idle") -> (s? t:f=w976:T1)
            }
            frame "Cue_pre" {
              w986 = u16 0 ("new element/subarray")
              # "Audio cue or LED cue?"
              # "Audio, LED, or \"Audio or LED\""
              # "Right Audio?"
              # "Left Audio?"
              # "Left or Right?"
              # "Cue Audio?\n(T=Audio, F=LED)"
              # "Ncycle"
              # "count"
              # "Audio_R"
              # "Ncycle"
              # "count"
              # "Audio_L"
              n680 = local read "Cue1Param_CueType_Switch"() -> (w1007:u16)
              n681 = case shown="3" w1007 {
                tunnel: [TRUE _ w1027 w1029] -> w982
                tunnel: [_ TRUE w1026 w1029] -> w981
                frame 0, Default {
                  # "Audio"
                }
                frame 1 {
                  # "LED"
                }
                frame 2 {
                  # "Audio or LED"
                  n682 = local read "Cue1Param_AudioLed_Probability_Switch"() -> (w1028:u16)
                  n683 = call "myRIO__convert__Probability_to_TrueFalse.vi"("input_probability_u16"=w1028) -> ("output_TF"=w1026:bool)  [unwired: 10 in]
                  n684 = Not(x=w1026) -> (.not. x?=w1027:bool)
                }
                frame 3 {
                  w1029 = TRUE
                }
              }
              n685 = call "myRIO_BRig_RT_dataMTrig_Solenoid_N__L.vi"() -> ("output_Solenoid_N__L"=w1017:i32)  [unwired: 11 in]
              n686 = call "myRIO_BRig_RT_dataMTrig_Solenoid_N__R.vi"() -> ("output_Solenoid_N__R"=w1016:i32)  [unwired: 11 in]
              n687 = Index Array(array=w1013, index #1=w1017, index #2=w1016) -> (element #1=w1015:u16, element #2=w1014:u16)
              n688 = Not Equal To 0?(x=w1015) -> (x != 0?=w1006:bool)
              n689 = Not Equal To 0?(x=w1014) -> (x != 0?=w1005:bool)
              n690 = And(x=w982, y=w1006) -> (x .and. y?=w1000:bool)
              n691 = And(x=w982, y=w1005) -> (x .and. y?=w998:bool)
              n692 = local read "sp_RightSpout"() -> (w999:u16)
              n693 = local read "sp_LeftSpout"() -> (w1001:u16)
              n694 = Boolean To (0,1)(Boolean=w981) -> (0, 1=w984:i16)
              n695 = To Unsigned Word Integer(number=w984) -> (unsigned 16bit integer=w983:u16)
              n696 = case shown="0, Default" w1001 {
                tunnel: [w1021 _ w1023] -> w997
                tunnel: [_ w1022 w1023] -> w995
                tunnel: w1000 -> [w1021 w1022 w1023]
                frame 0, Default {
                }
                frame 1 {
                }
                frame 2 {
                }
              }
              n697 = case shown="0, Default" w999 {
                tunnel: [w1018 _ w1020] -> w996
                tunnel: [_ w1019 w1020] -> w994
                tunnel: w998 -> [w1018 w1019 w1020]
                frame 0, Default {
                }
                frame 1 {
                }
                frame 2 {
                }
              }
              n698 = call "myRIO_BRig_RT_dataMTrig_Audio_c__L.vi"() -> ("output_Audio_c__L"=w1011:i32)  [unwired: 11 in]
              n699 = call "myRIO_BRig_RT_dataMTrig_Audio_N__L.vi"() -> ("output_Audio_N__L"=w1010:i32)  [unwired: 11 in]
              n700 = call "myRIO_BRig_RT_dataMTrig_Audio_c__R.vi"() -> ("output_Audio_c__R"=w1009:i32)  [unwired: 11 in]
              n701 = call "myRIO_BRig_RT_dataMTrig_Audio_N__R.vi"() -> ("output_Audio_N__R"=w1008:i32)  [unwired: 11 in]
              n702 = call "myRIO_BRig_RT_dataMTrig_CueLed_c.vi"() -> ("output_CueLed_c"=w987:i32)  [unwired: 11 in]
              n703 = call "myRIO_BRig_RT_dataMTrig_CueLed_N.vi"() -> ("output_CueLed_N"=w985:i32)  [unwired: 11 in]
              n704 = Or(x=w997, y=w996) -> (x .or. y?=w993:bool)
              n705 = Boolean To (0,1)(Boolean=w993) -> (0, 1=w991:i16)
              n706 = To Unsigned Word Integer(number=w991) -> (unsigned 16bit integer=w990:u16)
              n707 = Or(x=w995, y=w994) -> (x .or. y?=w992:bool)
              n708 = Boolean To (0,1)(Boolean=w992) -> (0, 1=w989:i16)
              n709 = To Unsigned Word Integer(number=w989) -> (unsigned 16bit integer=w988:u16)
              n710 = Replace Array Subset(array=w1013, new element #1=w986, index #1=w1011, new element #2=w990, index #2=w1010, new element #3=w986, index #3=w1009, new element #4=w988, index #4=w1008, new element #5=w986, index #5=w987, new element #6=w983, index #6=w985) -> (w1012:u16[])
              n711 = Initialize Array(u16 0 ("element"), 1 ("dimension size")) -> (w1004:u16[])
            }
            frame "Cue" {
              # "warmupType\n0 = Cue with reward (not possible to be in this state with value==0)\n1 = Cue then reward\n2 = Cue then reward (no lick)"
              # "lick did not occur or warmupType==1"
              # "lick occurred?"
              # "Ncycle"
              # "Audio_R"
              # "Ncycle"
              # "Audio_L"
              n712 = local read "warmupType"() -> (w1039:u8)
              n713 = Greater?(x=w1045, y=w1044) -> (0:w1048:bool)
              n714 = Greater?(x=w1047, y=w1046) -> (0:w1043:bool)
              n715 = Or(x=w1043, y=w1048) -> (x .or. y?=w1037:bool)
              n716 = Equal?(x=w1039, y=u8 1) -> (x = y?=w1033:bool)
              n717 = Not(x=w1037) -> (.not. x?=w1036:bool)
              n718 = call "myRIO_BRig_RT_dataMTrig_Audio_N__L.vi"() -> ("output_Audio_N__L"=w1050:i32)  [unwired: 11 in]
              n719 = call "myRIO_BRig_RT_dataMTrig_Audio_N__R.vi"() -> ("output_Audio_N__R"=w1049:i32)  [unwired: 11 in]
              n720 = call "myRIO_BRig_RT_dataMTrig_CueLed_N.vi"() -> ("output_CueLed_N"=w1030:i32)  [unwired: 11 in]
              n721 = Or(x=w1036, y=w1033) -> (x .or. y?=w1034:bool)
              n722 = case shown="True" w1034 {
                tunnel: w1050 -> [w1056 w1077]
                tunnel: w1049 -> [w1055 w1076]
                tunnel: w1042 -> [w1058 w1071]
                tunnel: [w1057 w1071] -> w1041
                tunnel: w1040 -> [_ w1069]
                tunnel: [myRIO_BRig_RT__Case_NonExp_stateList."Idle" ("t") w1068] -> w1035
                tunnel: w1033 -> [_ w1067]
                tunnel: w1032 -> [_ w1063]
                tunnel: w1031 -> [_ w1062]
                tunnel: w1030 -> [_ w1061]
                frame False {
                  w1051 = u16 0 ("new element/subarray")
                  # "lick occurred and warmupType==2"
                  n723 = call "myRIO_BRig_RT_dataMTrig_Solenoid_N__R.vi"() -> ("output_Solenoid_N__R"=w1052:i32)  [unwired: 11 in]
                  n724 = call "myRIO_BRig_RT_dataMTrig_Solenoid_N__L.vi"() -> ("output_Solenoid_N__L"=w1053:i32)  [unwired: 11 in]
                  n725 = Replace Array Subset(array=w1058, new element #1=w1051, index #1=w1056, new element #2=w1051, index #2=w1055, new element #3=w1051, index #3=w1053, new element #4=w1051, index #4=w1052) -> (w1057:u16[])
                }
                frame True {
                  n726 = Not(x=w1067) -> (.not. x?=w1066:bool)
                  n727 = Index Array(array=w1071, index #1=w1077, index #2=w1076, index #3=w1061) -> (element #1=w1075:u16, element #2=w1074:u16, element #3=w1060:u16)
                  n728 = Equal To 0?(x=w1075) -> (x = 0?=w1073:bool)
                  n729 = Equal To 0?(x=w1074) -> (x = 0?=w1072:bool)
                  n730 = Equal To 0?(x=w1060) -> (x = 0?=w1059:bool)
                  n731 = Compound Arithmetic op=AND(w1073, w1072, w1059) -> (w1065:bool)
                  n732 = And(x=w1065, y=w1066) -> (x .and. y?=w1064:bool)
                  n733 = case shown="True" w1064 {
                    tunnel: w1063 -> [_ w1085]
                    tunnel: w1062 -> [_ w1080]
                    frame False {
                    }
                    frame True {
                      n734 = local read "count_warmup_R"() -> (w1078:u16)
                      n735 = local read "count_warmup_L"() -> (w1083:u16)
                      n736 = Increment(x=w1078) -> (x+1=w1081:u16)
                      n737 = Increment(x=w1083) -> (x+1=w1084:u16)
                      n738 = Select(t=w1081, s=w1080, f=w1078) -> (s? t:f=w1079:u16)
                      n739 = Select(t=w1084, s=w1085, f=w1083) -> (s? t:f=w1082:u16)
                      n740 = local write "count_warmup_R"(w1079) -> ()
                      n741 = local write "count_warmup_L"(w1082) -> ()
                    }
                  }
                  n742 = Select(t=myRIO_BRig_RT__Case_NonExp_stateList."DispenseWater_pre", s=w1065, f=w1069) -> (s? t:f=w1068:T1)
                }
              }
            }
            frame "RewardCalibration_pre" {
              (unwired) FALSE
              w1086 = FALSE
              w1097 = u8 0
              w1113 = u8 0
              # "Are we starting a RewardCalibration?\nOr are we stopping a RewardCalibration?\nOr is a RewardCalibration over?"
              # "RewCalib\nOnOff"
              # "N"
              # "Solenoid R"
              # "RewCalib\nOnOff"
              # "N"
              # "Solenoid L"
              n743 = local read "RewCalib_Trig_L"() -> (w1120:bool)
              n744 = local read "RewCalib_Trig_R"() -> (w1089:bool)
              n745 = call "myRIO_BRig_RT_dataMTrig_Solenoid_N__R.vi"() -> ("output_Solenoid_N__R"=w1091:i32)  [unwired: 11 in]
              n746 = call "myRIO_BRig_RT_dataMTrig_Solenoid_RewCalib_OnOff__R.vi"() -> ("output_Solenoid_RewCalib_OnOff__R"=w1088:i32)  [unwired: 11 in]
              n747 = call "myRIO_BRig_RT_dataMTrig_Solenoid_N__L.vi"() -> ("output_Solenoid_N__L"=w1106:i32)  [unwired: 11 in]
              n748 = call "myRIO_BRig_RT_dataMTrig_Solenoid_RewCalib_OnOff__L.vi"() -> ("output_Solenoid_RewCalib_OnOff__L"=w1107:i32)  [unwired: 11 in]
              n749 = Index Array(array=w1090, index #1=w1091, index #2=w1088) -> (element #1=w1101:u16, element #2=w1096:u16)
              n750 = Index Array(array=w1090, index #1=w1106, index #2=w1107) -> (element #1=w1117:u16, element #2=w1112:u16)
              n751 = Equal To 0?(x=w1101) -> (x = 0?=w1102:bool)
              n752 = Not Equal To 0?(x=w1096) -> (x != 0?=w1099:bool)
              n753 = Equal To 0?(x=w1117) -> (x = 0?=w1118:bool)
              n754 = Not Equal To 0?(x=w1112) -> (x != 0?=w1115:bool)
              n755 = local write "MTrig_Solenoid_trig__L"(w1086) -> ()
              n756 = local write "MTrig_Solenoid_trig__R"(w1086) -> ()
              n757 = Select(t=u8 1, s=w1089, f=w1097) -> (s? t:f=w1093:u8)
              n758 = Select(t=u8 1, s=w1120, f=w1113) -> (s? t:f=w1109:u8)
              n759 = Select(t=u8 2, s=w1102, f=w1097) -> (s? t:f=w1094:u8)
              n760 = Select(t=u8 4, s=w1099, f=w1097) -> (s? t:f=w1095:u8)
              n761 = Select(t=u8 2, s=w1118, f=w1113) -> (s? t:f=w1110:u8)
              n762 = Select(t=u8 4, s=w1115, f=w1113) -> (s? t:f=w1111:u8)
              n763 = Compound Arithmetic op=ADD(w1093, w1094, w1095) -> (w1092:u8)
              n764 = Compound Arithmetic op=ADD(w1109, w1110, w1111) -> (w1108:u8)
              n765 = case shown="7" w1108 {
                tunnel: w1090 -> [w1150 w1155 w1157 w1162 w1167 w1169 w1172 w1177]
                tunnel: [w1150 w1156 w1157 w1163 w1168 w1169 w1173 w1178] -> w1105
                tunnel: w1107 -> [_ w1153 _ w1160 w1165 _ w1171 w1176]
                tunnel: w1106 -> [_ w1154 _ w1161 w1166 _ _ _]
                frame 0, Default {
                }
                frame 1 {
                  n766 = Replace Array Subset(array=w1155, new element #1=u16 100 ("new element/subarray"), index #1=w1154, new element #2=u16 1 ("new element/subarray"), index #2=w1153) -> (w1156:u16[])
                }
                frame 2 {
                }
                frame 3 {
                  n767 = Replace Array Subset(array=w1162, new element #1=u16 100 ("new element/subarray"), index #1=w1161, new element #2=u16 1 ("new element/subarray"), index #2=w1160) -> (w1163:u16[])
                }
                frame 4 {
                  w1164 = u16 0 ("new element/subarray")
                  n768 = Replace Array Subset(array=w1167, new element #1=w1164, index #1=w1166, new element #2=w1164, index #2=w1165) -> (w1168:u16[])
                }
                frame 5 {
                }
                frame 6 {
                  n769 = Replace Array Subset(array=w1172, new element=u16 0 ("new element/subarray"), index=w1171) -> (w1173:u16[])
                }
                frame 7 {
                  n770 = local write "RewCalib_Trig_L"(FALSE ("RewCalib_Trig_L")) -> ()
                  n771 = Replace Array Subset(array=w1177, new element=u16 0 ("new element/subarray"), index=w1176) -> (w1178:u16[])
                }
              }
              n772 = case shown="7" w1092 {
                tunnel: w1105 -> [w1121 w1126 w1128 w1133 w1138 w1140 w1143 w1148]
                tunnel: [w1121 w1127 w1128 w1134 w1139 w1140 w1144 w1149] -> w1104
                tunnel: w1088 -> [_ w1124 _ w1131 w1136 _ w1142 w1147]
                tunnel: w1091 -> [_ w1125 _ w1132 w1137 _ _ _]
                frame 0, Default {
                }
                frame 1 {
                  n773 = Replace Array Subset(array=w1126, new element #1=u16 100 ("new element/subarray"), index #1=w1125, new element #2=u16 1 ("new element/subarray"), index #2=w1124) -> (w1127:u16[])
                }
                frame 2 {
                }
                frame 3 {
                  n774 = Replace Array Subset(array=w1133, new element #1=u16 100 ("new element/subarray"), index #1=w1132, new element #2=u16 1 ("new element/subarray"), index #2=w1131) -> (w1134:u16[])
                }
                frame 4 {
                  w1135 = u16 0 ("new element/subarray")
                  n775 = Replace Array Subset(array=w1138, new element #1=w1135, index #1=w1137, new element #2=w1135, index #2=w1136) -> (w1139:u16[])
                }
                frame 5 {
                }
                frame 6 {
                  n776 = Replace Array Subset(array=w1143, new element=u16 0 ("new element/subarray"), index=w1142) -> (w1144:u16[])
                }
                frame 7 {
                  n777 = local write "RewCalib_Trig_R"(FALSE ("RewCalib_Trig_L")) -> ()
                  n778 = Replace Array Subset(array=w1148, new element=u16 0 ("new element/subarray"), index=w1147) -> (w1149:u16[])
                }
              }
            }
            frame "DispenseWater_pre" {
              w1184 = u16 0 ("t")
              w1227 = u16 0 ("new element/subarray")
              # "just trust me on this one"
              # "RewCalib\nOnOff"
              # "RewCalib\nOnOff"
              # "nCycle"
              # "Solenoid__R"
              # "Tdelay"
              # "delay"
              # "nCycle"
              # "Solenoid__L"
              # "Tdelay"
              # "delay"
              # "Solenoid__R"
              # "count"
              # "Solenoid_Tcycle_R"
              # "Solenoid_Tcycle_L"
              # "Solenoid__L"
              # "count"
              n779 = call "myRIO_BRig_RT_dataMTrig_Solenoid_RewCalib_OnOff__L.vi"() -> ("output_Solenoid_RewCalib_OnOff__L"=w1191:i32)  [unwired: 11 in]
              n780 = call "myRIO_BRig_RT_dataMTrig_Solenoid_N__L.vi"() -> ("output_Solenoid_N__L"=w1182:i32)  [unwired: 11 in]
              n781 = call "myRIO_BRig_RT_dataMTrig_Solenoid_delay__L.vi"() -> ("output_Solenoid_delay__L"=w1225:i32)  [unwired: 11 in]
              n782 = call "myRIO_BRig_RT_dataMTrig_Solenoid_Tdelay__L.vi"() -> ("output_Solenoid_Tdelay__L"=w1224:i32)  [unwired: 11 in]
              n783 = call "myRIO_BRig_RT_dataMTrig_Solenoid_N__R.vi"() -> ("output_Solenoid_N__R"=w1180:i32)  [unwired: 11 in]
              n784 = call "myRIO_BRig_RT_dataMTrig_Solenoid_delay__R.vi"() -> ("output_Solenoid_delay__R"=w1214:i32)  [unwired: 11 in]
              n785 = call "myRIO_BRig_RT_dataMTrig_Solenoid_Tdelay__R.vi"() -> ("output_Solenoid_Tdelay__R"=w1213:i32)  [unwired: 11 in]
              n786 = call "myRIO_BRig_RT_dataMTrig_Solenoid_RewCalib_OnOff__R.vi"() -> ("output_Solenoid_RewCalib_OnOff__R"=w1187:i32)  [unwired: 11 in]
              n787 = Index Array(array=w1226, index #1=w1182, index #2=w1225, index #3=w1224, index #4=w1180, index #5=w1214, index #6=w1213, index #7=w1191, index #8=w1187) -> (element #1=w1183:u16, element #2=w1223:u16, element #3=w1218:u16, element #4=w1186:u16, element #5=w1208:u16, element #6=w1207:u16, element #7=w1192:u16, element #8=w1189:u16)
              n788 = Equal To 0?(x=w1223) -> (x = 0?=w1222:bool)
              n789 = Equal To 0?(x=w1208) -> (x = 0?=w1212:bool)
              n790 = local read "RewCalib_Trig_L"() -> (w1203:bool)
              n791 = local read "RewCalib_Trig_R"() -> (w1198:bool)
              n792 = Not Equal To 0?(x=w1183) -> (x != 0?=w1221:bool)
              n793 = Not Equal To 0?(x=w1186) -> (x != 0?=w1211:bool)
              n794 = local read "MTrig_Solenoid_Tcycle__L"() -> (w1220:u16)
              n795 = local read "MTrig_Solenoid_Tcycle__R"() -> (w1206:u16)
              n796 = Not Equal To 0?(x=w1192) -> (x != 0?=w1202:bool)
              n797 = Not Equal To 0?(x=w1189) -> (x != 0?=w1200:bool)
              n798 = Not(x=w1203) -> (.not. x?=w1201:bool)
              n799 = Not(x=w1198) -> (.not. x?=w1199:bool)
              n800 = And(x=w1202, y=w1201) -> (x .and. y?=w1197:bool)
              n801 = And(x=w1200, y=w1199) -> (x .and. y?=w1196:bool)
              n802 = call "myRIO_BRig_RT_dataMTrig_Solenoid_c__L.vi"() -> ("output_Solenoid_c__L"=w1229:i32)  [unwired: 11 in]
              n803 = call "myRIO_BRig_RT_dataMTrig_Solenoid_c__R.vi"() -> ("output_Solenoid_c__R"=w1228:i32)  [unwired: 11 in]
              n804 = Select(t=w1220, s=w1221, f=u16 0) -> (s? t:f=w1217:u16)
              n805 = Or(x=w1197, y=w1196) -> (x .or. y?=w1185:bool)
              n806 = Select(t=w1206, s=w1211, f=u16 0) -> (s? t:f=w1209:u16)
              n807 = Select(t=w1217, s=w1222, f=w1218) -> (s? t:f=w1215:u16)
              n808 = Select(t=w1209, s=w1212, f=w1207) -> (s? t:f=w1204:u16)
              n809 = call "myRIO_BRig_RT_dataMTrig_Solenoid_Tcycle__L.vi"() -> ("output_Solenoid_Tcycle__L"=w1216:i32)  [unwired: 11 in]
              n810 = call "myRIO_BRig_RT_dataMTrig_Solenoid_Tcycle__R.vi"() -> ("output_Solenoid_Tcycle__R"=w1205:i32)  [unwired: 11 in]
              n811 = Select(t=w1184, s=w1185, f=w1183) -> (s? t:f=w1181:u16)
              n812 = Select(t=w1184, s=w1185, f=w1186) -> (s? t:f=w1179:u16)
              n813 = Select(t=myRIO_BRig_RT__Case_NonExp_stateList."Idle" ("Enum"), s=w1185, f=myRIO_BRig_RT__Case_NonExp_stateList."DispenseWater" ("Enum")) -> (s? t:f=w1193:T1)
              n814 = Select(t=w1184, s=w1185, f=w1192) -> (s? t:f=w1190:u16)
              n815 = Select(t=w1184, s=w1185, f=w1189) -> (s? t:f=w1188:u16)
              n816 = Replace Array Subset(array=w1226, new element #1=w1227, index #1=w1229, new element #2=w1227, index #2=w1228, new element #3=w1215, index #3=w1216, new element #4=w1204, index #4=w1205, new element #5=w1190, index #5=w1191, new element #6=w1188, index #6=w1187, new element #7=w1181, index #7=w1182, new element #8=w1179, index #8=w1180) -> (w1230:u16[])
            }
            frame "DispenseWater" {
              # "D"
              # "C"
              # "B"
              # "A"
              # "(A) Add COUNT and INCREMENT\n(B) Is (A) smaller than Tcycle?\n(C) Are we dispensing water or in the delay phase?\n(D) If (A) is smaller than Tcycle   AND   if we are dispensing water\n      then send TRUE to solenoid"
              # "delay"
              # "Tcycle"
              # "Solenoid__R"
              # "count"
              # "delay"
              # "Tcycle"
              # "Solenoid__L"
              # "count"
              n817 = To Unsigned Word Integer(number=w1257) -> (unsigned 16bit integer=w1239:u16)
              n818 = call "myRIO_BRig_RT_dataMTrig_Solenoid_delay__R.vi"() -> ("output_Solenoid_delay__R"=w1243:i32)  [unwired: 11 in]
              n819 = call "myRIO_BRig_RT_dataMTrig_Solenoid_c__R.vi"() -> ("output_Solenoid_c__R"=w1242:i32)  [unwired: 11 in]
              n820 = call "myRIO_BRig_RT_dataMTrig_Solenoid_Tcycle__R.vi"() -> ("output_Solenoid_Tcycle__R"=w1244:i32)  [unwired: 11 in]
              n821 = call "myRIO_BRig_RT_dataMTrig_Solenoid_delay__L.vi"() -> ("output_Solenoid_delay__L"=w1259:i32)  [unwired: 11 in]
              n822 = call "myRIO_BRig_RT_dataMTrig_Solenoid_c__L.vi"() -> ("output_Solenoid_c__L"=w1251:i32)  [unwired: 11 in]
              n823 = call "myRIO_BRig_RT_dataMTrig_Solenoid_Tcycle__L.vi"() -> ("output_Solenoid_Tcycle__L"=w1260:i32)  [unwired: 11 in]
              n824 = Index Array(array=w1253, index #1=w1251, index #2=w1260, index #3=w1259, index #4=w1242, index #5=w1244, index #6=w1243) -> (element #1=w1258:u16, element #2=w1248:u16, element #3=w1256:u16, element #4=w1238:u16, element #5=w1235:u16, element #6=w1234:u16)
              n825 = Add(x=w1258, y=w1239) -> (x+y=w1249:u16)
              n826 = Add(x=w1238, y=w1239) -> (x+y=w1240:u16)
              n827 = Less?(x=w1249, y=w1248) -> (x < y?=w1232:bool)
              n828 = Equal To 0?(x=w1256) -> (x = 0?=w1255:bool)
              n829 = Less?(x=w1240, y=w1235) -> (x < y?=w1233:bool)
              n830 = Equal To 0?(x=w1234) -> (x = 0?=w1241:bool)
              n831 = And(x=w1232, y=w1255) -> (x .and. y?=w1254:bool)
              n832 = Or(x=w1232, y=w1233) -> (x .or. y?=w1231:bool)
              n833 = And(x=w1233, y=w1241) -> (x .and. y?=w1236:bool)
              n834 = Select(t=w1249, s=w1232, f=w1248) -> (s? t:f=w1250:u16)
              n835 = Select(t=w1240, s=w1233, f=w1235) -> (s? t:f=w1237:u16)
              n836 = Replace Array Subset(array=w1253, new element #1=w1250, index #1=w1251, new element #2=w1237, index #2=w1242) -> (w1252:u16[])
              n837 = Select(t=w1247, s=w1231, f=myRIO_BRig_RT__Case_NonExp_stateList."DispenseWater_post" ("Enum")) -> (s? t:f=w1245:T1)
            }
            frame "DispenseWater_post" {
              # "nCycle"
              # "delay"
              # "Solenoid__R"
              # "nCycle"
              # "delay"
              # "Solenoid__L"
              n838 = call "myRIO_BRig_RT_dataMTrig_Solenoid_N__L.vi"() -> ("output_Solenoid_N__L"=w1277:i32)  [unwired: 11 in]
              n839 = call "myRIO_BRig_RT_dataMTrig_Solenoid_delay__L.vi"() -> ("output_Solenoid_delay__L"=w1276:i32)  [unwired: 11 in]
              n840 = call "myRIO_BRig_RT_dataMTrig_Solenoid_N__R.vi"() -> ("output_Solenoid_N__R"=w1273:i32)  [unwired: 11 in]
              n841 = call "myRIO_BRig_RT_dataMTrig_Solenoid_delay__R.vi"() -> ("output_Solenoid_delay__R"=w1272:i32)  [unwired: 11 in]
              n842 = Index Array(array=w1279, index #1=w1277, index #2=w1276, index #3=w1273, index #4=w1272) -> (element #1=w1281:u16, element #2=w1280:u16, element #3=w1264:u16, element #4=w1266:u16)
              n843 = Not Equal To 0?(x=w1281) -> (x != 0?=w1282:bool)
              n844 = Not Equal To 0?(x=w1264) -> (x != 0?=w1265:bool)
              n845 = case shown="True" w1265 {
                selector: w1265 -> [_ w1286]
                tunnel: w1264 -> [w1284 w1292]
                tunnel: w1266 -> [_ w1293]
                tunnel: [w1284 w1290] -> w1263
                tunnel: [u16 0 w1289] -> w1262
                tunnel: [_ w1286] -> w1261
                frame False {
                }
                frame True {
                  n846 = Equal To 0?(x=w1293) -> (x = 0?=w1285:bool)
                  n847 = Decrement(x=w1292) -> (x-1=w1291:u16)
                  n848 = Select(t=w1291, s=w1285, f=w1292) -> (s? t:f=w1290:u16)
                  n849 = Select(t=u16 1, s=w1285, f=u16 0) -> (s? t:f=w1289:u16)
                }
              }
              n850 = case shown="True" w1282 {
                selector: w1282 -> [_ w1297]
                tunnel: w1281 -> [w1295 w1303]
                tunnel: w1280 -> [_ w1304]
                tunnel: [w1295 w1301] -> w1275
                tunnel: [u16 0 w1300] -> w1274
                tunnel: [_ w1297] -> w1271
                frame False {
                }
                frame True {
                  n851 = Equal To 0?(x=w1304) -> (x = 0?=w1296:bool)
                  n852 = Decrement(x=w1303) -> (x-1=w1302:u16)
                  n853 = Select(t=w1302, s=w1296, f=w1303) -> (s? t:f=w1301:u16)
                  n854 = Select(t=u16 1, s=w1296, f=u16 0) -> (s? t:f=w1300:u16)
                }
              }
              n855 = Or(x=w1271, y=w1261) -> (x .or. y?=w1270:bool)
              n856 = Replace Array Subset(array=w1279, new element #1=w1275, index #1=w1277, new element #2=w1274, index #2=w1276, new element #3=w1263, index #3=w1273, new element #4=w1262, index #4=w1272) -> (w1278:u16[])
              n857 = Select(t=myRIO_BRig_RT__Case_NonExp_stateList."DispenseWater_pre" ("Enum"), s=w1270, f=myRIO_BRig_RT__Case_NonExp_stateList."Idle" ("Enum")) -> (s? t:f=w1267:T1)
            }
            frame "TestConnection" {
              n858 = local read "Host Password"() -> (w1310:string)
              n859 = local read "Host UserName"() -> (w1311:string)
              n860 = call "myRIO_BRig_RT_comm_webdav_testConnect.vi"("input_password"=w1310, "input_username"=w1311) -> ("output_Iconnected"=w1308:bool)  [unwired: 9 in]
              n861 = Select(t="Connection accepted!" ("message"), s=w1308, f="Error!") -> (s? t:f=w1306:string)
              n862 = One Button Dialog(message=w1306) -> ()  [unwired: 1 in, 1 out]
            }
            frame "SendData" {
              n863 = local read "Data Set Prefix"() -> (w1313:string)
              n864 = local read "Host Password"() -> (w1314:string)
              n865 = local read "Host UserName"() -> (w1315:string)
              n866 = call "myRIO_BRig_RT_comm_webdav_sendData_all.vi"("Host Filename Prefix"=w1313, "Host Password"=w1314, "Host UserName"=w1315) -> ()  [unwired: 9 in]
            }
            frame "Get_FPGA_count_per_ms" {
              # "Used to automatically determine how many FPGA cycles in 1 ms"
              n867 = case shown="False" w1328 {
                selector: w1328 -> [w1330 _]
                tunnel: w1326 -> [_ w1343]
                tunnel: [w1334 w1343] -> w1325
                tunnel: w1324 -> [w1333 w1341]
                tunnel: w1323 -> [w1332 w1340]
                tunnel: [w1331 w1338] -> w1318
                tunnel: [w1330 w1337] -> w1322
                frame False {
                  n868 = Get Date/Time In Seconds() -> (seconds since 1Jan1904=w1335:timestamp)
                  n869 = xnode "Read/Write Control"("FPGA VI Reference In"=w1333, "error in"=w1332, "timeTrial_trig"=TRUE ("timeTrial")) -> ("error out"=w1331:errorcluster)  [unwired: 1 out]
                  n870 = To Double Precision Float(number=w1335) -> (double precision float=w1334:dbl)
                  n871 = local write "get_countPerMS"(w1330) -> ()
                }
                frame True {
                  w1339 = 1.0
                  n872 = Get Date/Time In Seconds() -> (seconds since 1Jan1904=w1344:timestamp)
                  n873 = To Double Precision Float(number=w1344) -> (double precision float=w1345:dbl)
                  n874 = Subtract(x=w1345, y=w1343) -> (x-y=w1342:dbl)
                  n875 = Less Or Equal?(x=w1339, y=w1342) -> (x <= y?=w1337:bool)
                  n876 = case shown="True" w1337 {
                    tunnel: w1341 -> [_ w1358]
                    tunnel: w1340 -> [w1346 w1357]
                    tunnel: w1339 -> [_ w1348]
                    tunnel: [w1346 w1347] -> w1338
                    frame False {
                    }
                    frame True {
                      n877 = xnode "Read/Write Control"("FPGA VI Reference In"=w1358, "error in"=w1357) -> ("FPGA VI Reference Out"=w1355:refnum<k20>, "error out"=w1354:errorcluster, "timeTrial_count"=w1349:u32)
                      n878 = Multiply(x=w1348, y=1000.0) -> (x*y=w1352:dbl)
                      n879 = To Double Precision Float(number=w1349) -> (double precision float=w1351:dbl)
                      n880 = Divide(x=w1351, y=w1352) -> (x/y=w1353:dbl)
                      n881 = local write "FPGA_count2ms"(w1353) -> ()
                      n882 = xnode "Read/Write Control"("FPGA VI Reference In"=w1355, "error in"=w1354, "timeTrial_trig"=FALSE ("timeTrial")) -> ("error out"=w1347:errorcluster)  [unwired: 1 out]
                    }
                  }
                }
              }
              n883 = Select(t=myRIO_BRig_RT__Case_NonExp_stateList."Idle" ("Enum"), s=w1322, f=w1320) -> (s? t:f=w1319:T1)
              n884 = local write "error out"(w1318) -> ()
            }
            frame "End" {
            }
          }
          n885 = local read "MTrig_Audio_trig__R"() -> (w91:bool)
          n886 = local read "MTrig_Audio_trig__L"() -> (w92:bool)
          n887 = local read "MTrig_Laser_trig"() -> (w90:bool)
          n888 = local read "MTrig_CueLed"() -> (w83:bool)
          n889 = Compound Arithmetic op=OR(w92, w91, w90, w83) -> (w89:bool)
          n890 = local read "START"() -> (w115:bool)
          n891 = local read "STOP_abort"() -> (w114:bool)
          n892 = case shown="True" w89 {
            frame False {
            }
            frame True {
              w131 = FALSE
              n893 = local write "MTrig_Audio_trig__R"(w131) -> ()
              n894 = local write "MTrig_Audio_trig__L"(w131) -> ()
              n895 = local write "MTrig_Laser_trig"(w131) -> ()
              n896 = local write "MTrig_CueLed"(w131) -> ()
            }
          }
          n897 = call "myRIO_BRig_RT_dataMTrig_main__NoExp.vi"("input_dataMTrig"=w118, "input_Audio_trig_L"=w92, "input_Audio_trig_R"=w91, "input_Laser_trig"=w90, "input_CueLed"=w83) -> ("output_dataMTrig"=w117:u16[], "output_Audio_L"=w109:bool, "output_Audio_R"=w110:bool, "output_Laser"=w88:bool, "output_CueLed"=w82:bool)  [unwired: 10 in]
          n898 = Or(x=w115, y=w114) -> (x .or. y?=w113:bool)
          n899 = Select(t=myRIO_BRig_RT__Case_NonExp_stateList."End" ("Enum"), s=w113, f=w112) -> (s? t:f=w111:T1)
          n900 = Not(x="MTrig_Laser_Switch") -> (.not. x?=w85:bool)
          n901 = And(x=w88, y=w85) -> (x .and. y?=w86:bool)
          n902 = And(x=w88, y="MTrig_Laser_Switch") -> (x .and. y?=w87:bool)
          n903 = xnode "Read/Write Control"("FPGA VI Reference In"=w98, "error in"=w97, "A1_SR"=w119, "A3_SL"=w120, "audioTrigger_L"=w109, "audioTrigger_R"=w110, "LC_Laser_l1"=w86, "LC_Laser_l2"=w87, "CueLed_Event"=w82) -> ("FPGA VI Reference Out"=w125:refnum<k20>, "error out"=w124:errorcluster)
          n904 = node-c288() -> ()  [unwired: 1 in, 1 out]
          "cState_NonExp" <- w123
        }
        n905 = node-c288(w70) -> ()  [unwired: 1 out]
        n906 = flat-sequence {
          tunnel: w63 -> [w81]
          tunnel: [w81] -> w62
          tunnel: w61 -> [w80]
          tunnel: [w80] -> w60
          frame #0 {
            w79 = FALSE
            n907 = local write "STOP_endBlock"(w79) -> ()
            n908 = local write "STOP_endTrial"(w79) -> ()
          }
        }
      }
      frame True {
        w1371 = u16 0
        w1388 = u16 0 ("idxDataBlock")
        w1390 = u16 100 ("new element/subarray")
        w1391 = u16 100 ("new element/subarray")
        w1411 = T6 refnum items=["Session NI_WebDAV"] ("output_hSession")
        w1420 = FALSE
        # "dummyState counter"
        # "audio__L\naudio__R"
        # "Audio params"
        # "nRewards"
        # "idxDataBlock"
        # "Solenoid_Tdelay_R"
        # "Solenoid_Tdelay_L"
        # "RewCalib_N__R"
        # "RewCalib_N__L"
        # "Save dataLick to file\nSend file to Host\nSave dataMTrig\nSend file to Host\nDisconnect"
        # "dataTrial"
        # "dataTrial"
        # "Solenoid_Tcycle_R"
        # "Solenoid_Tcycle_L"
        # "Laser_Tcycle"
        # "Audio_Tcycle_R"
        # "Audio_Tcycle_L"
        # "dataLick"
        # "dataLC"
        # "dataLC"
        # "dataBlock"
        # "dataBlock"
        # "dataMTrig"
        # "dataMTrig"
        # "dataExp"
        # "dataCurrent"
        # "dataExp"
        # "dataCurrent"
        # "spout"
        # "state"
        n909 = call "myRIO_BRig_RT_dataMTrig_Solenoid_Tcycle__L.vi"() -> ("output_Solenoid_Tcycle__L"=w1417:i32)  [unwired: 11 in]
        n910 = call "myRIO_BRig_RT_dataMTrig_Solenoid_Tcycle__R.vi"() -> ("output_Solenoid_Tcycle__R"=w1416:i32)  [unwired: 11 in]
        n911 = call "myRIO_BRig_RT_dataMTrig_Audio_Tcycle__L.vi"() -> ("output_Audio_Tcycle__L"=w1415:i32)  [unwired: 11 in]
        n912 = call "myRIO_BRig_RT_dataMTrig_Audio_Tcycle__R.vi"() -> ("output_Audio_Tcycle__R"=w1414:i32)  [unwired: 11 in]
        n913 = call "myRIO_BRig_RT_dataMTrig_Laser_Tcycle.vi"() -> ("output_Laser_Tcycle"=w1413:i32)  [unwired: 11 in]
        n914 = local read "Tcycle_Reward_min_L"() -> (w1392:u16)
        n915 = local read "Tcycle_Reward_min_R"() -> (w1393:u16)
        n916 = local read "MTrig_Solenoid_Tcycle__L"() -> (w1396:u16)
        n917 = local read "MTrig_Solenoid_Tcycle__R"() -> (w1395:u16)
        n918 = local read "MTrig_Laser_Tcycle"() -> (w1394:u16)
        n919 = call "myRIO_BRig_RT_dataMTrig_Solenoid_RewCalib_nCycle__L.vi"() -> ("output_Solenoid_RewCalib_nCycle__L"=w1399:i32)  [unwired: 11 in]
        n920 = call "myRIO_BRig_RT_dataMTrig_Solenoid_Tdelay__L.vi"() -> ("output_Solenoid_Tdelay__L"=w1401:i32)  [unwired: 11 in]
        n921 = call "myRIO_BRig_RT_dataMTrig_Solenoid_RewCalib_nCycle__R.vi"() -> ("output_Solenoid_RewCalib_nCycle__R"=w1400:i32)  [unwired: 11 in]
        n922 = call "myRIO_BRig_RT_dataMTrig_Solenoid_Tdelay__R.vi"() -> ("output_Solenoid_Tdelay__R"=w1402:i32)  [unwired: 11 in]
        n923 = case shown="False" w1381 {
          selector: w1381 -> [_ w1442]
          tunnel: w1380 -> [w1439 w1444]
          tunnel: [w1440 w1444] -> w1376
          tunnel: w1379 -> [_ w1443]
          tunnel: [w1441 w1443] -> w1377
          tunnel: [w1438 w1442] -> w1375
          frame False {
            n924 = call "myRIO__TCP_connect_forWriting.vi"("input_error"=w1439) -> ("output_error"=w1440:errorcluster, "output_connected"=w1438:bool, "output_hTCP"=w1441:refnum<k5>)  [unwired: 8 in]
          }
          frame True {
          }
        }
        n925 = call "myRIO_BRig_RT_dataLick_init.vi"() -> ("output_dataLick"=w1422:u16[][])  [unwired: 11 in]
        n926 = call "myRIO_BRig_RT_dataCurrent_init.vi"() -> ("output_dataCurrent"=w1429:u16[])  [unwired: 11 in]
        n927 = call "myRIO_BRig_RT_dataExp_init.vi"() -> ("output_dataExp"=w1428:u16[])  [unwired: 11 in]
        n928 = call "myRIO_BRig_RT_dataMTrig_init.vi"() -> ("output_dataMTrig"=w1419:u16[])  [unwired: 5 in]
        n929 = call "myRIO_BRig_RT_dataLC_init.vi"() -> ("output_dataLC"=w1426:u16[])  [unwired: 11 in]
        n930 = call "myRIO_BRig_RT_dataBlock_init.vi"() -> ("output_dataBlock"=w1427:u16[][])  [unwired: 11 in]
        n931 = call "myRIO_BRig_RT_dataTrial_init.vi"() -> ("output_dataTrial"=w1412:u16[][])  [unwired: 11 in]
        n932 = local write "I_connect_TCP"(w1375) -> ()
        n933 = Replace Array Subset(array=w1419, new element #1=w1391, index #1=w1399, new element #2=w1391, index #2=w1400, new element #3=w1390, index #3=w1401, new element #4=w1390, index #4=w1402, new element #5=w1396, index #5=w1417, new element #6=w1395, index #6=w1416, new element #7=w1392, index #7=w1415, new element #8=w1393, index #8=w1414, new element #9=w1394, index #9=w1413) -> (w1418:u16[])
        n934 = call "myRIO_BRig_RT_dataAnalog_init.vi"() -> ("output_dataAnalog"=w1386:u16[][])  [unwired: 11 in]
        n935 = call "myRIO_BRig_RT_TCP__start_exp.vi"("input_hTCP"=w1377, "input_I_connected_TCP"=w1375, "input_error"=w1376) -> ("output_hTCP"=w1374:refnum<k5>, "output_error"=w1373:errorcluster)  [unwired: 11 in]
        n936 = Get Date/Time In Seconds() -> (seconds since 1Jan1904=w1398:timestamp)
        n937 = call "myRIO_BRig_RT_arrTrig_init.vi"() -> ("output_arrTrig"=w1370:bool[])  [unwired: 11 in]
        n938 = To Double Precision Float(number=w1398) -> (double precision float=w1397:dbl)
        n939 = node-c288() -> (w1437:T3)  [unwired: 4 in]
        n940 = timed-loop {
          timing: w1437 -> [_]
          timing-out: [_] -> w1436
          shift-right: [w1571] -> _
          shift-left: myRIO_BRig_RT__Case_Exp_stateList."Start1" ("Enum") -> [w1495]
          shift-right: [w1529] -> _
          shift-left: enum16{"Left", "Right"}."Left" -> [w1611]
          tunnel: w1369 -> [w1609]
          tunnel: w1368 -> [w1501]
          shift-right: [w1604] -> _
          shift-left: w1434 -> [w1608]
          shift-right: [w1603] -> _
          shift-left: w1433 -> [w1607]
          tunnel: [w1587] -> w1431
          tunnel: [w1588] -> w1432
          shift-right: [w1589] -> w1403
          shift-left: w1429 -> [w1490]
          shift-right: [w1602] -> _
          shift-left: w1428 -> [w1562]
          shift-right: [w1583] -> w1407
          shift-left: w1418 -> [w1584]
          shift-right: [w1600] -> _
          shift-left: w1427 -> [w1601]
          shift-right: [w1598] -> _
          shift-left: w1426 -> [w1599]
          shift-right: [w1590] -> w1409
          shift-left: w1422 -> [w1591]
          shift-right: [w1560] -> _
          shift-left: w1420 -> [w1585]
          shift-right: [w1561] -> _
          shift-left: w1420 -> [w1586]
          shift-right: [w1569] -> _
          shift-left: w1412 -> [w1570]
          shift-right: [w1568] -> w1405
          shift-left: w1411 -> [w1566]
          shift-right: [w1567] -> w1406
          shift-left: FALSE ("output_Iconnected") -> [w1565]
          tunnel: "Data Set Prefix" -> [w1564]
          tunnel: [w1564] -> w1404
          tunnel: w1397 -> [w1563]
          shift-right: [w1558] -> _
          shift-left: 0 ("idxDataBlock") -> [w1559]
          shift-right: [w1555] -> _
          shift-left: w1388 -> [w1557]
          shift-right: [w1554] -> _
          shift-left: w1388 -> [w1556]
          shift-right: [w1548] -> w1384
          shift-left: 0 -> [w1534]
          shift-right: [w1530] -> _
          shift-left: w1371 -> [w1543]
          shift-right: [w1531] -> _
          shift-left: w1371 -> [w1540]
          shift-right: [w1539] -> _
          shift-left: w1371 -> [w1546]
          shift-right: [w1549] -> w1385
          shift-left: w1386 -> [w1550]
          tunnel: w1374 -> [w1538]
          tunnel: [w1537] -> w1383
          tunnel: w1375 -> [w1535]
          tunnel: [w1535] -> w1382
          tunnel: w1373 -> [w1536]
          tunnel: [w1498] -> w1378
          shift-right: [w1527] -> _
          shift-left: u16 0 -> [w1528]
          shift-right: [w1525] -> _
          shift-left: w1371 -> [w1526]
          shift-right: [w1522] -> _
          shift-left: w1370 -> [w1523]
          shift-right: [w1493] -> _
          shift-left: FALSE -> [w1496]
          stop <- w1597 stop-if-true
          # "arrTrig"
          # "arrTrig"
          # "LC_Laser_l2"
          # "LC_Event_l2"
          # "LC_Laser_l1"
          # "LC_Event_l1"
          # "CueLed"
          # "LC_Laser_l2"
          # "LC_Event_l2"
          # "LC_Laser_l1"
          # "LC_Event_l1"
          # "solenoid__R"
          # "solenoid__L"
          # "spout"
          # "iState"
          # "dataAnalog"
          # "index"
          # "iEvent"
          # "iBlock"
          # "iTrial"
          # "Laser"
          # "Audio R"
          # "Audio L"
          # "Solenoid R"
          # "Solenoid L"
          # "manual triggering"
          # "dataTrial"
          # "dataBlock"
          # "nRewards"
          # "dataExp"
          # "dataCurrent"
          # "audio__L\naudio__R"
          # "time stamp"
          # "nRewards"
          # "idxDataBlock"
          # "idxDataBlock"
          # "audio__L\naudio__R"
          # "dataLC"
          # "solenoid__R"
          # "solenoid__L"
          # "Did a lick occur?"
          # "Update lick counter"
          # "spout"
          # "spout"
          # "state"
          # "state"
          n941 = node-c288() -> ()  [unwired: 1 in, 1 out]
          n942 = flat-sequence {
            tunnel: w1501 -> [w1612]
            tunnel: [w1612] -> _
            tunnel: [w1613] -> w1497
            tunnel: [w1612] -> w1500
            frame #0 {
              n943 = Get Date/Time In Seconds() -> (seconds since 1Jan1904=w1613:timestamp)
            }
          }
          n944 = xnode "Read/Write Control"("FPGA VI Reference In"=w1609, "error in"=w1500) -> ("FPGA VI Reference Out"=w1553:refnum<k20>, "error out"=w1552:errorcluster, "A2_LickL"=w1604:u32, "A4_LickR"=w1603:u32)
          "A2" <- w1604
          "A4" <- w1603
          n945 = Greater?(x=w1604, y=w1608) -> (0:w1606:bool)
          n946 = Greater?(x=w1603, y=w1607) -> (0:w1605:bool)
          n947 = call "myRIO_BRig_RT_dataCurrent_IallReward_L.vi"() -> ("output_IallReward_L"=w1491:i32)  [unwired: 11 in]
          n948 = call "myRIO_BRig_RT_dataCurrent_IallReward_R.vi"() -> ("output_IallReward_R"=w1492:i32)  [unwired: 11 in]
          n949 = Or(x=w1606, y=w1605) -> (x .or. y?=w1610:bool)
          n950 = local read "MTrig_Solenoid_trig__L"() -> (w1581:bool)
          n951 = local read "MTrig_Solenoid_trig__R"() -> (w1580:bool)
          n952 = local read "MTrig_Audio_trig__L"() -> (w1579:bool)
          n953 = local read "MTrig_Audio_trig__R"() -> (w1578:bool)
          n954 = local read "MTrig_Laser_trig"() -> (w1577:bool)
          n955 = Index Array(array=w1490, index #1=w1491, index #2=w1492) -> (element #1=w1488:u16, element #2=w1489:u16)
          n956 = Not Equal To 0?(x=w1488) -> (x != 0?=→"allReward_L":bool)
          n957 = Not Equal To 0?(x=w1489) -> (x != 0?=→"allReward_R":bool)
          n958 = case shown="\"Start1\", Default" w1495 {
            selector: w1495 -> [_ _ _ _ _ _ _ _ _ _ _ _ _ _ _ _ _ _ _ _ _ _ _ _ _ w2578 _ w2621 _ _ _ _ _ w2718 _ w2778 _ _ _ _ _ w2881 _ w2933 _ w2988 _ w3028 _ _ w3086 _ _ _ _ _ w3233 _ _ _ _ _ _ _ _ _ _ _ _ w3466 w3495]
            tunnel: [myRIO_BRig_RT__Case_Exp_stateList."Start2" ("Enum") myRIO_BRig_RT__Case_Exp_stateList."Start3" ("Enum") myRIO_BRig_RT__Case_Exp_stateList."saveSettings1" ("Enum") myRIO_BRig_RT__Case_Exp_stateList."saveSettings2" ("Enum") myRIO_BRig_RT__Case_Exp_stateList."saveSettings3" ("Enum") myRIO_BRig_RT__Case_Exp_stateList."saveSettings4" ("Enum") myRIO_BRig_RT__Case_Exp_stateList."saveSettings_LC_ENL_l1" ("Enum") myRIO_BRig_RT__Case_Exp_stateList."saveSettings_LC_ENL_l2" ("Enum") myRIO_BRig_RT__Case_Exp_stateList."saveSettings_LC_Cue_l1" ("Enum") myRIO_BRig_RT__Case_Exp_stateList."saveSettings_LC_Cue_l2" ("Enum") myRIO_BRig_RT__Case_Exp_stateList."saveSettings6_LC_l1_Other" ("Enum") myRIO_BRig_RT__Case_Exp_stateList."SaveSettings6_LC_l2_Other" ("Enum") myRIO_BRig_RT__Case_Exp_stateList."setSettings_Audio" ("Enum") myRIO_BRig_RT__Case_Exp_stateList."setSettings_Laser" ("Enum") myRIO_BRig_RT__Case_Exp_stateList."commConnect" ("Enum") w2335 myRIO_BRig_RT__Case_Exp_stateList."initTrial" ("Enum") w2389 myRIO_BRig_RT__Case_Exp_stateList."initTrial3" ("Enum") myRIO_BRig_RT__Case_Exp_stateList."initTrial_LC_ENL1" ("Enum") myRIO_BRig_RT__Case_Exp_stateList."ENL1_pre" ("Enum") myRIO_BRig_RT__Case_Exp_stateList."initTrial_LC_Cue1" ("Enum") myRIO_BRig_RT__Case_Exp_stateList."initTrial_LC_Sel" ("Enum") myRIO_BRig_RT__Case_Exp_stateList."initTrial4" ("Enum") w2553 w2575 myRIO_BRig_RT__Case_Exp_stateList."ENL1Penalty" ("Enum") w2622 myRIO_BRig_RT__Case_Exp_stateList."endExp" ("Enum") myRIO_BRig_RT__Case_Exp_stateList."endExp" ("Enum") myRIO_BRig_RT__Case_Exp_stateList."endExp" ("Enum") myRIO_BRig_RT__Case_Exp_stateList."endExp" ("Enum") w2695 w2712 myRIO_BRig_RT__Case_Exp_stateList."Cue1Penalty" ("Enum") w2776 myRIO_BRig_RT__Case_Exp_stateList."endExp" ("Enum") myRIO_BRig_RT__Case_Exp_stateList."endExp" ("Enum") myRIO_BRig_RT__Case_Exp_stateList."endExp" ("Enum") myRIO_BRig_RT__Case_Exp_stateList."endExp" ("Enum") w2854 w2880 myRIO_BRig_RT__Case_Exp_stateList."SelectReward" ("Enum") w2934 myRIO_BRig_RT__Case_Exp_stateList."SelectRewardPost" ("Enum") w2989 myRIO_BRig_RT__Case_Exp_stateList."SelectWrong" ("Enum") w3024 myRIO_BRig_RT__Case_Exp_stateList."endTrial1" ("Enum") myRIO_BRig_RT__Case_Exp_stateList."SelectTimeout" ("Enum") w3088 myRIO_BRig_RT__Case_Exp_stateList."endTrial1" ("Enum") myRIO_BRig_RT__Case_Exp_stateList."endTrial2" ("Enum") myRIO_BRig_RT__Case_Exp_stateList."endTrial3" ("Enum") w3158 w3216 w3233 myRIO_BRig_RT__Case_Exp_stateList."initBlock" ("Enum") w3256 myRIO_BRig_RT__Case_Exp_stateList."commUpload_dataExp" ("Enum") myRIO_BRig_RT__Case_Exp_stateList."endBlock" ("Enum") myRIO_BRig_RT__Case_Exp_stateList."commUpload_dataLC" ("Enum") myRIO_BRig_RT__Case_Exp_stateList."commUpload_dataTrial" ("Enum") myRIO_BRig_RT__Case_Exp_stateList."commUpload_dataCurrent" ("Enum") myRIO_BRig_RT__Case_Exp_stateList."saveData_dataCurrent" ("Enum") myRIO_BRig_RT__Case_Exp_stateList."saveData_dataExp" ("Enum") myRIO_BRig_RT__Case_Exp_stateList."saveData_dataLC" ("Enum") myRIO_BRig_RT__Case_Exp_stateList."saveData_dataTrial" ("Enum") myRIO_BRig_RT__Case_Exp_stateList."commUpload_pre" ("Enum") w3465 w3494] -> w1571
            tunnel: [w1640 w1655 w1673 w1736 w1794 w1856 w1915 w1975 w2035 w2095 w2155 w2194 w2234 w2263 w2326 w2334 w2359 w2376 w2406 w2448 w2476 w2497 w2516 w2539 w2563 w2587 w2608 w2626 w2638 w2656 w2671 w2686 w2694 w2734 w2758 w2775 w2792 w2809 w2824 w2839 w2863 w2895 w2916 w2931 w2944 w2986 w3006 w3034 w3051 w3067 w3094 w3113 w3125 w3141 w3178 w3193 w3232 w3245 w3259 w3285 w3302 w3319 w3336 w3353 w3377 w3393 w3416 w3432 w3452 w3482 w3511] -> w1529
            tunnel: w1611 -> [w1640 w1655 w1673 w1736 w1794 w1856 w1915 w1975 w2035 w2095 w2155 w2194 w2234 w2263 w2326 w2336 w2359 w2376 w2406 w2448 w2476 w2497 w2516 w2539 w2563 w2587 w2608 w2626 w2638 w2656 w2671 w2686 w2694 w2734 w2758 w2775 w2792 w2809 w2824 w2839 w2863 w2895 w2916 w2931 w2944 w2986 w3006 w3034 w3051 w3067 w3094 w3113 w3125 w3141 w3178 w3193 w3232 w3245 w3259 w3285 w3302 w3319 w3336 w3353 w3377 w3393 w3416 w3432 w3452 w3482 w3511]
            tunnel: w1610 -> [w1643 w1658 w1670 w1739 w1797 w1859 w1918 w1978 w2038 w2098 w2158 w2197 w2237 w2266 w2329 w2351 w2366 w2390 w2425 w2459 w2486 w2505 w2525 w2548 w2554 w2574 w2611 w2629 w2644 w2659 w2674 w2689 w2698 w2717 w2764 w2782 w2797 w2812 w2827 w2842 w2862 w2894 w2921 w2940 w2971 w2994 w3017 w3037 w3050 w3079 w3099 w3110 w3129 w3140 w3185 w3215 w3236 w3242 w3264 w3288 w3305 w3322 w3339 w3356 w3380 w3396 w3419 w3435 w3455 w3485 w3514]
            tunnel: w1606 -> [w1642 w1657 w1671 w1738 w1796 w1858 w1917 w1977 w2037 w2097 w2157 w2196 w2236 w2265 w2328 w2350 w2365 w2391 w2424 w2460 w2487 w2506 w2526 w2549 w2567 w2589 w2610 w2628 w2643 w2658 w2673 w2688 w2708 w2735 w2763 w2781 w2796 w2811 w2826 w2841 w2844 w2870 w2920 w2939 w2970 w2993 w3016 w3036 w3049 w3078 w3098 w3111 w3130 w3139 w3184 w3214 w3235 w3243 w3265 w3287 w3304 w3321 w3338 w3355 w3379 w3395 w3418 w3434 w3454 w3484 w3513]
            tunnel: w1605 -> [w1641 w1656 w1672 w1737 w1795 w1857 w1916 w1976 w2036 w2096 w2156 w2195 w2235 w2264 w2327 w2349 w2364 w2392 w2423 w2461 w2488 w2507 w2527 w2550 w2566 w2588 w2609 w2627 w2642 w2657 w2672 w2687 w2707 w2736 w2762 w2780 w2795 w2810 w2825 w2840 w2843 w2869 w2919 w2938 w2969 w2992 w3015 w3035 w3048 w3077 w3097 w3112 w3131 w3138 w3183 w3213 w3234 w3244 w3266 w3286 w3303 w3320 w3337 w3354 w3378 w3394 w3417 w3433 w3453 w3483 w3512]
            tunnel: [w1643 w1658 w1670 w1739 w1797 w1859 w1918 w1978 w2038 w2098 w2158 w2197 w2237 w2266 w2329 w2351 w2366 w2390 w2425 w2459 w2486 w2505 w2525 w2548 w2554 w2574 w2611 w2629 w2644 w2659 w2674 w2689 w2698 w2717 w2764 w2782 w2797 w2812 w2827 w2842 w2862 w2894 w2921 w2940 w2971 w2994 w3017 w3037 w3050 w3079 w3099 w3110 w3129 w3140 w3185 w3215 w3236 w3242 w3264 w3288 w3305 w3322 w3339 w3356 w3380 w3396 w3419 w3435 w3455 w3485 w3514] -> w1594
            tunnel: [w1642 w1657 w1671 w1738 w1796 w1858 w1917 w1977 w2037 w2097 w2157 w2196 w2236 w2265 w2328 w2350 w2365 w2391 w2424 w2460 w2487 w2506 w2526 w2549 w2567 w2589 w2610 w2628 w2643 w2658 w2673 w2688 w2708 w2735 w2763 w2781 w2796 w2811 w2826 w2841 w2844 w2870 w2920 w2939 w2970 w2993 w3016 w3036 w3049 w3078 w3098 w3111 w3130 w3139 w3184 w3214 w3235 w3243 w3265 w3287 w3304 w3321 w3338 w3355 w3379 w3395 w3418 w3434 w3454 w3484 w3513] -> w1593
            tunnel: [w1641 w1656 w1672 w1737 w1795 w1857 w1916 w1976 w2036 w2096 w2156 w2195 w2235 w2264 w2327 w2349 w2364 w2392 w2423 w2461 w2488 w2507 w2527 w2550 w2566 w2588 w2609 w2627 w2642 w2657 w2672 w2687 w2707 w2736 w2762 w2780 w2795 w2810 w2825 w2840 w2843 w2869 w2919 w2938 w2969 w2992 w3015 w3035 w3048 w3077 w3097 w3112 w3131 w3138 w3183 w3213 w3234 w3244 w3266 w3286 w3303 w3320 w3337 w3354 w3378 w3394 w3417 w3433 w3453 w3483 w3512] -> w1592
            tunnel: w1490 -> [w1639 w1654 w1669 w1703 w1779 w1798 w1860 w1974 w2034 w2094 w2154 w2193 w2233 w2261 w2280 w2342 w2358 w2388 w2395 w2437 w2475 w2496 w2515 w2538 w2555 w2577 w2602 w2625 w2639 w2655 w2670 w2685 w2697 w2719 w2757 w2779 w2793 w2808 w2823 w2838 w2856 w2883 w2896 w2936 w2946 w2991 w3007 w3033 w3047 w3068 w3096 w3109 w3122 w3143 w3160 w3191 w3231 w3246 w3267 w3282 w3299 w3316 w3333 w3344 w3370 w3385 w3405 w3429 w3445 w3464 w3493]
            tunnel: w1562 -> [w1638 w1653 w1668 w1734 w1792 w1853 w1912 w1972 w2032 w2092 w2152 w2191 w2231 w2254 w2272 w2339 w2363 w2387 w2393 w2432 w2478 w2489 w2519 w2542 w2565 w2586 w2601 w2623 w2641 w2654 w2669 w2684 w2693 w2733 w2755 w2774 w2794 w2807 w2822 w2837 w2846 w2871 w2917 w2923 w2963 w2987 w3008 w3031 w3046 w3070 w3093 w3108 w3128 w3132 w3159 w3206 w3230 w3247 w3268 w3281 w3298 w3315 w3332 w3345 w3374 w3390 w3401 w3428 w3449 w3479 w3508]
            tunnel: [w1639 w1654 w1669 w1703 w1779 w1798 w1860 w1974 w2034 w2094 w2154 w2193 w2233 w2261 w2279 w2341 w2358 w2381 w2394 w2436 w2475 w2495 w2514 w2537 w2552 w2576 w2603 w2624 w2639 w2655 w2670 w2685 w2696 w2713 w2756 w2777 w2793 w2808 w2823 w2838 w2855 w2882 w2918 w2935 w2964 w2990 w3009 w3032 w3047 w3071 w3095 w3109 w3121 w3142 w3160 w3189 w3231 w3246 w3267 w3282 w3299 w3316 w3333 w3344 w3370 w3385 w3405 w3429 w3445 w3464 w3493] -> w1503
            tunnel: [w1638 w1653 w1668 w1733 w1791 w1848 w1911 w1972 w2032 w2092 w2152 w2191 w2231 w2254 w2271 w2340 w2363 w2386 w2393 w2432 w2478 w2489 w2519 w2542 w2565 w2586 w2601 w2623 w2641 w2654 w2669 w2684 w2693 w2733 w2755 w2774 w2794 w2807 w2822 w2837 w2846 w2871 w2917 w2923 w2963 w2987 w3008 w3031 w3046 w3070 w3093 w3108 w3128 w3132 w3159 w3206 w3230 w3247 w3268 w3281 w3298 w3315 w3332 w3345 w3374 w3390 w3404 w3428 w3449 w3479 w3508] -> w1602
            tunnel: [_ _ _ _ _ _ _ _ _ _ _ _ _ _ _ _ _ _ _ _ _ _ _ _ _ _ _ _ _ _ _ _ _ _ _ _ _ _ _ _ _ _ _ w2929 _ _ _ _ _ _ _ _ _ _ _ _ _ _ _ _ _ _ _ _ _ _ _ _ _ _ _] -> w1520
            tunnel: [_ _ _ _ _ _ _ _ _ _ _ _ _ _ _ _ _ _ _ _ _ _ _ _ _ _ _ _ _ _ _ _ _ _ _ _ _ _ _ _ _ _ _ w2930 _ _ _ _ _ _ _ _ _ _ _ _ _ _ _ _ _ _ _ _ _ _ _ _ _ _ _] -> w1574
            tunnel: w1601 -> [w1636 w1651 w1666 w1705 w1781 w1854 w1913 w1973 w2033 w2093 w2153 w2192 w2232 w2259 w2323 w2331 w2360 w2371 w2416 w2457 w2484 w2492 w2511 w2534 w2564 w2585 w2598 w2619 w2640 w2652 w2667 w2682 w2706 w2732 w2754 w2772 w2790 w2805 w2820 w2835 w2868 w2892 w2914 w2937 w2948 w2984 w3005 w3029 w3044 w3069 w3092 w3106 w3124 w3147 w3181 w3202 w3228 w3249 w3270 w3279 w3296 w3313 w3330 w3350 w3364 w3387 w3411 w3426 w3447 w3477 w3506]
            tunnel: [w1636 w1651 w1666 w1705 w1781 w1854 w1913 w1973 w2033 w2093 w2153 w2192 w2232 w2259 w2323 w2330 w2357 w2371 w2416 w2457 w2484 w2492 w2511 w2534 w2564 w2585 w2598 w2619 w2640 w2652 w2667 w2682 w2706 w2732 w2754 w2772 w2790 w2805 w2820 w2835 w2868 w2892 w2914 w2937 w2947 w2984 w3005 w3029 w3044 w3069 w3092 w3106 w3123 w3147 w3181 w3202 w3228 w3249 w3270 w3279 w3296 w3313 w3330 w3350 w3364 w3387 w3411 w3426 w3447 w3477 w3506] -> w1600
            tunnel: w1599 -> [w1637 w1652 w1667 w1704 w1780 w1855 w1914 w1970 w2030 w2090 w2150 w2189 w2229 w2260 w2324 w2352 w2362 w2385 w2405 w2458 w2485 w2498 w2517 w2540 w2562 w2573 w2599 w2620 w2637 w2653 w2668 w2683 w2705 w2721 w2753 w2773 w2791 w2806 w2821 w2836 w2867 w2893 w2915 w2932 w2961 w2985 w3004 w3030 w3045 w3066 w3091 w3107 w3127 w3146 w3182 w3205 w3229 w3248 w3269 w3280 w3297 w3314 w3331 w3351 w3373 w3389 w3413 w3424 w3448 w3478 w3507]
            tunnel: [w1637 w1652 w1667 w1704 w1780 w1855 w1914 w1971 w2031 w2091 w2151 w2190 w2230 w2260 w2324 w2352 w2362 w2385 w2405 w2458 w2485 w2498 w2517 w2540 w2562 w2573 w2599 w2620 w2637 w2653 w2668 w2683 w2705 w2721 w2753 w2773 w2791 w2806 w2821 w2836 w2867 w2893 w2915 w2932 w2961 w2985 w3004 w3030 w3045 w3066 w3091 w3107 w3127 w3146 w3182 w3205 w3229 w3248 w3269 w3280 w3297 w3314 w3331 w3351 w3373 w3389 w3413 w3424 w3448 w3478 w3507] -> w1598
            tunnel: [_ _ _ _ _ _ _ _ _ _ _ _ _ _ _ _ _ _ _ _ _ _ _ _ _ _ _ _ _ _ _ _ _ _ _ _ _ _ _ _ _ _ _ _ _ _ _ _ _ _ _ _ _ _ _ _ TRUE _ _ _ _ _ _ _ _ _ _ _ _ _ _] -> w1595
            tunnel: w1586 -> [_ _ _ _ _ _ _ _ _ _ _ _ _ _ _ _ _ _ _ _ _ _ _ _ _ _ _ _ _ _ _ _ _ w2731 _ _ _ _ _ _ _ _ _ _ _ _ _ _ _ _ _ _ _ _ _ _ _ _ _ _ _ _ _ _ _ _ _ _ _ _ _]
            tunnel: w1585 -> [_ _ _ _ _ _ _ _ _ _ _ _ _ _ _ _ _ _ _ _ _ _ _ _ _ _ _ _ _ _ _ _ _ w2730 _ _ _ _ _ _ _ _ _ _ _ _ _ _ _ _ _ _ _ _ _ _ _ _ _ _ _ _ _ _ _ _ _ _ _ _ _]
            tunnel: [_ _ _ _ _ _ _ _ _ _ _ _ _ _ _ _ _ _ _ _ _ _ _ _ _ _ _ _ _ _ _ _ w2692 w2731 _ _ _ _ _ _ _ _ _ _ _ _ _ _ _ _ _ _ _ _ _ _ _ _ _ _ _ _ _ _ _ _ _ _ _ _ _] -> w1561
            tunnel: [_ _ _ _ _ _ _ _ _ _ _ _ _ _ _ _ _ _ _ _ _ _ _ _ _ _ _ _ _ _ _ _ w2691 w2730 _ _ _ _ _ _ _ _ _ _ _ _ _ _ _ _ _ _ _ _ _ _ _ _ _ _ _ _ _ _ _ _ _ _ _ _ _] -> w1560
            tunnel: w1570 -> [w1634 w1649 w1664 w1695 w1777 w1843 w1910 w1957 w2022 w2077 w2137 w2164 w2214 w2253 w2322 w2348 w2361 w2384 w2408 w2450 w2474 w2494 w2513 w2536 w2561 w2584 w2596 w2618 w2635 w2650 w2665 w2680 w2704 w2729 w2751 w2771 w2788 w2803 w2818 w2833 w2866 w2891 w2904 w2922 w2959 w2983 w3000 w3023 w3043 w3062 w3085 w3105 w3120 w3145 w3174 w3201 w3226 w3250 w3271 w3278 w3295 w3312 w3329 w3349 w3372 w3388 w3412 w3427 w3442 w3476 w3505]
            tunnel: [w1634 w1649 w1664 w1695 w1777 w1843 w1910 w1957 w2022 w2077 w2137 w2164 w2214 w2253 w2322 w2348 w2361 w2384 w2407 w2449 w2467 w2493 w2512 w2535 w2561 w2584 w2596 w2618 w2635 w2650 w2665 w2680 w2704 w2729 w2751 w2771 w2788 w2803 w2818 w2833 w2866 w2891 w2904 w2922 w2959 w2983 w3000 w3023 w3043 w3062 w3085 w3105 w3120 w3144 w3174 w3201 w3226 w3250 w3271 w3278 w3295 w3312 w3329 w3349 w3372 w3388 w3412 w3427 w3442 w3476 w3505] -> w1569
            tunnel: [w1633 w1648 w1663 w1694 w1776 w1842 w1909 w1956 w2021 w2076 w2136 w2163 w2213 w2252 w2321 w2347 w2368 w2383 w2418 w2456 w2483 w2504 w2524 w2547 w2560 w2583 w2595 w2617 w2634 w2649 w2664 w2679 w2703 w2728 w2750 w2770 w2787 w2802 w2817 w2832 w2865 w2890 w2903 w2928 w2958 w2982 w2999 w3022 w3042 w3061 w3084 w3104 w3119 w3137 w3180 w3200 w3224 w3251 w3261 w3277 w3294 w3311 w3328 w3348 w3376 w3392 w3415 w3431 w3451 w3481 w3510] -> w1568
            tunnel: [w1632 w1647 w1662 w1693 w1775 w1841 w1908 w1955 w2020 w2075 w2135 w2162 w2212 w2251 w2320 w2346 w2367 w2382 w2417 w2455 w2482 w2503 w2523 w2546 w2559 w2582 w2594 w2616 w2633 w2648 w2663 w2678 w2702 w2727 w2749 w2769 w2786 w2801 w2816 w2831 w2864 w2889 w2902 w2927 w2957 w2981 w2998 w3021 w3041 w3060 w3083 w3103 w3118 w3136 w3179 w3199 w3225 w3237 w3258 w3283 w3300 w3317 w3334 w3352 w3375 w3391 w3414 w3430 w3450 w3480 w3509] -> w1567
            tunnel: w1566 -> [w1633 w1648 w1663 w1694 w1776 w1842 w1909 w1956 w2021 w2076 w2136 w2163 w2213 w2252 w2321 w2347 w2368 w2383 w2418 w2456 w2483 w2504 w2524 w2547 w2560 w2583 w2595 w2617 w2634 w2649 w2664 w2679 w2703 w2728 w2750 w2770 w2787 w2802 w2817 w2832 w2865 w2890 w2903 w2928 w2958 w2982 w2999 w3022 w3042 w3061 w3084 w3104 w3119 w3137 w3180 w3200 w3224 _ w3261 w3277 w3294 w3311 w3328 w3348 w3376 w3392 w3415 w3431 w3451 w3481 w3510]
            tunnel: w1565 -> [w1632 w1647 w1662 w1693 w1775 w1841 w1908 w1955 w2020 w2075 w2135 w2162 w2212 w2251 w2320 w2346 w2367 w2382 w2417 w2455 w2482 w2503 w2523 w2546 w2559 w2582 w2594 w2616 w2633 w2648 w2663 w2678 w2702 w2727 w2749 w2769 w2786 w2801 w2816 w2831 w2864 w2889 w2902 w2927 w2957 w2981 w2998 w3021 w3041 w3060 w3083 w3103 w3118 w3136 w3179 w3199 w3225 _ w3258 w3283 w3300 w3317 w3334 w3352 w3375 w3391 w3414 w3430 w3450 w3480 w3509]
            tunnel: w1564 -> [_ _ _ _ _ _ _ _ _ _ _ _ _ _ _ _ _ _ _ _ _ _ _ _ _ _ _ _ _ _ _ _ _ _ _ _ _ _ _ _ _ _ _ _ _ _ _ _ _ _ _ _ _ _ _ _ _ _ _ w3275 w3292 w3309 w3326 w3346 _ _ _ _ _ _ _]
            tunnel: w1563 -> [_ _ _ _ _ _ _ _ _ _ _ _ _ _ _ _ _ _ _ _ _ _ _ _ _ _ _ _ _ _ _ _ _ _ _ _ _ _ _ _ _ _ _ _ _ _ _ _ _ _ _ _ _ _ _ _ _ _ _ _ _ _ _ _ _ _ w3406 _ _ _ _]
            tunnel: [w1631 w1646 w1661 w1692 w1774 w1840 w1907 w1954 w2019 w2074 w2134 w2161 w2211 w2250 w2319 w2337 w2355 w2380 w2419 w2454 w2481 w2502 w2522 w2545 w2558 w2581 w2593 w2615 w2632 w2647 w2662 w2677 w2701 w2726 w2748 w2768 w2785 w2800 w2815 w2830 w2861 w2888 w2901 w2926 w2942 w2980 w2997 w3020 w3040 w3059 w3082 w3102 w3117 w3135 w3177 w3186 w3223 w3240 w3260 w3274 w3291 w3308 w3325 w3343 w3359 w3384 w3400 w3423 w3440 w3475 w3504] -> w1558
            tunnel: w1559 -> [w1631 w1646 w1661 w1692 w1774 w1840 w1907 w1954 w2019 w2074 w2134 w2161 w2211 w2250 w2319 _ _ w2380 w2419 w2454 w2481 w2502 w2522 w2545 w2558 w2581 w2593 w2615 w2632 w2647 w2662 w2677 w2701 w2726 w2748 w2768 w2785 w2800 w2815 w2830 w2861 w2888 w2901 w2926 w2942 w2980 w2997 w3020 w3040 w3059 w3082 w3102 w3117 w3135 w3177 w3187 w3223 w3240 w3260 w3274 w3291 w3308 w3325 w3343 w3359 w3384 w3400 w3423 w3440 w3475 w3504]
            tunnel: w1557 -> [w1630 w1645 w1660 w1691 w1773 w1839 w1906 w1953 w2018 w2073 w2133 w2160 w2210 w2249 w2318 w2345 w2354 w2379 w2415 w2453 w2480 w2501 w2521 w2544 w2557 w2580 w2592 w2614 w2631 w2646 w2661 w2676 w2700 w2725 w2747 w2767 w2784 w2799 w2814 w2829 w2860 w2887 w2900 w2925 w2956 w2979 w2996 w3019 w3039 w3058 w3081 w3101 w3116 w3134 w3176 w3198 w3222 w3239 w3263 w3273 w3290 w3307 w3324 w3342 w3358 w3383 w3399 w3422 w3439 w3474 w3503]
            tunnel: w1556 -> [w1629 w1644 w1659 w1690 w1772 w1838 w1905 w1952 w2017 w2072 w2132 w2159 w2209 w2248 w2317 w2344 w2353 w2378 w2414 w2452 w2479 w2500 w2520 w2543 w2556 w2579 w2591 w2613 w2630 w2645 w2660 w2675 w2699 w2724 w2746 w2766 w2783 w2798 w2813 w2828 w2859 w2886 w2899 w2924 w2953 w2978 w2995 w3018 w3038 w3057 w3080 w3100 w3115 w3133 w3175 w3197 w3221 w3238 w3262 w3272 w3289 w3306 w3323 w3341 w3357 w3382 w3398 w3421 w3438 w3473 w3502]
            tunnel: [w1630 w1645 w1660 w1691 w1773 w1839 w1906 w1953 w2018 w2073 w2133 w2160 w2210 w2249 w2318 w2345 w2354 w2379 w2415 w2453 w2480 w2501 w2521 w2544 w2557 w2580 w2592 w2614 w2631 w2646 w2661 w2676 w2700 w2725 w2747 w2767 w2784 w2799 w2814 w2829 w2860 w2887 w2900 w2925 w2955 w2979 w2996 w3019 w3039 w3058 w3081 w3101 w3116 w3134 w3176 w3198 w3222 w3239 w3263 w3273 w3290 w3307 w3324 w3342 w3358 w3383 w3399 w3422 w3439 w3474 w3503] -> w1555
            tunnel: [w1629 w1644 w1659 w1690 w1772 w1838 w1905 w1952 w2017 w2072 w2132 w2159 w2209 w2248 w2317 w2344 w2353 w2378 w2414 w2452 w2479 w2500 w2520 w2543 w2556 w2579 w2591 w2613 w2630 w2645 w2660 w2675 w2699 w2724 w2746 w2766 w2783 w2798 w2813 w2828 w2859 w2886 w2899 w2924 w2954 w2978 w2995 w3018 w3038 w3057 w3080 w3100 w3115 w3133 w3175 w3197 w3221 w3238 w3262 w3272 w3289 w3306 w3323 w3341 w3357 w3382 w3398 w3421 w3438 w3473 w3502] -> w1554
            tunnel: w1553 -> [w1628 _ _ _ _ _ _ _ _ _ _ _ _ w2245 w2314 _ _ w2375 w2422 w2444 w2465 _ _ w2530 _ _ _ _ _ _ _ _ _ w2723 _ _ _ _ _ _ w2857 w2885 _ _ _ _ _ _ _ w3056 _ _ _ _ w3156 _ w3219 _ _ _ _ _ _ _ _ _ _ _ _ _ _]
            tunnel: w1552 -> [w1627 _ _ _ _ _ _ _ _ _ _ _ _ w2244 w2315 _ _ w2374 w2421 w2443 w2464 _ _ w2529 _ _ _ _ _ _ _ _ _ w2722 _ _ _ _ _ _ w2858 w2884 _ _ _ _ _ _ _ w3055 _ _ _ _ w3155 _ w3218 _ _ _ _ _ _ _ _ _ _ _ _ _ _]
            tunnel: [_ _ _ _ _ _ _ _ _ _ _ _ _ _ _ _ _ _ _ _ _ _ _ _ _ w2571 _ _ _ _ _ _ _ w2709 _ _ _ _ _ _ w2850 w2876 _ _ _ _ _ _ _ _ _ _ _ _ _ _ _ _ _ _ _ _ _ _ _ _ _ _ _ _ _] -> w1511
            tunnel: [_ _ _ _ _ _ _ _ _ _ _ _ _ _ _ _ _ _ _ _ _ _ _ _ _ w2570 _ _ _ _ _ _ _ w2710 _ _ _ _ _ _ w2849 w2875 _ _ _ _ _ _ _ _ _ _ _ _ _ _ _ _ _ _ _ _ _ _ _ _ _ _ _ _ _] -> w1510
            tunnel: [_ _ _ _ _ _ _ _ _ _ _ _ _ _ _ _ _ _ _ _ _ _ TRUE ("Recording") _ _ _ _ _ _ _ _ _ _ _ _ _ _ _ _ _ _ _ _ _ _ _ _ _ _ _ _ _ _ _ _ _ _ _ _ _ _ _ _ _ _ _ _ _ _ _ _] -> w1547
            tunnel: [_ _ _ _ _ _ _ _ _ _ _ _ _ _ _ TRUE _ _ _ _ _ _ _ _ _ _ _ _ _ _ _ _ _ _ _ _ _ _ _ _ _ _ _ _ _ _ _ _ _ _ _ _ _ _ _ _ _ _ _ _ _ _ _ _ _ _ _ _ _ _ _] -> w1544
            tunnel: [_ _ _ _ _ _ _ _ _ _ _ _ _ _ _ _ _ TRUE _ _ _ _ _ _ _ _ _ _ _ _ _ _ _ _ _ _ _ _ _ _ _ _ _ _ _ _ _ _ _ _ _ _ _ _ _ _ _ _ _ _ _ _ _ _ _ _ _ _ _ _ _] -> w1542
            tunnel: [_ _ _ _ _ _ _ _ _ _ _ _ _ _ _ _ _ w2370 _ _ _ _ _ _ _ _ _ _ _ _ _ _ _ _ _ _ _ _ _ _ _ _ _ _ _ _ _ _ _ _ _ _ _ _ _ _ _ _ _ _ _ _ _ _ _ _ _ _ _ _ _] -> w1541
            tunnel: w1528 -> [_ _ _ _ _ _ _ _ _ _ _ _ _ _ _ _ _ _ _ _ _ _ _ _ _ _ _ _ _ _ _ _ _ _ _ _ _ _ _ _ _ _ _ _ _ _ _ _ _ _ _ _ _ _ _ _ _ _ _ _ _ _ _ _ _ _ _ _ _ w3471 w3500]
            tunnel: [_ _ _ _ _ _ _ _ _ _ _ _ _ _ _ _ _ _ _ _ _ _ _ _ _ _ _ _ _ _ _ _ _ _ _ _ _ _ _ _ _ _ _ _ _ _ _ _ _ _ _ _ _ _ _ _ _ _ _ _ _ _ _ _ _ _ _ _ _ w3469 w3498] -> w1527
            tunnel: w1523 -> [_ _ _ _ _ _ _ _ _ _ _ _ _ _ _ _ _ _ _ _ w2466 w2491 w2510 w2533 w2551 w2572 w2590 w2612 _ _ _ _ w2690 w2720 w2745 w2765 _ _ _ _ w2851 w2877 _ _ _ _ _ _ _ _ _ _ _ _ _ _ _ _ _ _ _ _ _ _ _ _ _ _ _ _ _]
            tunnel: [_ _ _ _ _ _ _ _ _ _ _ _ _ _ _ _ _ _ _ w2434 w2466 w2490 w2509 w2532 w2551 w2572 w2590 w2612 _ _ _ _ w2690 w2720 w2745 w2765 _ _ _ _ w2851 w2877 _ _ _ _ _ _ _ _ _ _ _ _ _ _ _ _ _ _ _ _ _ _ _ _ _ _ _ _ _] -> w1522
            tunnel: [_ _ _ _ _ _ _ _ _ _ _ _ _ _ _ _ _ _ _ _ _ _ _ _ _ w2569 _ _ _ _ _ _ _ w2714 _ _ _ _ _ _ w2848 w2874 _ _ _ _ _ _ _ _ _ _ _ _ _ _ _ _ _ _ _ _ _ _ _ _ _ _ _ _ _] -> w1515
            tunnel: [_ _ _ _ _ _ _ _ _ _ _ _ _ _ _ _ _ _ _ _ _ _ _ _ _ w2568 _ _ _ _ _ _ _ w2715 _ _ _ _ _ _ w2847 w2873 _ _ _ _ _ _ _ _ _ _ _ _ _ _ _ _ _ _ _ _ _ _ _ _ _ _ _ _ _] -> w1513
            tunnel: [_ _ _ _ _ _ _ _ _ _ _ _ _ _ _ _ _ _ _ _ _ _ _ _ _ _ _ _ _ _ _ _ _ w2716 _ _ _ _ _ _ _ _ _ _ _ _ _ _ _ _ _ _ _ _ _ _ _ _ _ _ _ _ _ _ _ _ _ _ _ _ _] -> w1519
            tunnel: [_ _ _ _ _ _ _ _ _ _ _ _ _ _ _ w2332 _ _ _ _ _ _ _ _ _ _ _ _ _ _ _ _ _ _ _ _ _ _ _ _ _ _ _ _ _ _ _ _ _ _ _ _ _ _ _ _ _ _ _ _ _ _ _ _ _ _ _ _ _ _ _] -> w1502
            frame "Start1", Default {
              w1626 = FALSE ("SelectionState")
              n959 = local read "CueLed_baseline"() -> (w1625:bool)
              n960 = xnode "Read/Write Control"("FPGA VI Reference In"=w1628, "error in"=w1627, "SelectionState"=w1626, "LR_reward_Laser_l1"=w1626, "LR_wrong_Laser_l1"=w1626, "LR_reward_Event_l1"=w1626, "LR_wrong_Event_l1"=w1626, "Left(F)_or_Right(T)"=w1626, "ignoreWrong"=w1626, "SelectionState"=w1626, "LR_reward_Laser_l2"=w1626, "LR_wrong_laser_l2"=w1626, "LR_reward_Event_l2"=w1626, "LR_wrong_Event_l2"=w1626, "LC_Event_l1"=w1626, "LC_Laser_l1"=w1626, "LC_Laser_l2"=w1626, "LC_Event_l2"=w1626, "CueLed_Event"=w1626, "I_allReward"=w1626, "CueLed_Baseline"=w1625) -> ()  [unwired: 2 out]
            }
            frame "Start2" {
            }
            frame "Start3" {
            }
            frame "saveSettings1" {
              n961 = call "myRIO_BRig_RT_dataExp_Tcycle_Reward_min_L.vi"() -> ("output_Tcycle_Reward_min_L"=w1679:i32)  [unwired: 11 in]
              n962 = local read "Tcycle_Reward_min_L"() -> (w1678:u16)
              n963 = call "myRIO_BRig_RT_dataExp_Audio_freq__L.vi"() -> ("output_Audio_freq__L"=w1711:i32)  [unwired: 11 in]
              n964 = call "myRIO_BRig_RT_dataExp_Audio_freq__R.vi"() -> ("output_Audio_freq__R"=w1710:i32)  [unwired: 11 in]
              n965 = call "myRIO_BRig_RT_dataExp_Audio_amp__L.vi"() -> ("output_Audio_amp__L"=w1709:i32)  [unwired: 11 in]
              n966 = call "myRIO_BRig_RT_dataExp_Audio_amp__R.vi"() -> ("output_Audio_amp__R"=w1707:i32)  [unwired: 11 in]
              n967 = call "myRIO_BRig_RT_dataExp_TPB_min__L.vi"() -> ("output_TPB_min__L"=w1719:i32)  [unwired: 11 in]
              n968 = call "myRIO_BRig_RT_dataExp_TPB_min__R.vi"() -> ("output_TPB_min__R"=w1717:i32)  [unwired: 11 in]
              n969 = call "myRIO_BRig_RT_dataExp_TPB_max__L.vi"() -> ("output_TPB_max__L"=w1715:i32)  [unwired: 11 in]
              n970 = call "myRIO_BRig_RT_dataExp_TPB_max__R.vi"() -> ("output_TPB_max__R"=w1713:i32)  [unwired: 11 in]
              n971 = call "myRIO_BRig_RT_dataExp_Cue1Param_AudioLed_Count_Switch.vi"() -> ("output_Cue1Param_AudioLed_Count_Switch"=w1685:i32)  [unwired: 11 in]
              n972 = call "myRIO_BRig_RT_dataExp_Cue1Param_AudioLed_Probability_Switch.vi"() -> ("output_Cue1Param_AudioLed_Probability_Switch"=w1683:i32)  [unwired: 11 in]
              n973 = call "myRIO_BRig_RT_dataExp_Cue1Param_CueType_Switch.vi"() -> ("output_Cue1Param_CueType_Switch"=w1681:i32)  [unwired: 11 in]
              n974 = call "myRIO_BRig_RT_dataExp_ItrialUntilReward.vi"() -> ("output_I_trialUntilReward"=w1732:i32)  [unwired: 11 in]
              n975 = call "myRIO_BRig_RT_dataExp_IblockUntilReward.vi"() -> ("output_I_blockUntilReward"=w1728:i32)  [unwired: 11 in]
              n976 = call "myRIO_BRig_RT_dataExp_CueCycles.vi"() -> ("output_CueCycles"=w1727:i32)  [unwired: 11 in]
              n977 = call "myRIO_BRig_RT_dataExp_ENL_min.vi"() -> ("output_ENL_min"=w1725:i32)  [unwired: 11 in]
              n978 = call "myRIO_BRig_RT_dataExp_ENL_max.vi"() -> ("output_ENL_max"=w1723:i32)  [unwired: 11 in]
              n979 = call "myRIO_BRig_RT_dataExp_ENL_penalty.vi"() -> ("output_ENL_penalty"=w1721:i32)  [unwired: 11 in]
              n980 = local read "Audio_Freq__L"() -> (w1689:u8)
              n981 = local read "Audio_Freq__R"() -> (w1687:u8)
              n982 = local read "Audio_Amp__L"() -> (w1708:u16)
              n983 = local read "TpB_Min_L"() -> (w1718:u16)
              n984 = local read "TpB_Min_R"() -> (w1716:u16)
              n985 = local read "TpB_Max_L"() -> (w1714:u16)
              n986 = local read "TpB_Max_R"() -> (w1712:u16)
              n987 = local read "Audio_Amp__R"() -> (w1706:u16)
              n988 = local read "TrialUntilReward"() -> (w1731:bool)
              n989 = local read "CueCycles"() -> (w1726:u16)
              n990 = local read "Tcycle_ENL_min"() -> (w1724:u16)
              n991 = local read "Tcycle_ENL_max"() -> (w1722:u16)
              n992 = local read "Tcycle_ENLPenalty"() -> (w1720:u16)
              n993 = local read "Cue1Param_AudioLed_Count_Switch"() -> (w1684:u16)
              n994 = local read "Cue1Param_AudioLed_Probability_Switch"() -> (w1682:u16)
              n995 = local read "Cue1Param_CueType_Switch"() -> (w1680:u16)
              n996 = local read "Tcycle_Reward_max_L"() -> (w1676:u16)
              n997 = call "myRIO_BRig_RT_dataExp_Tcycle_Reward_max_L.vi"() -> ("output_Tcycle_Reward_max_L"=w1677:i32)  [unwired: 11 in]
              n998 = To Unsigned Word Integer(number=w1687) -> (unsigned 16bit integer=w1686:u16)
              n999 = To Unsigned Word Integer(number=w1689) -> (unsigned 16bit integer=w1688:u16)
              n1000 = Boolean To (0,1)(Boolean=w1731) -> (0, 1=w1730:i16)
              n1001 = To Unsigned Word Integer(number=w1730) -> (unsigned 16bit integer=w1729:u16)
              n1002 = call "myRIO_BRig_RT_dataExp_Tcycle_Reward_step_L.vi"() -> ("output_Tcycle_Reward_step_L"=w1675:i32)  [unwired: 11 in]
              n1003 = local read "Tcycle_Reward_step_L"() -> (w1674:u16)
              n1004 = local read "BUR_min"() -> (w1700:u16)
              n1005 = local read "BUR_max"() -> (w1701:u16)
              n1006 = Not Equal To 0?(x=w1700) -> (x != 0?=w1699:bool)
              n1007 = Not Equal To 0?(x=w1701) -> (x != 0?=w1698:bool)
              n1008 = And(x=w1699, y=w1698) -> (x .and. y?=w1697:bool)
              n1009 = Boolean To (0,1)(Boolean=w1697) -> (0, 1=w1702:i16)
              n1010 = To Unsigned Word Integer(number=w1702) -> (unsigned 16bit integer=w1696:u16)
              n1011 = Replace Array Subset(array=w1734, new element #1=w1729, index #1=w1732, new element #2=w1696, index #2=w1728, new element #3=w1726, index #3=w1727, new element #4=w1724, index #4=w1725, new element #5=w1722, index #5=w1723, new element #6=w1720, index #6=w1721, new element #7=w1718, index #7=w1719, new element #8=w1716, index #8=w1717, new element #9=w1714, index #9=w1715, new element #10=w1712, index #10=w1713, new element #11=w1688, index #11=w1711, new element #12=w1686, index #12=w1710, new element #13=w1708, index #13=w1709, new element #14=w1706, index #14=w1707, new element #15=w1684, index #15=w1685, new element #16=w1682, index #16=w1683, new element #17=w1680, index #17=w1681, new element #18=w1678, index #18=w1679, new element #19=w1676, index #19=w1677, new element #20=w1674, index #20=w1675) -> (w1733:u16[])
            }
            frame "saveSettings2" {
              n1012 = call "myRIO_BRig_RT_dataExp_Tcycle_Reward_min_R.vi"() -> ("output_Tcycle_Reward_min_R"=w1753:i32)  [unwired: 11 in]
              n1013 = local read "Tcycle_Reward_min_R"() -> (w1752:u16)
              n1014 = call "myRIO_BRig_RT_dataExp_Tcycle_Cue1_Audio_min.vi"() -> ("output_Tcycle_Cue1_Audio_min"=w1784:i32)  [unwired: 11 in]
              n1015 = call "myRIO_BRig_RT_dataExp_Tcycle_Cue1_Audio_max.vi"() -> ("output_Tcycle_Cue1_Audio_max"=w1783:i32)  [unwired: 11 in]
              n1016 = call "myRIO_BRig_RT_dataExp_Tcycle_Cue1Penalty_Audio.vi"() -> ("output_Tcycle_Cue1Penalty_Audio"=w1782:i32)  [unwired: 11 in]
              n1017 = call "myRIO_BRig_RT_dataExp_Tcycle_RewardPost.vi"() -> ("output_Tcycle_RewardPost"=w1790:i32)  [unwired: 11 in]
              n1018 = call "myRIO_BRig_RT_dataExp_Tcycle_Wrong.vi"() -> ("output_Tcycle_Wrong"=w1788:i32)  [unwired: 11 in]
              n1019 = call "myRIO_BRig_RT_dataExp_Tcycle_Timeout.vi"() -> ("output_Tcycle_Timeout"=w1786:i32)  [unwired: 11 in]
              n1020 = call "myRIO_BRig_RT_dataExp_Tcycle_Cue1_LED_min.vi"() -> ("output_Tcycle_Cue1_LED_min"=w1759:i32)  [unwired: 11 in]
              n1021 = call "myRIO_BRig_RT_dataExp_Tcycle_Cue1_LED_max.vi"() -> ("output_Tcycle_Cue1_LED_max"=w1758:i32)  [unwired: 11 in]
              n1022 = call "myRIO_BRig_RT_dataExp_Tcycle_Cue1Penalty_LED.vi"() -> ("output_Tcycle_Cue1Penalty_LED"=w1757:i32)  [unwired: 11 in]
              n1023 = call "myRIO_BRig_RT_dataExp_SolenoidProbability_L.vi"() -> ("output_SolenoidProbability_L"=w1769:i32)  [unwired: 11 in]
              n1024 = call "myRIO_BRig_RT_dataExp_SolenoidProbability_R.vi"() -> ("output_SolenoidProbability_R"=w1768:i32)  [unwired: 11 in]
              n1025 = call "myRIO_BRig_RT_dataExp_Cue1Param_AudioLed_Count_NS.vi"() -> ("output_Cue1Param_AudioLed_Count_NS"=w1765:i32)  [unwired: 11 in]
              n1026 = call "myRIO_BRig_RT_dataExp_Cue1Param_AudioLed_Probability_NS.vi"() -> ("output_Cue1Param_AudioLed_Probability_NS"=w1763:i32)  [unwired: 11 in]
              n1027 = call "myRIO_BRig_RT_dataExp_Cue1Param_CueType_NS.vi"() -> ("output_Cue1Param_CueType_NS"=w1761:i32)  [unwired: 11 in]
              n1028 = call "myRIO_BRig_RT_dataExp_nBlock.vi"() -> ("output_nBlock"=w1740:i32)  [unwired: 11 in]
              n1029 = call "myRIO_BRig_RT_dataExp_nTrial.vi"() -> ("output_nTrial"=w1742:i32)  [unwired: 11 in]
              n1030 = call "myRIO_BRig_RT_dataExp_runTime_seconds.vi"() -> ("output_RunTime_minutes"=w1745:i32)  [unwired: 11 in]
              n1031 = call "myRIO_BRig_RT_dataExp_Tcycle_Selection.vi"() -> ("output_Tcycle_Selection"=w1747:i32)  [unwired: 11 in]
              n1032 = local read "Tcycle_CuePenalty_Audio"() -> (w1778:u16)
              n1033 = local read "Tcycle_Cue_Audio_max"() -> (w1770:u16)
              n1034 = local read "Tcycle_Cue_Audio_min"() -> (w1771:u16)
              n1035 = local read "Tcycle_RewardPost"() -> (w1789:u16)
              n1036 = local read "Tcycle_Wrong"() -> (w1787:u16)
              n1037 = local read "Tcycle_Timeout"() -> (w1785:u16)
              n1038 = local read "Tcycle_Selection"() -> (w1746:u16)
              n1039 = local read "Cue1Param_AudioLed_Count_NS"() -> (w1764:u16)
              n1040 = local read "Cue1Param_AudioLed_Probability_NS"() -> (w1762:u16)
              n1041 = local read "Cue1Param_CueType_NS"() -> (w1760:u16)
              n1042 = local read "Tcycle_CuePenalty_LED"() -> (w1754:u16)
              n1043 = local read "SolenoidProbability_R"() -> (w1766:u16)
              n1044 = local read "SolenoidProbability_L"() -> (w1767:u16)
              n1045 = local read "Tcycle_Cue_LED_min"() -> (w1756:u16)
              n1046 = local read "Tcycle_Cue_LED_max"() -> (w1755:u16)
              n1047 = local read "Tcycle_Reward_max_R"() -> (w1750:u16)
              n1048 = call "myRIO_BRig_RT_dataExp_Tcycle_Reward_max_R.vi"() -> ("output_Tcycle_Reward_max_R"=w1751:i32)  [unwired: 11 in]
              n1049 = call "myRIO_BRig_RT_dataExp_Tcycle_Reward_step_R.vi"() -> ("output_Tcycle_Reward_step_R"=w1749:i32)  [unwired: 11 in]
              n1050 = local read "Tcycle_Reward_step_R"() -> (w1748:u16)
              n1051 = Replace Array Subset(array=w1792, new element #1=u16 0, index #1=w1740, new element #2=u16 0, index #2=w1742, new element #3=u16 0, index #3=w1745, new element #4=w1746, index #4=w1747, new element #5=w1789, index #5=w1790, new element #6=w1787, index #6=w1788, new element #7=w1785, index #7=w1786, new element #8=w1771, index #8=w1784, new element #9=w1770, index #9=w1783, new element #10=w1778, index #10=w1782, new element #11=w1767, index #11=w1769, new element #12=w1766, index #12=w1768, new element #13=w1764, index #13=w1765, new element #14=w1762, index #14=w1763, new element #15=w1760, index #15=w1761, new element #16=w1756, index #16=w1759, new element #17=w1755, index #17=w1758, new element #18=w1754, index #18=w1757, new element #19=w1752, index #19=w1753, new element #20=w1750, index #20=w1751, new element #21=w1748, index #21=w1749) -> (w1791:u16[])
            }
            frame "saveSettings3" {
              w1804 = 100.0 ("y")
              n1052 = call "myRIO_BRig_RT_dataExp_laser1_Freq.vi"() -> ("output_laser1_Freq"=w1837:i32)  [unwired: 11 in]
              n1053 = call "myRIO_BRig_RT_dataExp_laser1_Tpeak.vi"() -> ("output_laser1_Tpeak"=w1832:i32)  [unwired: 11 in]
              n1054 = call "myRIO_BRig_RT_dataExp_laser1_Tshutter.vi"() -> ("output_laser1_Tshutter"=w1827:i32)  [unwired: 11 in]
              n1055 = call "myRIO_BRig_RT_dataExp_FPGA_f_count2ms.vi"() -> ("output_FPGA_f_count2ms"=w1822:i32)  [unwired: 11 in]
              n1056 = call "myRIO_BRig_RT_dataExp_laser1_Power_min.vi"() -> ("output_laser1_Power_min"=w1817:i32)  [unwired: 11 in]
              n1057 = call "myRIO_BRig_RT_dataExp_laser1_Power_max.vi"() -> ("output_laser1_Power_max"=w1810:i32)  [unwired: 11 in]
              n1058 = call "myRIO_BRig_RT_dataExp_laser1_Power_step.vi"() -> ("output_laser1_Power_step"=w1809:i32)  [unwired: 11 in]
              n1059 = call "myRIO_BRig_RT_dataExp_laser1_duration.vi"() -> ("output_laser1_duration"=w1812:i32)  [unwired: 11 in]
              n1060 = local read "Laser_Tshutter_l1"() -> (w1824:dbl)
              n1061 = local read "Laser_Tpeak_l1"() -> (w1829:dbl)
              n1062 = local read "Laser_power_max_l1"() -> (w1803:dbl)
              n1063 = local read "Laser_power_step_l1"() -> (w1802:dbl)
              n1064 = local read "Laser_power_min_l1"() -> (w1814:dbl)
              n1065 = local read "Laser_Freq_l1"() -> (w1836:dbl)
              n1066 = call "myRIO_BRig_RT_dataExp_BUR_min.vi"() -> ("output_BUR_min"=w1852:i32)  [unwired: 11 in]
              n1067 = call "myRIO_BRig_RT_dataExp_BUR_max.vi"() -> ("output_BUR_max"=w1850:i32)  [unwired: 11 in]
              n1068 = call "myRIO_BRig_RT_dataExp_Audio_sp__L.vi"() -> ("output_Audio_sp__L"=w1847:i32)  [unwired: 11 in]
              n1069 = call "myRIO_BRig_RT_dataExp_Audio_sp__R.vi"() -> ("output_Audio_sp__R"=w1846:i32)  [unwired: 11 in]
              n1070 = local read "FPGA_count2ms"() -> (w1819:dbl)
              n1071 = local read "sp_LeftSpout"() -> (w1845:u16)
              n1072 = local read "BUR_max"() -> (w1849:u16)
              n1073 = local read "sp_RightSpout"() -> (w1844:u16)
              n1074 = local read "BUR_min"() -> (w1851:u16)
              n1075 = Multiply(x=w1836, y=w1804) -> (x*y=w1835:dbl)
              n1076 = Multiply(x=w1829, y=w1804) -> (x*y=w1831:dbl)
              n1077 = Multiply(x=w1824, y=w1804) -> (x*y=w1826:dbl)
              n1078 = Multiply(x=w1819, y=w1804) -> (x*y=w1821:dbl)
              n1079 = Multiply(x=w1814, y=w1804) -> (x*y=w1816:dbl)
              n1080 = Multiply(x=w1803, y=w1804) -> (x*y=w1808:dbl)
              n1081 = Multiply(x=w1802, y=w1804) -> (x*y=w1806:dbl)
              n1082 = Round To Nearest(number=w1835) -> (nearest integer value=w1834:dbl)
              n1083 = Round To Nearest(number=w1831) -> (nearest integer value=w1830:dbl)
              n1084 = Round To Nearest(number=w1826) -> (nearest integer value=w1825:dbl)
              n1085 = Round To Nearest(number=w1821) -> (nearest integer value=w1820:dbl)
              n1086 = Round To Nearest(number=w1816) -> (nearest integer value=w1815:dbl)
              n1087 = Round To Nearest(number=w1808) -> (nearest integer value=w1807:dbl)
              n1088 = Round To Nearest(number=w1806) -> (nearest integer value=w1805:dbl)
              n1089 = To Unsigned Word Integer(number=w1834) -> (unsigned 16bit integer=w1833:u16)
              n1090 = To Unsigned Word Integer(number=w1830) -> (unsigned 16bit integer=w1828:u16)
              n1091 = To Unsigned Word Integer(number=w1825) -> (unsigned 16bit integer=w1823:u16)
              n1092 = To Unsigned Word Integer(number=w1820) -> (unsigned 16bit integer=w1818:u16)
              n1093 = To Unsigned Word Integer(number=w1815) -> (unsigned 16bit integer=w1813:u16)
              n1094 = To Unsigned Word Integer(number=w1807) -> (unsigned 16bit integer=w1801:u16)
              n1095 = To Unsigned Word Integer(number=w1805) -> (unsigned 16bit integer=w1800:u16)
              n1096 = local read "Laser_duration_l1"() -> (w1811:u16)
              n1097 = Replace Array Subset(array=w1853, new element #1=w1851, index #1=w1852, new element #2=w1849, index #2=w1850, new element #3=w1845, index #3=w1847, new element #4=w1844, index #4=w1846, new element #5=w1833, index #5=w1837, new element #6=w1828, index #6=w1832, new element #7=w1823, index #7=w1827, new element #8=w1818, index #8=w1822, new element #9=w1813, index #9=w1817, new element #10=w1801, index #10=w1810, new element #11=w1800, index #11=w1809, new element #12=w1811, index #12=w1812) -> (w1848:u16[])
            }
            frame "saveSettings4" {
              w1873 = 100.0 ("y")
              n1098 = call "myRIO_BRig_RT_dataExp_laser2_Freq.vi"() -> ("output_laser2_Freq"=w1862:i32)  [unwired: 11 in]
              n1099 = call "myRIO_BRig_RT_dataExp_laser2_Tpeak.vi"() -> ("output_laser2_Tpeak"=w1864:i32)  [unwired: 11 in]
              n1100 = call "myRIO_BRig_RT_dataExp_laser2_Tshutter.vi"() -> ("output_laser2_Tshutter"=w1866:i32)  [unwired: 11 in]
              n1101 = call "myRIO_BRig_RT_dataExp_laser2_Power_min.vi"() -> ("output_laser2_Power_min"=w1881:i32)  [unwired: 11 in]
              n1102 = call "myRIO_BRig_RT_dataExp_laser2_Power_max.vi"() -> ("output_laser2_Power_max"=w1880:i32)  [unwired: 11 in]
              n1103 = call "myRIO_BRig_RT_dataExp_laser2_Power_step.vi"() -> ("output_laser2_Power_step"=w1879:i32)  [unwired: 11 in]
              n1104 = call "myRIO_BRig_RT_dataExp_laser2_duration.vi"() -> ("output_laser2_duration"=w1878:i32)  [unwired: 11 in]
              n1105 = call "myRIO_BRig_RT_dataExp_CueLed_Freq.vi"() -> ("output_CueLed_Freq"=w1870:i32)  [unwired: 11 in]
              n1106 = call "myRIO_BRig_RT_dataExp_CueLed_Tpeak.vi"() -> ("output_CueLed_Tpeak"=w1869:i32)  [unwired: 11 in]
              n1107 = local read "Laser_Tshutter_l2"() -> (w1896:dbl)
              n1108 = local read "Laser_Tpeak_l2"() -> (w1899:dbl)
              n1109 = local read "Laser_power_max_l2"() -> (w1886:dbl)
              n1110 = local read "Laser_power_step_l2"() -> (w1885:dbl)
              n1111 = local read "Laser_power_min_l2"() -> (w1893:dbl)
              n1112 = local read "Laser_Freq_l2"() -> (w1904:dbl)
              n1113 = local read "CueLed_Tpeak"() -> (w1871:dbl)
              n1114 = local read "CueLed_Freq"() -> (w1872:dbl)
              n1115 = Multiply(x=w1904, y=w1873) -> (x*y=w1903:dbl)
              n1116 = Multiply(x=w1899, y=w1873) -> (x*y=w1901:dbl)
              n1117 = Multiply(x=w1896, y=w1873) -> (x*y=w1898:dbl)
              n1118 = Multiply(x=w1893, y=w1873) -> (x*y=w1895:dbl)
              n1119 = Multiply(x=w1886, y=w1873) -> (x*y=w1890:dbl)
              n1120 = Multiply(x=w1885, y=w1873) -> (x*y=w1888:dbl)
              n1121 = Multiply(x=w1872, y=w1873) -> (x*y=w1874:dbl)
              n1122 = Multiply(x=w1871, y=w1873) -> (x*y=w1875:dbl)
              n1123 = Round To Nearest(number=w1903) -> (nearest integer value=w1902:dbl)
              n1124 = Round To Nearest(number=w1901) -> (nearest integer value=w1900:dbl)
              n1125 = Round To Nearest(number=w1898) -> (nearest integer value=w1897:dbl)
              n1126 = Round To Nearest(number=w1895) -> (nearest integer value=w1894:dbl)
              n1127 = Round To Nearest(number=w1890) -> (nearest integer value=w1889:dbl)
              n1128 = Round To Nearest(number=w1888) -> (nearest integer value=w1887:dbl)
              n1129 = Round To Nearest(number=w1874) -> (nearest integer value=w1877:dbl)
              n1130 = Round To Nearest(number=w1875) -> (nearest integer value=w1876:dbl)
              n1131 = To Unsigned Word Integer(number=w1902) -> (unsigned 16bit integer=w1861:u16)
              n1132 = To Unsigned Word Integer(number=w1900) -> (unsigned 16bit integer=w1863:u16)
              n1133 = To Unsigned Word Integer(number=w1897) -> (unsigned 16bit integer=w1865:u16)
              n1134 = To Unsigned Word Integer(number=w1894) -> (unsigned 16bit integer=w1892:u16)
              n1135 = To Unsigned Word Integer(number=w1889) -> (unsigned 16bit integer=w1884:u16)
              n1136 = To Unsigned Word Integer(number=w1887) -> (unsigned 16bit integer=w1883:u16)
              n1137 = To Unsigned Word Integer(number=w1877) -> (unsigned 16bit integer=w1868:u16)
              n1138 = To Unsigned Word Integer(number=w1876) -> (unsigned 16bit integer=w1867:u16)
              n1139 = local read "Laser_duration_l2"() -> (w1891:u16)
              n1140 = Replace Array Subset(array=w1912, new element #1=w1861, index #1=w1862, new element #2=w1863, index #2=w1864, new element #3=w1865, index #3=w1866, new element #4=w1892, index #4=w1881, new element #5=w1884, index #5=w1880, new element #6=w1883, index #6=w1879, new element #7=w1891, index #7=w1878, new element #8=w1868, index #8=w1870, new element #9=w1867, index #9=w1869) -> (w1911:u16[])
            }
            frame "saveSettings_LC_ENL_l1" {
              # "Selection First"
              # "Count"
              # "Tdelay"
              # "Probability"
              # "OnOff"
              # "Block"
              # "delayOpt"
              # "Count"
              # "Tdelay"
              # "Probability"
              # "OnOff"
              # "Block"
              # "ENL1 All"
              # "delayOpt"
              # "Count"
              # "Tdelay"
              # "Probability"
              # "OnOff"
              # "Block"
              # "ENL1 First"
              n1141 = local read "LC_ENL1_delayOpt_Switch_l1"() -> (w1950:bool)
              n1142 = call "myRIO_BRig_RT_dataLC_ENL1_Block_NS_l1.vi"() -> ("output_ENL1_All_Block"=w1947:i32)  [unwired: 11 in]
              n1143 = call "myRIO_BRig_RT_dataLC_ENL1_OnOff_NS_l1.vi"() -> ("output_ENL1_OnOff_NS_l1"=w1937:i32)  [unwired: 11 in]
              n1144 = call "myRIO_BRig_RT_dataLC_ENL1_Probability_NS_l1.vi"() -> ("output_ENL1_Probability_NS_l1"=w1936:i32)  [unwired: 11 in]
              n1145 = call "myRIO_BRig_RT_dataLC_ENL1_Tdelay_NS_l1.vi"() -> ("output_ENL1_Tdelay_NS_l1"=w1935:i32)  [unwired: 11 in]
              n1146 = call "myRIO_BRig_RT_dataLC_ENL1_Count_NS_l1.vi"() -> ("output_ENL1_Count_NS_l1"=w1934:i32)  [unwired: 11 in]
              n1147 = call "myRIO_BRig_RT_dataLC_ENL1_delayOpt_NS_l1.vi"() -> ("output_ENL1_delayOpt_NS_l1"=w1933:i32)  [unwired: 11 in]
              n1148 = call "myRIO_BRig_RT_dataLC_ENL1_Block_Switch_l1.vi"() -> ("output_ENL1_Block_Switch_l1"=w1969:i32)  [unwired: 11 in]
              n1149 = call "myRIO_BRig_RT_dataLC_ENL1_OnOff_Switch_l1.vi"() -> ("output_ENL1_OnOff_Switch_l1"=w1967:i32)  [unwired: 11 in]
              n1150 = call "myRIO_BRig_RT_dataLC_ENL1_Probability_Switch_l1.vi"() -> ("output_ENL1_Probability_Switch_l1"=w1963:i32)  [unwired: 11 in]
              n1151 = call "myRIO_BRig_RT_dataLC_ENL1_Tdelay_Switch_l1.vi"() -> ("output_ENL1_Tdelay_Switch_l1"=w1961:i32)  [unwired: 11 in]
              n1152 = call "myRIO_BRig_RT_dataLC_ENL1_Count_Switch_l1.vi"() -> ("output_ENL1_Count_Switch_l1"=w1959:i32)  [unwired: 11 in]
              n1153 = call "myRIO_BRig_RT_dataLC_ENL1_delayOpt_Switch_l1.vi"() -> ("output_ENL1_delayOpt_Switch_l1"=w1949:i32)  [unwired: 11 in]
              n1154 = local read "LC_ENL1_Count_Switch_l1"() -> (w1958:u16)
              n1155 = local read "LC_ENL1_Probability_Switch_l1"() -> (w1962:u16)
              n1156 = local read "LC_ENL1_Block_Switch_l1"() -> (w1968:u16)
              n1157 = local read "LC_ENL1_Tdelay_Switch_l1"() -> (w1960:u16)
              n1158 = local read "LC_ENL1_OnOff_Switch_l1"() -> (w1966:bool)
              n1159 = call "myRIO_BRig_RT_dataLC_Selection_Block_Switch_l1.vi"() -> ("output_Selection_Block_Switch_l1"=w1931:i32)  [unwired: 11 in]
              n1160 = call "myRIO_BRig_RT_dataLC_Selection_OnOff_Switch_l1.vi"() -> ("output_Selection_OnOff_Switch_l1"=w1930:i32)  [unwired: 11 in]
              n1161 = call "myRIO_BRig_RT_dataLC_Selection_Probability_Switch_l1.vi"() -> ("output_Selection_Probability_Switch_l1"=w1929:i32)  [unwired: 11 in]
              n1162 = call "myRIO_BRig_RT_dataLC_Selection_Tdelay_Switch_l1.vi"() -> ("output_Selection_Tdelay_Switch_l1"=w1928:i32)  [unwired: 11 in]
              n1163 = call "myRIO_BRig_RT_dataLC_Selection_Count_Switch_l1.vi"() -> ("output_Selection_Count_Switch_l1"=w1927:i32)  [unwired: 11 in]
              n1164 = local read "LC_ENL1_OnOff_NS_l1"() -> (w1943:bool)
              n1165 = local read "LC_ENL1_Probability_NS_l1"() -> (w1941:u16)
              n1166 = local read "LC_ENL1_delayOpt_NS_l1"() -> (w1939:bool)
              n1167 = local read "LC_Sel_Probability_Switch_l1"() -> (w1922:u16)
              n1168 = local read "LC_ENL1_Tdelay_NS_l1"() -> (w1932:u16)
              n1169 = local read "LC_ENL1_Block_NS_l1"() -> (w1944:u16)
              n1170 = local read "LC_ENL1_Count_NS_l1"() -> (w1940:u16)
              n1171 = local read "LC_Sel_Tdelay_Switch_l1"() -> (w1921:u16)
              n1172 = local read "LC_Sel_OnOff_Switch_l1"() -> (w1925:bool)
              n1173 = local read "LC_Sel_Count_Switch_l1"() -> (w1920:u16)
              n1174 = local read "LC_Sel_Block_Switch_l1"() -> (w1924:u16)
              n1175 = Boolean To (0,1)(Boolean=w1950) -> (0, 1=w1951:i16)
              n1176 = Boolean To (0,1)(Boolean=w1966) -> (0, 1=w1965:i16)
              n1177 = Boolean To (0,1)(Boolean=w1943) -> (0, 1=w1946:i16)
              n1178 = To Unsigned Word Integer(number=w1951) -> (unsigned 16bit integer=w1948:u16)
              n1179 = To Unsigned Word Integer(number=w1965) -> (unsigned 16bit integer=w1964:u16)
              n1180 = Boolean To (0,1)(Boolean=w1939) -> (0, 1=w1945:i16)
              n1181 = To Unsigned Word Integer(number=w1946) -> (unsigned 16bit integer=w1942:u16)
              n1182 = Boolean To (0,1)(Boolean=w1925) -> (0, 1=w1926:i16)
              n1183 = To Unsigned Word Integer(number=w1945) -> (unsigned 16bit integer=w1938:u16)
              n1184 = To Unsigned Word Integer(number=w1926) -> (unsigned 16bit integer=w1923:u16)
              n1185 = Replace Array Subset(array=w1970, new element #1=w1968, index #1=w1969, new element #2=w1964, index #2=w1967, new element #3=w1962, index #3=w1963, new element #4=w1960, index #4=w1961, new element #5=w1958, index #5=w1959, new element #6=w1948, index #6=w1949, new element #7=w1944, index #7=w1947, new element #8=w1942, index #8=w1937, new element #9=w1941, index #9=w1936, new element #10=w1932, index #10=w1935, new element #11=w1940, index #11=w1934, new element #12=w1938, index #12=w1933, new element #13=w1924, index #13=w1931, new element #14=w1923, index #14=w1930, new element #15=w1922, index #15=w1929, new element #16=w1921, index #16=w1928, new element #17=w1920, index #17=w1927) -> (w1971:u16[])
            }
            frame "saveSettings_LC_ENL_l2" {
              # "Selection First"
              # "Count"
              # "Tdelay"
              # "Probability"
              # "OnOff"
              # "Block"
              # "delayOpt"
              # "Count"
              # "Tdelay"
              # "Probability"
              # "OnOff"
              # "Block"
              # "ENL1 All"
              # "delayOpt"
              # "Count"
              # "Tdelay"
              # "Probability"
              # "OnOff"
              # "Block"
              # "ENL1 First"
              n1186 = call "myRIO_BRig_RT_dataLC_ENL1_Block_Switch_l2.vi"() -> ("output_ENL1_Block_Switch_l2"=w1990:i32)  [unwired: 11 in]
              n1187 = call "myRIO_BRig_RT_dataLC_ENL1_OnOff_Switch_l2.vi"() -> ("output_ENL1_OnOff_Switch_l2"=w1991:i32)  [unwired: 11 in]
              n1188 = call "myRIO_BRig_RT_dataLC_ENL1_Probability_Switch_l2.vi"() -> ("output_ENL1_Probability_Switch_l2"=w1992:i32)  [unwired: 11 in]
              n1189 = call "myRIO_BRig_RT_dataLC_ENL1_Tdelay_Switch_l2.vi"() -> ("output_ENL1_Tdelay_Switch_l2"=w1993:i32)  [unwired: 11 in]
              n1190 = call "myRIO_BRig_RT_dataLC_ENL1_Count_Switch_l2.vi"() -> ("output_ENL1_Count_Switch_l2"=w1994:i32)  [unwired: 11 in]
              n1191 = call "myRIO_BRig_RT_dataLC_ENL1_delayOpt_Switch_l2.vi"() -> ("output_ENL1_delayOpt_Switch_l2"=w1995:i32)  [unwired: 11 in]
              n1192 = local read "LC_ENL1_delayOpt_Switch_l2"() -> (w2015:bool)
              n1193 = call "myRIO_BRig_RT_dataLC_ENL1_Block_NS_l2.vi"() -> ("output_ENL1_Block_NS_l2"=w1984:i32)  [unwired: 11 in]
              n1194 = call "myRIO_BRig_RT_dataLC_ENL1_OnOff_NS_l2.vi"() -> ("output_ENL1_OnOff_NS_l2"=w1985:i32)  [unwired: 11 in]
              n1195 = call "myRIO_BRig_RT_dataLC_ENL1_Probability_NS_l2.vi"() -> ("output_ENL1_Probability_NS_l2"=w1986:i32)  [unwired: 11 in]
              n1196 = call "myRIO_BRig_RT_dataLC_ENL1_Tdelay_NS_l2.vi"() -> ("output_ENL1_Tdelay_NS_l2"=w1987:i32)  [unwired: 11 in]
              n1197 = call "myRIO_BRig_RT_dataLC_ENL1_Count_NS_l2.vi"() -> ("output_ENL1_Count_NS_l2"=w1988:i32)  [unwired: 11 in]
              n1198 = call "myRIO_BRig_RT_dataLC_ENL1_delayOpt_NS_l2.vi"() -> ("output_ENL1_delayOpt_NS_l2"=w1989:i32)  [unwired: 11 in]
              n1199 = local read "LC_ENL1_Count_Switch_l2"() -> (w2023:u16)
              n1200 = local read "LC_ENL1_Probability_Switch_l2"() -> (w2025:u16)
              n1201 = local read "LC_ENL1_Block_Switch_l2"() -> (w2029:u16)
              n1202 = local read "LC_ENL1_Tdelay_Switch_l2"() -> (w2024:u16)
              n1203 = local read "LC_ENL1_OnOff_Switch_l2"() -> (w2028:bool)
              n1204 = call "myRIO_BRig_RT_dataLC_Selection_Block_Switch_l2.vi"() -> ("output_Selection_Block_Switch_l2"=w1983:i32)  [unwired: 11 in]
              n1205 = call "myRIO_BRig_RT_dataLC_Selection_OnOff_Switch_l2.vi"() -> ("output_Selection_OnOff_Switch_l2"=w1982:i32)  [unwired: 11 in]
              n1206 = call "myRIO_BRig_RT_dataLC_Selection_Probability_Switch_l2.vi"() -> ("output_Selection_Probability_Switch_l1"=w1981:i32)  [unwired: 11 in]
              n1207 = call "myRIO_BRig_RT_dataLC_Selection_Tdelay_Switch_l2.vi"() -> ("output_Selection_Tdelay_Switch_l2"=w1980:i32)  [unwired: 11 in]
              n1208 = call "myRIO_BRig_RT_dataLC_Selection_Count_Switch_l2.vi"() -> ("output_Selection_Count_Switch_l2"=w1979:i32)  [unwired: 11 in]
              n1209 = local read "LC_ENL1_OnOff_NS_l2"() -> (w2010:bool)
              n1210 = local read "LC_ENL1_Probability_NS_l2"() -> (w2008:u16)
              n1211 = local read "LC_ENL1_delayOpt_NS_l2"() -> (w2006:bool)
              n1212 = local read "LC_Sel_Probability_Switch_l2"() -> (w1999:u16)
              n1213 = local read "LC_ENL1_Tdelay_NS_l2"() -> (w2004:u16)
              n1214 = local read "LC_ENL1_Block_NS_l2"() -> (w2011:u16)
              n1215 = local read "LC_ENL1_Count_NS_l2"() -> (w2007:u16)
              n1216 = local read "LC_Sel_Tdelay_Switch_l2"() -> (w1998:u16)
              n1217 = local read "LC_Sel_OnOff_Switch_l2"() -> (w2002:bool)
              n1218 = local read "LC_Sel_Count_Switch_l2"() -> (w1997:u16)
              n1219 = local read "LC_Sel_Block_Switch_l2"() -> (w2001:u16)
              n1220 = Boolean To (0,1)(Boolean=w2015) -> (0, 1=w2016:i16)
              n1221 = Boolean To (0,1)(Boolean=w2028) -> (0, 1=w2027:i16)
              n1222 = Boolean To (0,1)(Boolean=w2010) -> (0, 1=w2013:i16)
              n1223 = To Unsigned Word Integer(number=w2016) -> (unsigned 16bit integer=w2014:u16)
              n1224 = To Unsigned Word Integer(number=w2027) -> (unsigned 16bit integer=w2026:u16)
              n1225 = Boolean To (0,1)(Boolean=w2006) -> (0, 1=w2012:i16)
              n1226 = To Unsigned Word Integer(number=w2013) -> (unsigned 16bit integer=w2009:u16)
              n1227 = Boolean To (0,1)(Boolean=w2002) -> (0, 1=w2003:i16)
              n1228 = To Unsigned Word Integer(number=w2012) -> (unsigned 16bit integer=w2005:u16)
              n1229 = To Unsigned Word Integer(number=w2003) -> (unsigned 16bit integer=w2000:u16)
              n1230 = Replace Array Subset(array=w2030, new element #1=w2029, index #1=w1990, new element #2=w2026, index #2=w1991, new element #3=w2025, index #3=w1992, new element #4=w2024, index #4=w1993, new element #5=w2023, index #5=w1994, new element #6=w2014, index #6=w1995, new element #7=w2011, index #7=w1984, new element #8=w2009, index #8=w1985, new element #9=w2008, index #9=w1986, new element #10=w2004, index #10=w1987, new element #11=w2007, index #11=w1988, new element #12=w2005, index #12=w1989, new element #13=w2001, index #13=w1983, new element #14=w2000, index #14=w1982, new element #15=w1999, index #15=w1981, new element #16=w1998, index #16=w1980, new element #17=w1997, index #17=w1979) -> (w2031:u16[])
            }
            frame "saveSettings_LC_Cue_l1" {
              # "Selection All"
              # "Count"
              # "Tdelay"
              # "Probability"
              # "OnOff"
              # "Block"
              # "delayOpt"
              # "Count"
              # "Tdelay"
              # "Probability"
              # "OnOff"
              # "Block"
              # "Cue1 All"
              # "delayOpt"
              # "Count"
              # "Tdelay"
              # "Probability"
              # "OnOff"
              # "Block"
              # "Cue1 First"
              n1231 = call "myRIO_BRig_RT_dataLC_Cue1_delayOpt_Switch_l1.vi"() -> ("output_Cue1_delayOpt_Switch_l1"=w2070:i32)  [unwired: 11 in]
              n1232 = call "myRIO_BRig_RT_dataLC_Cue1_Block_Switch_l1.vi"() -> ("output_Cue1_Block_Switch_l1"=w2089:i32)  [unwired: 11 in]
              n1233 = call "myRIO_BRig_RT_dataLC_Cue1_OnOff_Switch_l1.vi"() -> ("output_Cue1_OnOff_Switch_l1"=w2087:i32)  [unwired: 11 in]
              n1234 = call "myRIO_BRig_RT_dataLC_Cue1_Probability_Switch_l1.vi"() -> ("output_Cue1_Probability_Switch_l1"=w2083:i32)  [unwired: 11 in]
              n1235 = call "myRIO_BRig_RT_dataLC_Cue1_Tdelay_Switch_l1.vi"() -> ("output_Cue1_Tdelay_Switch_l1"=w2081:i32)  [unwired: 11 in]
              n1236 = call "myRIO_BRig_RT_dataLC_Cue1_Count_Switch_l1.vi"() -> ("output_Cue1_Count_Switch_l1"=w2079:i32)  [unwired: 11 in]
              n1237 = local read "LC_Cue1_delayOpt_Switch_l1"() -> (w2069:bool)
              n1238 = call "myRIO_BRig_RT_dataLC_Cue1_Block_NS_l1.vi"() -> ("output_Cue1_Block_NS_l1"=w2067:i32)  [unwired: 11 in]
              n1239 = call "myRIO_BRig_RT_dataLC_Cue1_OnOff_NS_l1.vi"() -> ("output_Cue1_OnOff_NS_l1"=w2066:i32)  [unwired: 11 in]
              n1240 = call "myRIO_BRig_RT_dataLC_Cue1_Probability_NS_l1.vi"() -> ("output_Cue1_l1_All_Probability"=w2065:i32)  [unwired: 11 in]
              n1241 = call "myRIO_BRig_RT_dataLC_Cue1_Tdelay_NS_l1.vi"() -> ("output_Cue1_Tdelay_NS_l1"=w2064:i32)  [unwired: 11 in]
              n1242 = call "myRIO_BRig_RT_dataLC_Cue1_Count_NS_l1.vi"() -> ("output_Cue1_Count_NS_l1"=w2063:i32)  [unwired: 11 in]
              n1243 = call "myRIO_BRig_RT_dataLC_Cue1_delayOpt_NS_l1.vi"() -> ("output_Cue1_delayOpt_NS_l1"=w2062:i32)  [unwired: 11 in]
              n1244 = local read "LC_Cue1_Count_Switch_l1"() -> (w2078:u16)
              n1245 = local read "LC_Cue1_Probability_Switch_l1"() -> (w2082:u16)
              n1246 = local read "LC_Cue1_Block_Switch_l1"() -> (w2088:u16)
              n1247 = local read "LC_Cue1_Tdelay_Switch_l1"() -> (w2080:u16)
              n1248 = local read "LC_Cue1_OnOff_Switch_l1"() -> (w2086:bool)
              n1249 = local read "LC_Cue1_OnOff_NS_l1"() -> (w2058:bool)
              n1250 = call "myRIO_BRig_RT_dataLC_Selection_Block_NS_l1.vi"() -> ("output_Selection_Block_NS_l1"=w2051:i32)  [unwired: 11 in]
              n1251 = call "myRIO_BRig_RT_dataLC_Selection_OnOff_NS_l1.vi"() -> ("output_Selection_OnOff_NS_l1"=w2050:i32)  [unwired: 11 in]
              n1252 = call "myRIO_BRig_RT_dataLC_Selection_Probability_NS_l1.vi"() -> ("output_Selection_Probability_NS_l1"=w2049:i32)  [unwired: 11 in]
              n1253 = call "myRIO_BRig_RT_dataLC_Selection_Tdelay_NS_l1.vi"() -> ("output_Selection_Tdelay_NS_l1"=w2048:i32)  [unwired: 11 in]
              n1254 = call "myRIO_BRig_RT_dataLC_Selection_Count_NS_l1.vi"() -> ("output_Selection_Count_NS_l1"=w2041:i32)  [unwired: 11 in]
              n1255 = local read "LC_Cue1_delayOpt_NS_l1"() -> (w2059:bool)
              n1256 = local read "LC_Cue1_Probability_NS_l1"() -> (w2055:u16)
              n1257 = local read "LC_Cue1_Tdelay_NS_l1"() -> (w2054:u16)
              n1258 = local read "LC_Cue1_Count_NS_l1"() -> (w2053:u16)
              n1259 = local read "LC_Cue1_Block_NS_l1"() -> (w2057:u16)
              n1260 = local read "LC_Sel_Probability_NS_l1"() -> (w2043:u16)
              n1261 = local read "LC_Sel_Tdelay_NS_l1"() -> (w2042:u16)
              n1262 = local read "LC_Sel_OnOff_NS_l1"() -> (w2045:bool)
              n1263 = local read "LC_Sel_Count_NS_l1"() -> (w2040:u16)
              n1264 = local read "LC_Sel_Block_NS_l1"() -> (w2047:u16)
              n1265 = Boolean To (0,1)(Boolean=w2069) -> (0, 1=w2071:i16)
              n1266 = Boolean To (0,1)(Boolean=w2086) -> (0, 1=w2085:i16)
              n1267 = Boolean To (0,1)(Boolean=w2058) -> (0, 1=w2061:i16)
              n1268 = To Unsigned Word Integer(number=w2071) -> (unsigned 16bit integer=w2068:u16)
              n1269 = To Unsigned Word Integer(number=w2085) -> (unsigned 16bit integer=w2084:u16)
              n1270 = To Unsigned Word Integer(number=w2061) -> (unsigned 16bit integer=w2056:u16)
              n1271 = Boolean To (0,1)(Boolean=w2059) -> (0, 1=w2060:i16)
              n1272 = Boolean To (0,1)(Boolean=w2045) -> (0, 1=w2046:i16)
              n1273 = To Unsigned Word Integer(number=w2060) -> (unsigned 16bit integer=w2052:u16)
              n1274 = To Unsigned Word Integer(number=w2046) -> (unsigned 16bit integer=w2044:u16)
              n1275 = Replace Array Subset(array=w2090, new element #1=w2088, index #1=w2089, new element #2=w2084, index #2=w2087, new element #3=w2082, index #3=w2083, new element #4=w2080, index #4=w2081, new element #5=w2078, index #5=w2079, new element #6=w2068, index #6=w2070, new element #7=w2057, index #7=w2067, new element #8=w2056, index #8=w2066, new element #9=w2055, index #9=w2065, new element #10=w2054, index #10=w2064, new element #11=w2053, index #11=w2063, new element #12=w2052, index #12=w2062, new element #13=w2047, index #13=w2051, new element #14=w2044, index #14=w2050, new element #15=w2043, index #15=w2049, new element #16=w2042, index #16=w2048, new element #17=w2040, index #17=w2041) -> (w2091:u16[])
            }
            frame "saveSettings_LC_Cue_l2" {
              # "Selection All"
              # "Count"
              # "Tdelay"
              # "Probability"
              # "OnOff"
              # "Block"
              # "delayOpt"
              # "Count"
              # "Tdelay"
              # "Probability"
              # "OnOff"
              # "Block"
              # "Cue1 All"
              # "delayOpt"
              # "Count"
              # "Tdelay"
              # "Probability"
              # "OnOff"
              # "Block"
              # "Cue1 First"
              n1276 = call "myRIO_BRig_RT_dataLC_Cue1_delayOpt_Switch_l2.vi"() -> ("output_Cue1_delayOpt_Switch_l2"=w2130:i32)  [unwired: 11 in]
              n1277 = call "myRIO_BRig_RT_dataLC_Cue1_Block_Switch_l2.vi"() -> ("output_Cue1_Block_Switch_l2"=w2149:i32)  [unwired: 11 in]
              n1278 = call "myRIO_BRig_RT_dataLC_Cue1_OnOff_Switch_l2.vi"() -> ("output_Cue1_OnOff_Switch_l2"=w2147:i32)  [unwired: 11 in]
              n1279 = call "myRIO_BRig_RT_dataLC_Cue1_Probability_Switch_l2.vi"() -> ("output_Cue1_l2_First_Probability"=w2143:i32)  [unwired: 11 in]
              n1280 = call "myRIO_BRig_RT_dataLC_Cue1_Tdelay_Switch_l2.vi"() -> ("output_Cue1_Tdelay_Switch_l2"=w2141:i32)  [unwired: 11 in]
              n1281 = call "myRIO_BRig_RT_dataLC_Cue1_Count_Switch_l2.vi"() -> ("output_Cue1_Count_Switch_l2"=w2139:i32)  [unwired: 11 in]
              n1282 = local read "LC_Cue1_delayOpt_Switch_l2"() -> (w2129:bool)
              n1283 = call "myRIO_BRig_RT_dataLC_Cue1_Block_NS_l2.vi"() -> ("output_Cue1_Block_NS_l2"=w2127:i32)  [unwired: 11 in]
              n1284 = call "myRIO_BRig_RT_dataLC_Cue1_OnOff_NS_l2.vi"() -> ("output_Cue1_OnOff_NS_l2"=w2126:i32)  [unwired: 11 in]
              n1285 = call "myRIO_BRig_RT_dataLC_Cue1_Probability_NS_l2.vi"() -> ("output_Cue1_l2_All_Probability"=w2125:i32)  [unwired: 11 in]
              n1286 = call "myRIO_BRig_RT_dataLC_Cue1_Tdelay_NS_l2.vi"() -> ("output_Cue1_Tdelay_NS_l2"=w2124:i32)  [unwired: 11 in]
              n1287 = call "myRIO_BRig_RT_dataLC_Cue1_Count_NS_l2.vi"() -> ("output_Cue1_Count_NS_l2"=w2123:i32)  [unwired: 11 in]
              n1288 = call "myRIO_BRig_RT_dataLC_Cue1_delayOpt_NS_l2.vi"() -> ("output_Cue1_delayOpt_NS_l2"=w2122:i32)  [unwired: 11 in]
              n1289 = local read "LC_Cue1_Count_Switch_l2"() -> (w2138:u16)
              n1290 = local read "LC_Cue1_Probability_Switch_l2"() -> (w2142:u16)
              n1291 = local read "LC_Cue1_Block_Switch_l2"() -> (w2148:u16)
              n1292 = local read "LC_Cue1_Tdelay_Switch_l2"() -> (w2140:u16)
              n1293 = local read "LC_Cue1_OnOff_Switch_l2"() -> (w2146:bool)
              n1294 = local read "LC_Cue1_OnOff_NS_l2"() -> (w2118:bool)
              n1295 = call "myRIO_BRig_RT_dataLC_Selection_Block_NS_l2.vi"() -> ("output_Selection_Block_NS_l2"=w2103:i32)  [unwired: 11 in]
              n1296 = call "myRIO_BRig_RT_dataLC_Selection_OnOff_NS_l2.vi"() -> ("output_Selection_OnOff_NS_l2"=w2102:i32)  [unwired: 11 in]
              n1297 = call "myRIO_BRig_RT_dataLC_Selection_Probability_NS_l2.vi"() -> ("output_Selection_Probability_NS_l2"=w2101:i32)  [unwired: 11 in]
              n1298 = call "myRIO_BRig_RT_dataLC_Selection_Tdelay_NS_l2.vi"() -> ("output_Selection_Tdelay_NS_l2"=w2100:i32)  [unwired: 11 in]
              n1299 = call "myRIO_BRig_RT_dataLC_Selection_Count_NS_l2.vi"() -> ("output_Selection_Count_NS_l2"=w2099:i32)  [unwired: 11 in]
              n1300 = local read "LC_Cue1_delayOpt_NS_l2"() -> (w2119:bool)
              n1301 = local read "LC_Cue1_Probability_NS_l2"() -> (w2115:u16)
              n1302 = local read "LC_Cue1_Tdelay_NS_l2"() -> (w2114:u16)
              n1303 = local read "LC_Cue1_Count_NS_l2"() -> (w2113:u16)
              n1304 = local read "LC_Cue1_Block_NS_l2"() -> (w2117:u16)
              n1305 = local read "LC_Sel_Probability_NS_l2"() -> (w2107:u16)
              n1306 = local read "LC_Sel_Tdelay_NS_l2"() -> (w2106:u16)
              n1307 = local read "LC_Sel_OnOff_NS_l2"() -> (w2109:bool)
              n1308 = local read "LC_Sel_Count_NS_l2"() -> (w2105:u16)
              n1309 = local read "LC_Sel_Block_NS_l2"() -> (w2111:u16)
              n1310 = Boolean To (0,1)(Boolean=w2129) -> (0, 1=w2131:i16)
              n1311 = Boolean To (0,1)(Boolean=w2146) -> (0, 1=w2145:i16)
              n1312 = Boolean To (0,1)(Boolean=w2118) -> (0, 1=w2121:i16)
              n1313 = To Unsigned Word Integer(number=w2131) -> (unsigned 16bit integer=w2128:u16)
              n1314 = To Unsigned Word Integer(number=w2145) -> (unsigned 16bit integer=w2144:u16)
              n1315 = To Unsigned Word Integer(number=w2121) -> (unsigned 16bit integer=w2116:u16)
              n1316 = Boolean To (0,1)(Boolean=w2119) -> (0, 1=w2120:i16)
              n1317 = Boolean To (0,1)(Boolean=w2109) -> (0, 1=w2110:i16)
              n1318 = To Unsigned Word Integer(number=w2120) -> (unsigned 16bit integer=w2112:u16)
              n1319 = To Unsigned Word Integer(number=w2110) -> (unsigned 16bit integer=w2108:u16)
              n1320 = Replace Array Subset(array=w2150, new element #1=w2148, index #1=w2149, new element #2=w2144, index #2=w2147, new element #3=w2142, index #3=w2143, new element #4=w2140, index #4=w2141, new element #5=w2138, index #5=w2139, new element #6=w2128, index #6=w2130, new element #7=w2117, index #7=w2127, new element #8=w2116, index #8=w2126, new element #9=w2115, index #9=w2125, new element #10=w2114, index #10=w2124, new element #11=w2113, index #11=w2123, new element #12=w2112, index #12=w2122, new element #13=w2111, index #13=w2103, new element #14=w2108, index #14=w2102, new element #15=w2107, index #15=w2101, new element #16=w2106, index #16=w2100, new element #17=w2105, index #17=w2099) -> (w2151:u16[])
            }
            frame "saveSettings6_LC_l1_Other" {
              # "Trial"
              # "Tdelay"
              # "Probability"
              # "OnOff"
              # "Block"
              # "Wrong"
              # "Trial"
              # "Tdelay"
              # "Probability"
              # "OnOff"
              # "Block"
              # "Reward"
              n1321 = call "myRIO_BRig_RT_dataLC_Wrong_Block_l1.vi"() -> ("output_Wrong_Block_l1"=w2176:i32)  [unwired: 11 in]
              n1322 = call "myRIO_BRig_RT_dataLC_Wrong_OnOff_l1.vi"() -> ("output_Wrong_OnOff_l1"=w2175:i32)  [unwired: 11 in]
              n1323 = call "myRIO_BRig_RT_dataLC_Wrong_Probability_l1.vi"() -> ("output_Wrong_Probability_l1"=w2174:i32)  [unwired: 11 in]
              n1324 = call "myRIO_BRig_RT_dataLC_Wrong_Tdelay_l1.vi"() -> ("output_Wrong_Tdelay_l1"=w2173:i32)  [unwired: 11 in]
              n1325 = call "myRIO_BRig_RT_dataLC_Wrong_Trial_l1.vi"() -> ("output_Wrong_Trial_l1"=w2172:i32)  [unwired: 11 in]
              n1326 = call "myRIO_BRig_RT_dataLC_Reward_Block_l1.vi"() -> ("output_Reward_Block_l1"=w2188:i32)  [unwired: 11 in]
              n1327 = call "myRIO_BRig_RT_dataLC_Reward_OnOff_l1.vi"() -> ("output_Reward_OnOff_l1"=w2186:i32)  [unwired: 11 in]
              n1328 = call "myRIO_BRig_RT_dataLC_Reward_Probability_l1.vi"() -> ("output_Reward_Probability_l1"=w2182:i32)  [unwired: 11 in]
              n1329 = call "myRIO_BRig_RT_dataLC_Reward_Tdelay_l1.vi"() -> ("output_Reward_Tdelay_l1"=w2180:i32)  [unwired: 11 in]
              n1330 = call "myRIO_BRig_RT_dataLC_Reward_Trial_l1.vi"() -> ("output_Reward_Trial_l1"=w2178:i32)  [unwired: 11 in]
              n1331 = local read "LC_Wrong_OnOff_l1"() -> (w2170:bool)
              n1332 = local read "LC_Wrong_Probability_l1"() -> (w2167:u16)
              n1333 = local read "LC_Wrong_Block_l1"() -> (w2169:u16)
              n1334 = local read "LC_Wrong_Tdelay_l1"() -> (w2166:u16)
              n1335 = local read "LC_Wrong_Trial_l1"() -> (w2165:u16)
              n1336 = local read "LC_Reward_Probability_l1"() -> (w2181:u16)
              n1337 = local read "LC_Reward_Block_l1"() -> (w2187:u16)
              n1338 = local read "LC_Reward_Tdelay_l1"() -> (w2179:u16)
              n1339 = local read "LC_Reward_OnOff_l1"() -> (w2185:bool)
              n1340 = local read "LC_Reward_Trial_l1"() -> (w2177:u16)
              n1341 = Boolean To (0,1)(Boolean=w2170) -> (0, 1=w2171:i16)
              n1342 = Boolean To (0,1)(Boolean=w2185) -> (0, 1=w2184:i16)
              n1343 = To Unsigned Word Integer(number=w2171) -> (unsigned 16bit integer=w2168:u16)
              n1344 = To Unsigned Word Integer(number=w2184) -> (unsigned 16bit integer=w2183:u16)
              n1345 = Replace Array Subset(array=w2189, new element #1=w2187, index #1=w2188, new element #2=w2183, index #2=w2186, new element #3=w2181, index #3=w2182, new element #4=w2179, index #4=w2180, new element #5=w2177, index #5=w2178, new element #6=w2169, index #6=w2176, new element #7=w2168, index #7=w2175, new element #8=w2167, index #8=w2174, new element #9=w2166, index #9=w2173, new element #10=w2165, index #10=w2172) -> (w2190:u16[])
            }
            frame "SaveSettings6_LC_l2_Other" {
              # "Trial"
              # "Tdelay"
              # "Probability"
              # "OnOff"
              # "Block"
              # "Wrong"
              # "Trial"
              # "Tdelay"
              # "Probability"
              # "OnOff"
              # "Block"
              # "Reward"
              n1346 = call "myRIO_BRig_RT_dataLC_Wrong_Block_l2.vi"() -> ("output_Wrong_Block_l2"=w2199:i32)  [unwired: 11 in]
              n1347 = call "myRIO_BRig_RT_dataLC_Wrong_OnOff_l2.vi"() -> ("output_Wrong_OnOff_l2"=w2200:i32)  [unwired: 11 in]
              n1348 = call "myRIO_BRig_RT_dataLC_Wrong_Probability_l2.vi"() -> ("output_Wrong_Probability_l2"=w2201:i32)  [unwired: 11 in]
              n1349 = call "myRIO_BRig_RT_dataLC_Wrong_Tdelay_l2.vi"() -> ("output_Wrong_Tdelay_l2"=w2202:i32)  [unwired: 11 in]
              n1350 = call "myRIO_BRig_RT_dataLC_Wrong_Trial_l2.vi"() -> ("output_Wrong_Trial_l2"=w2203:i32)  [unwired: 11 in]
              n1351 = call "myRIO_BRig_RT_dataLC_Reward_Block_l2.vi"() -> ("output_Reward_Block_l2"=w2204:i32)  [unwired: 11 in]
              n1352 = call "myRIO_BRig_RT_dataLC_Reward_OnOff_l2.vi"() -> ("output_Reward_OnOff_l2"=w2205:i32)  [unwired: 11 in]
              n1353 = call "myRIO_BRig_RT_dataLC_Reward_Probability_l2.vi"() -> ("output_Reward_Probability_l2"=w2206:i32)  [unwired: 11 in]
              n1354 = call "myRIO_BRig_RT_dataLC_Reward_Tdelay_l2.vi"() -> ("output_Reward_Tdelay_l2"=w2207:i32)  [unwired: 11 in]
              n1355 = call "myRIO_BRig_RT_dataLC_Reward_Trial_l2.vi"() -> ("output_Reward_Trial_l2"=w2208:i32)  [unwired: 11 in]
              n1356 = local read "LC_Wrong_OnOff_l2"() -> (w2220:bool)
              n1357 = local read "LC_Wrong_Probability_l2"() -> (w2217:u16)
              n1358 = local read "LC_Wrong_Block_l2"() -> (w2219:u16)
              n1359 = local read "LC_Wrong_Tdelay_l2"() -> (w2216:u16)
              n1360 = local read "LC_Wrong_Trial_l2"() -> (w2215:u16)
              n1361 = local read "LC_Reward_Probability_l2"() -> (w2224:u16)
              n1362 = local read "LC_Reward_Block_l2"() -> (w2228:u16)
              n1363 = local read "LC_Reward_Tdelay_l2"() -> (w2223:u16)
              n1364 = local read "LC_Reward_OnOff_l2"() -> (w2227:bool)
              n1365 = local read "LC_Reward_Trial_l2"() -> (w2222:u16)
              n1366 = Boolean To (0,1)(Boolean=w2220) -> (0, 1=w2221:i16)
              n1367 = Boolean To (0,1)(Boolean=w2227) -> (0, 1=w2226:i16)
              n1368 = To Unsigned Word Integer(number=w2221) -> (unsigned 16bit integer=w2218:u16)
              n1369 = To Unsigned Word Integer(number=w2226) -> (unsigned 16bit integer=w2225:u16)
              n1370 = Replace Array Subset(array=w2229, new element #1=w2228, index #1=w2204, new element #2=w2225, index #2=w2205, new element #3=w2224, index #3=w2206, new element #4=w2223, index #4=w2207, new element #5=w2222, index #5=w2208, new element #6=w2219, index #6=w2199, new element #7=w2218, index #7=w2200, new element #8=w2217, index #8=w2201, new element #9=w2216, index #9=w2202, new element #10=w2215, index #10=w2203) -> (w2230:u16[])
            }
            frame "setSettings_Audio" {
              # "amp_L"
              # "amp_R"
              # "freq_L"
              # "freq_R"
              n1371 = call "myRIO_BRig_RT_dataExp_Audio_amp__L.vi"() -> ("output_Audio_amp__L"=w2258:i32)  [unwired: 11 in]
              n1372 = call "myRIO_BRig_RT_dataExp_Audio_amp__R.vi"() -> ("output_Audio_amp__R"=w2257:i32)  [unwired: 11 in]
              n1373 = call "myRIO_BRig_RT_dataExp_Audio_freq__L.vi"() -> ("output_Audio_freq__L"=w2256:i32)  [unwired: 11 in]
              n1374 = call "myRIO_BRig_RT_dataExp_Audio_freq__R.vi"() -> ("output_Audio_freq__R"=w2255:i32)  [unwired: 11 in]
              n1375 = Index Array(array=w2254, index #1=w2258, index #2=w2257, index #3=w2256, index #4=w2255) -> (element #1=w2243:u16, element #2=w2242:u16, element #3=w2247:u16, element #4=w2246:u16)
              n1376 = To Unsigned Byte Integer(number=w2247) -> (unsigned 8bit integer=w2241:u8)
              n1377 = To Unsigned Byte Integer(number=w2246) -> (unsigned 8bit integer=w2240:u8)
              n1378 = xnode "Read/Write Control"("FPGA VI Reference In"=w2245, "error in"=w2244, "audioAmp_L"=w2243, "audioAmp_R"=w2242, "audioFreq_L_kHz"=w2241, "audioFreq_R_kHz"=w2240) -> ("error out"=w2239:errorcluster)  [unwired: 1 out]
              n1379 = local write "error out"(w2239) -> ()
            }
            frame "setSettings_Laser" {
              w2289 = u32 0 ("laser2_selRew_Ndelay")
              # "tDelay"
              # "Wrong l1"
              # "Reward l1"
              n1380 = call "myRIO_BRig_RT_dataExp_IallReward.vi"() -> ("output_I_allReward"=w2270:i32)  [unwired: 11 in]
              n1381 = local read "Laser_Tpeak_l1"() -> (w2300:dbl)
              n1382 = local read "Laser_Tshutter_l1"() -> (w2298:dbl)
              n1383 = local read "Laser_Freq_l1"() -> (w2299:dbl)
              n1384 = local read "Laser_duration_l1"() -> (w2274:u16)
              n1385 = local read "Laser_Tpeak_l2"() -> (w2296:dbl)
              n1386 = local read "Laser_Tshutter_l2"() -> (w2294:dbl)
              n1387 = local read "Laser_Freq_l2"() -> (w2295:dbl)
              n1388 = local read "Laser_duration_l2"() -> (w2273:u16)
              n1389 = local read "CueLed_Freq"() -> (w2283:dbl)
              n1390 = local read "CueLed_Tpeak"() -> (w2284:dbl)
              n1391 = local read "I_allReward"() -> (w2269:bool)
              n1392 = call "myRIO_BRig_RT_dataLC_Reward_Tdelay_l1.vi"() -> ("output_Reward_Tdelay_l1"=w2312:i32)  [unwired: 11 in]
              n1393 = call "myRIO_BRig_RT_dataLC_Wrong_Tdelay_l1.vi"() -> ("output_Wrong_Tdelay_l1"=w2313:i32)  [unwired: 11 in]
              n1394 = local read "FPGA_count2ms"() -> (w2285:dbl)
              n1395 = Index Array(array=w2280, index #1=w2312, index #2=w2313) -> (element #1=w2311:u16, element #2=w2310:u16)
              n1396 = To Double Precision Float(number=w2311) -> (double precision float=w2307:dbl)
              n1397 = To Double Precision Float(number=w2310) -> (double precision float=w2304:dbl)
              n1398 = Boolean To (0,1)(Boolean=w2269) -> (0, 1=w2268:i16)
              n1399 = To Unsigned Word Integer(number=w2268) -> (unsigned 16bit integer=w2267:u16)
              n1400 = Replace Array Subset(array=w2272, new element=w2267, index=w2270) -> (w2271:u16[])
              n1401 = To Unsigned Word Integer(number=w2285) -> (unsigned 16bit integer=w2301:u16)
              n1402 = call "myRIO_BRig_RT__calc_laser_FPGA_N.vi"("input_FPGA_ms2count"=w2285, "input_Tpeak"=w2300, "input_Freq"=w2299, "input_Tshutter"=w2298, "input_duration"=w2274) -> ("output_laser_Npeak"=w2288:u32, "output_laser_Nvalley"=w2287:u32, "output_laser_Nshutter"=w2286:u32, "output_laser_Nduration"=w2297:u32, "output_laser_Tduration"=w2278:u16)  [unwired: 6 in]
              n1403 = Multiply(x=w2285, y=w2307) -> (x*y=w2308:dbl)
              n1404 = Multiply(x=w2285, y=w2304) -> (x*y=w2305:dbl)
              n1405 = call "myRIO_BRig_RT__calc_laser_FPGA_N__CueLed.vi"("input_FPGA_ms2count"=w2285, "input_Tpeak"=w2284, "input_Freq"=w2283) -> ("output_laser_Npeak"=w2282:u32, "output_laser_Nvalley"=w2281:u32)  [unwired: 11 in]
              n1406 = call "myRIO_BRig_RT__calc_laser_FPGA_N.vi"("input_FPGA_ms2count"=w2285, "input_Tpeak"=w2296, "input_Freq"=w2295, "input_Tshutter"=w2294, "input_duration"=w2273) -> ("output_laser_Npeak"=w2293:u32, "output_laser_Nvalley"=w2292:u32, "output_laser_Nshutter"=w2291:u32, "output_laser_Nduration"=w2290:u32, "output_laser_Tduration"=w2277:u16)  [unwired: 6 in]
              n1407 = Round Toward +Infinity(x=w2308) -> (ceil(x): smallest int >= x=w2309:dbl)
              n1408 = Round Toward +Infinity(x=w2305) -> (ceil(x): smallest int >= x=w2306:dbl)
              n1409 = To Unsigned Long Integer(number=w2309) -> (unsigned 32bit integer=w2303:u32)
              n1410 = To Unsigned Long Integer(number=w2306) -> (unsigned 32bit integer=w2302:u32)
              n1411 = xnode "Read/Write Control"("FPGA VI Reference In"=w2314, "error in"=w2315, "I_allReward"=w2269, "LC_nPeak_l1"=w2288, "LC_nValley_l1"=w2287, "LC_nShutter_l1"=w2286, "LR_reward_nDelay_l1"=w2303, "LR_wrong_nDelay_l1"=w2302, "LR_reward_nTotal_l1"=w2297, "LR_wrong_nTotal_l1"=w2297, "k1__counter_per_ms"=w2301, "LC_nPeak_l2"=w2293, "LC_nValley_l2"=w2292, "LC_nShutter_l2"=w2291, "LR_reward_nDelay_l2"=w2289, "LR_wrong_nDelay_l2"=w2289, "LR_reward_nTotal_l2"=w2290, "LR_wrong_nTotal_l2"=w2290, "CueLed_nPeak"=w2282, "CueLed_nValley"=w2281) -> ("error out"=→"error out":errorcluster)  [unwired: 1 out]
              n1412 = call "myRIO_BRig_RT_dataCurrent_laser1_pulse_duration.vi"() -> ("output_laser1_pulse_duration"=w2276:i32)  [unwired: 11 in]
              n1413 = call "myRIO_BRig_RT_dataCurrent_laser2_pulse_duration.vi"() -> ("output_laser2_pulse_duration"=w2275:i32)  [unwired: 11 in]
              n1414 = Replace Array Subset(array=w2280, new element #1=w2278, index #1=w2276, new element #2=w2277, index #2=w2275) -> (w2279:u16[])
            }
            frame "initBlock" {
              n1415 = local write "nRewards_cur"(u16 0 ("nRewards_cur")) -> ()
              n1416 = call "myRIO_Brig_RT__Case_Exp_State_initBlock__v2.vi"("input_spout"=w2336, "input_dataCurrent"=w2342, "input_dataExp"=w2339, "input_dataBlock"=w2331) -> ("output_state"=w2335:T2, "output_spout"=w2334:enum16{"Left", "Right"}, "idxDataBlock"=w2337:i32, "output_dataCurrent"=w2341:u16[], "output_dataExp"=w2340:u16[], "output_TpB_target"=→"TpB_target":u16, "output_iBlock"=w2332:u16, "output_dataBlock"=w2330:u16[][])  [unwired: 4 in]
              "iBlock" <- w2332
              "cSpout" <- w2334
            }
            frame "initBlock2" {
              n1417 = call "myRIO_BRig_RT__Case_Exp_State_initBlock2.vi"("input_spout"=w2359, "input_dataBlock"=w2360, "input_dataCurrent"=w2358) -> ("idxDataBlock"=w2355:i32, "output_dataBlock"=w2357:u16[][])  [unwired: 7 in]
            }
            frame "initTrial" {
              n1418 = xnode "Read/Write Control"("FPGA VI Reference In"=w2375, "error in"=w2374, "SelectionState"=FALSE) -> ("error out"=w2373:errorcluster)  [unwired: 1 out]
              n1419 = call "myRIO_Brig_RT__Case_Exp_State_initTrial__v2.vi"("input_spout"=w2376, "input_dataBlock"=w2371, "input_dataExp"=w2387, "input_dataCurrent"=w2388) -> ("output_state"=w2389:T2, "output_dataExp"=w2386:u16[], "output_dataCurrent"=w2381:u16[], "output_iTrial"=w2370:u16, "output_SolenoidReward"=→"SolenoidReward":bool)  [unwired: 3 in]
              "iTrial" <- w2370
              n1420 = local write "error out"(w2373) -> ()
            }
            frame "initTrial2" {
              # "trialUntilReward"
              n1421 = call "myRIO_BRig_RT__Case_Exp_subState_LC__initTrial__v4.vi"("input_dataCurrent"=w2395, "input_dataExp"=w2393, "input_dataLC"=w2405, "input_spout"=w2406, "input_dataTrial"=w2408) -> ("output_dataTrial"=w2407:u16[][], "output_LR_Wrong_Laser_l2"=w2397:bool, "output_dataCurrent"=w2394:u16[], "output_LR_Reward_Laser_l2"=w2398:bool, "output_LR_Reward_Event_l1"=w2404:bool, "output_LR_Wrong_Event_l1"=w2403:bool, "output_LR_Reward_Laser_l1"=w2402:bool, "output_LR_Wrong_Laser_l1"=w2401:bool, "output_LR_Reward_Event_l2"=w2400:bool, "output_LR_Wrong_Event_l2"=w2399:bool)  [unwired: 5 in]
              n1422 = call "myRIO_BRig_RT_dataExp_ItrialUntilReward.vi"() -> ("output_I_trialUntilReward"=w2412:i32)  [unwired: 11 in]
              n1423 = Index Array(array=w2393, index=w2412) -> (element=w2411:u16)
              n1424 = Equal?(x=w2406, y=enum16{"Left", "Right"}."Right") -> (x = y?=w2410:bool)
              n1425 = Not Equal To 0?(x=w2411) -> (x != 0?=w2409:bool)
              n1426 = xnode "Read/Write Control"("FPGA VI Reference In"=w2422, "error in"=w2421, "Left(F)_or_Right(T)"=w2410, "ignoreWrong"=w2409, "LR_reward_Event_l1"=w2404, "LR_wrong_Event_l1"=w2403, "LR_reward_Laser_l1"=w2402, "LR_wrong_Laser_l1"=w2401, "LR_reward_Event_l2"=w2400, "LR_wrong_Event_l2"=w2399, "LR_reward_Laser_l2"=w2398, "LR_wrong_laser_l2"=w2397) -> ("error out"=w2396:errorcluster)  [unwired: 1 out]
              n1427 = local write "error out"(w2396) -> ()
            }
            frame "initTrial3" {
              # "Cue1_CueType"
              n1428 = call "myRIO_BRig_RT_dataExp_CueLed.vi"() -> ("output_CueLed"=w2431:i32)  [unwired: 11 in]
              n1429 = call "myRIO_BRig_RT_arrTrig_init.vi"() -> ("output_arrTrig"=w2435:bool[])  [unwired: 11 in]
              n1430 = Index Array(array=w2432, index=w2431) -> (element=w2430:u16)
              n1431 = call "myRIO_BRig_RT_arrTrig_Cue1_CueType_AudioLed.vi"() -> ("output_arrTrig_Cue1_CueType_AudioLed"=w2433:i32)  [unwired: 11 in]
              n1432 = Not Equal To 0?(x=w2430) -> (x != 0?=w2429:bool)
              n1433 = call "myRIO_BRig_RT__Case_Exp_State_initTrial_dataTrial.vi"("input_spout"=w2448, "input_dataCurrent"=w2437, "input_dataExp"=w2432, "input_dataTrial"=w2450) -> ("output_laserPower_l2"=w2438:u16, "output_dataCurrent"=w2436:u16[], "output_dataTrial"=w2449:u16[][], "output_laserPower_l1"=w2445:u16)  [unwired: 4 in]
              n1434 = To Double Precision Float(number=w2445) -> (double precision float=w2447:dbl)
              n1435 = To Double Precision Float(number=w2438) -> (double precision float=w2441:dbl)
              n1436 = Replace Array Subset(array=w2435, new element=w2429, index=w2433) -> (w2434:bool[])
              n1437 = Divide(x=w2447, y=100.0 ("x")) -> (x/y=w2442:dbl)
              "power_l1" <- w2442
              n1438 = Divide(x=w2441, y=100.0 ("x")) -> (x/y=w2439:dbl)
              "power_l2" <- w2439
              n1439 = call "myRIO__convert__Voltage_to_FPGAvalue.vi"("input_voltage"=w2442) -> ("output_PortC"=w2427:i16)  [unwired: 9 in, 1 out]
              n1440 = call "myRIO__convert__Voltage_to_FPGAvalue.vi"("input_voltage"=w2439) -> ("output_PortC"=w2426:i16)  [unwired: 9 in, 1 out]
              n1441 = xnode "Read/Write Control"("FPGA VI Reference In"=w2444, "error in"=w2443, "AnaOut_0"=w2427, "AnaOut_1"=w2426) -> ("error out"=w2428:errorcluster)  [unwired: 1 out]
              n1442 = local write "error out"(w2428) -> ()
            }
            frame "initTrial4" {
              n1443 = call "myRIO_BRig_RT_dataTrial_activeRecording.vi"() -> ("output_activeRecording"=w2470:i32)  [unwired: 11 in]
              n1444 = call "myRIO_BRig_RT_dataCurrent_idxDataTrial.vi"() -> ("output_idxDataTrial"=w2473:i32)  [unwired: 11 in]
              n1445 = Index Array(array=w2475, index=w2473) -> (element=w2472:u16)
              n1446 = xnode "Read/Write Control"("FPGA VI Reference In"=w2465, "error in"=w2464, "A6_Act"="Recording") -> ("error out"=w2462:errorcluster)  [unwired: 1 out]
              n1447 = Boolean To (0,1)(Boolean="Recording") -> (0, 1=w2469:i16)
              n1448 = To Long Integer(number=w2472) -> (32bit integer=w2471:i32)
              n1449 = To Unsigned Word Integer(number=w2469) -> (unsigned 16bit integer=w2468:u16)
              n1450 = local write "error out"(w2462) -> ()
              n1451 = Replace Array Subset(array=w2474, new element=w2468, index (row)=w2471, index (col)=w2470) -> (w2467:u16[][])
            }
            frame "initTrial_LC_ENL1" {
              n1452 = call "myRIO_BRig_RT__Case_Exp_State_initTrial_LC_ENL1__v4.vi"("input_dataTrial"=w2494, "input_spout"=w2497, "input_arrTrig"=w2491, "input_dataBlock"=w2492, "input_dataLC"=w2498, "input_dataCurrent"=w2496) -> ("output_arrTrig"=w2490:bool[], "output_dataTrial"=w2493:u16[][], "output_dataCurrent"=w2495:u16[])  [unwired: 3 in]
            }
            frame "initTrial_LC_Cue1" {
              n1453 = call "myRIO_BRig_RT__Case_Exp_State_initTrial_LC_Cue1__v4.vi"("input_dataTrial"=w2513, "input_spout"=w2516, "input_arrTrig"=w2510, "input_dataBlock"=w2511, "input_dataLC"=w2517, "input_dataCurrent"=w2515) -> ("output_arrTrig"=w2509:bool[], "output_dataTrial"=w2512:u16[][], "output_dataCurrent"=w2514:u16[])  [unwired: 3 in]
            }
            frame "initTrial_LC_Sel" {
              n1454 = xnode "Read/Write Control"("FPGA VI Reference In"=w2530, "error in"=w2529, "A6_Act"=FALSE) -> ("error out"=w2531:errorcluster)  [unwired: 1 out]
              n1455 = local write "error out"(w2531) -> ()
              n1456 = call "myRIO_BRig_RT__Case_Exp_State_initTrial_LC_Sel__v4.vi"("input_dataTrial"=w2536, "input_spout"=w2539, "input_arrTrig"=w2533, "input_dataBlock"=w2534, "input_dataLC"=w2540, "input_dataCurrent"=w2538) -> ("output_arrTrig"=w2532:bool[], "output_dataTrial"=w2535:u16[][], "output_dataCurrent"=w2537:u16[])  [unwired: 3 in]
            }
            frame "ENL1_pre" {
              n1457 = call "myRIO_BRig_RT__Case_Exp_State_Enl1Pre__v3.vi"("input_I_lick"=w2554, "input_arrTrig"=w2551, "input_dataCurrent"=w2555) -> ("output_dataCurrent"=w2552:u16[], "output_state"=w2553:T2)  [unwired: 3 in, 4 out]
            }
            frame "ENL1" {
              n1458 = call "myRIO_BRig_RT__Case_Exp_State_ENL1__v3.vi"("I_lick"=w2574, "input_arrTrig"=w2572, "input_state"=w2578, "input_dataCurrent"=w2577) -> ("output_l1_laserOn"=w2570:bool, "output_l1_laserEvent"=w2571:bool, "output_state"=w2575:T2, "output_dataCurrent"=w2576:u16[], "output_l2_laserEvent"=w2569:bool, "output_l2_laserOn"=w2568:bool)  [unwired: 2 in]
            }
            frame "ENL1Penalty_pre" {
              # "Tcycle"
              # "counter"
              n1459 = call "myRIO_BRig_RT_dataCurrent_Tcycle_generic.vi"() -> ("output_Tcycle_generic"=w2605:i32)  [unwired: 11 in]
              n1460 = call "myRIO_BRig_RT_dataCurrent_count_generic.vi"() -> ("output_count_generic"=w2607:i32)  [unwired: 11 in]
              n1461 = call "myRIO_BRig_RT_dataExp_ENL_penalty.vi"() -> ("output_ENL_penalty"=w2600:i32)  [unwired: 11 in]
              n1462 = Index Array(array=w2601, index=w2600) -> (element=w2604:u16)
              n1463 = Replace Array Subset(array=w2602, new element #1=u16 0 ("new element/subarray"), index #1=w2607, new element #2=w2604, index #2=w2605) -> (w2603:u16[])
            }
            frame "ENL1Penalty" {
              n1464 = call "myRIO_BRig_RT__Case_Exp_State_ENL1Penalty.vi"("input_state"=w2621, "input_dataCurrent"=w2625) -> ("output_state"=w2622:T2, "output_dataCurrent"=w2624:u16[])  [unwired: 8 in]
            }
            frame "ENL2_pre" {
            }
            frame "ENL2" {
            }
            frame "ENL2Penalty_pre" {
            }
            frame "ENL2Penalty" {
            }
            frame "Cue1_pre" {
              n1465 = call "myRIO_BRig_RT__Case_Exp_State_Cue1Pre__v3.vi"("input_dataCurrent"=w2697, "input_dataExp"=w2693, "input_arrTrig"=w2690, "input_spout"=w2694) -> ("output_audioR"=w2691:bool, "output_audioL"=w2692:bool, "output_state"=w2695:T2, "output_dataCurrent"=w2696:u16[])  [unwired: 7 in, 5 out]
            }
            frame "Cue1" {
              n1466 = call "myRIO_BRig_RT__Case_Exp_State_Cue1__v4.vi"("input_state"=w2718, "input_dataCurrent"=w2719, "I_lick"=w2717, "input_arrTrig"=w2720) -> ("output_SelectionState"=w2711:bool, "output_CueLed_Event"=w2716:bool, "output_state"=w2712:T2, "output_dataCurrent"=w2713:u16[], "output_l1_laserEvent"=w2709:bool, "output_l1_laserOn"=w2710:bool, "output_l2_laserEvent"=w2714:bool, "output_l2_laserOn"=w2715:bool)  [unwired: 8 in]
              n1467 = xnode "Read/Write Control"("FPGA VI Reference In"=w2723, "error in"=w2722, "SelectionState"=w2711) -> ()  [unwired: 2 out]
            }
            frame "Cue1Penalty_pre" {
              # "Tcycle"
              # "counter"
              n1468 = call "myRIO_BRig_RT_dataCurrent_Tcycle_generic.vi"() -> ("output_Tcycle_generic"=w2759:i32)  [unwired: 11 in]
              n1469 = call "myRIO_BRig_RT_dataCurrent_count_generic.vi"() -> ("output_count_generic"=w2761:i32)  [unwired: 11 in]
              n1470 = call "myRIO_BRig_RT_dataExp_CueLed.vi"() -> ("output_CueLed"=w2743:i32)  [unwired: 11 in]
              n1471 = call "myRIO_BRig_RT_dataExp_Tcycle_Cue1Penalty_Audio.vi"() -> ("output_Tcycle_Cue1Penalty_Audio"=w2744:i32)  [unwired: 11 in]
              n1472 = call "myRIO_BRig_RT_dataExp_Tcycle_Cue1Penalty_LED.vi"() -> ("output_Tcycle_Cue1Penalty_LED"=w2742:i32)  [unwired: 11 in]
              n1473 = Index Array(array=w2755, index #1=w2743, index #2=w2744, index #3=w2742) -> (element #1=w2741:u16, element #2=w2739:u16, element #3=w2738:u16)
              n1474 = Equal To 0?(x=w2741) -> (x = 0?=w2740:bool)
              n1475 = Select(t=w2739, s=w2740, f=w2738) -> (s? t:f=w2737:u16)
              n1476 = Replace Array Subset(array=w2757, new element #1=u16 0 ("new element/subarray"), index #1=w2761, new element #2=w2737, index #2=w2759) -> (w2756:u16[])
            }
            frame "Cue1Penalty" {
              n1477 = call "myRIO_BRig_RT__Case_Exp_State_Cue1Penalty.vi"("input_state"=w2778, "input_dataCurrent"=w2779) -> ("output_state"=w2776:T2, "output_dataCurrent"=w2777:u16[])  [unwired: 8 in]
            }
            frame "Cue2_pre" {
            }
            frame "Cue2" {
            }
            frame "Cue2Penalty_pre" {
            }
            frame "Cue2Penalty" {
            }
            frame "Selection_pre" {
              n1478 = xnode "Read/Write Control"("FPGA VI Reference In"=w2857, "error in"=w2858) -> ("error out"=w2845:errorcluster, "SelectReward"=w2852:bool, "SelectWrong"=w2853:bool)  [unwired: 1 out]
              n1479 = local write "error out"(w2845) -> ()
              n1480 = call "myRIO_BRig_RT__Case_Exp_State_SelectPre__v5.vi"("input_dataCurrent"=w2856, "input_SelectWrong"=w2853, "input_SelectReward"=w2852, "input_dataExp"=w2846, "input_LickL"=w2844, "input_LickR"=w2843, "input_arrTrig"=w2851) -> ("output_state"=w2854:T2, "output_dataCurrent"=w2855:u16[], "output_l1_laserEvent"=w2850:bool, "output_l1_laserOn"=w2849:bool, "output_l2_laserOn"=w2847:bool, "output_l2_laserEvent"=w2848:bool)  [unwired: 3 in]
            }
            frame "Selection" {
              n1481 = xnode "Read/Write Control"("FPGA VI Reference In"=w2885, "error in"=w2884) -> ("error out"=w2872:errorcluster, "SelectReward"=w2879:bool, "SelectWrong"=w2878:bool)  [unwired: 1 out]
              n1482 = local write "error out"(w2872) -> ()
              n1483 = call "myRIO_BRig_RT__Case_Exp_State_Selection__v5.vi"("input_dataCurrent"=w2883, "input_state"=w2881, "input_dataExp"=w2871, "input_LickL"=w2870, "input_FPGA_SelectReward"=w2879, "input_FPGA_SelectWrong"=w2878, "input_LickR"=w2869, "input_arrTrig"=w2877) -> ("output_state"=w2880:T2, "output_dataCurrent"=w2882:u16[], "output_LC_Event_l1"=w2876:bool, "output_LC_Laser_l2"=w2873:bool, "output_LC_Event_l2"=w2874:bool, "output_LC_Laser_l1"=w2875:bool)  [unwired: 2 in]
            }
            frame "SelectReward_pre" {
              # "iState"
              # "nRewTrials"
              # "Tcycle\nGeneric"
              # "counter"
              n1484 = call "myRIO_BRig_RT_dataCurrent_nRewTrials.vi"() -> ("output_nRewTrials"=w2909:i32)  [unwired: 11 in]
              n1485 = call "myRIO_BRig_RT_dataCurrent_Tcycle_reward.vi"() -> ("output_Tcycle_reward"=w2898:i32)  [unwired: 11 in]
              n1486 = Index Array(array=w2896, index #1=w2909, index #2=w2898) -> (element #1=w2908:u16, element #2=w2897:u16)
              n1487 = Increment(x=w2908) -> (x+1=w2907:u16)
              n1488 = call "myRIO_BRig_RT__Case_Exp_subState_LC__Reward.vi"("input_spout"=w2916, "input_dataCurrent"=w2896, "input_dataLC"=w2915) -> ()  [unwired: 6 in, 2 out]
              n1489 = call "myRIO_BRig_RT_dataCurrent_count_generic.vi"() -> ("output_count_generic"=w2911:i32)  [unwired: 11 in]
              n1490 = call "myRIO_BRig_RT_dataCurrent_Tcycle_generic.vi"() -> ("output_Tcycle_generic"=w2912:i32)  [unwired: 11 in]
              n1491 = call "myRIO_BRig_RT_dataCurrent_iState.vi"() -> ("output_iState"=w2906:i32)  [unwired: 11 in]
              n1492 = Replace Array Subset(array=w2896, new element #1=w2907, index #1=w2909, new element #2=u16 0 ("new element/subarray"), index #2=w2911, new element #3=w2897, index #3=w2912, new element #4=u16 1 ("new element/subarray"), index #4=w2906) -> (w2918:u16[])
            }
            frame "SelectReward" {
              n1493 = call "myRIO_BRig_RT__Case_Exp_State_Reward__v2.vi"("input_dataCurrent"=w2936, "input_state"=w2933, "input_spout"=w2931, "input_dataExp"=w2923, "input_dataTrial"=w2922) -> ("output_dataCurrent"=w2935:u16[], "output_state"=w2934:T2, "output__L"=w2929:bool, "output__R"=w2930:bool)  [unwired: 7 in]
            }
            frame "SelectRewardPost_pre" {
              # "nRewards"
              # "nRewTrials"
              # "Tcycle"
              # "counter"
              n1494 = call "myRIO_BRig_RT_dataBlock_nRewards__L.vi"() -> ("output_nRewards__L"=w2951:i32)  [unwired: 11 in]
              n1495 = call "myRIO_BRig_RT_dataBlock_nRewards__R.vi"() -> ("output_nRewards__R"=w2950:i32)  [unwired: 11 in]
              n1496 = call "myRIO_BRig_RT_dataCurrent_Tcycle_generic.vi"() -> ("output_Tcycle_generic"=w2966:i32)  [unwired: 11 in]
              n1497 = call "myRIO_BRig_RT_dataCurrent_count_generic.vi"() -> ("output_count_generic"=w2968:i32)  [unwired: 11 in]
              n1498 = case shown="\"Left\", Default" w2944 {
                tunnel: w2956 -> [w2973 w2977]
                tunnel: [w2972 w2977] -> w2955
                tunnel: [w2974 w2975] -> w2954
                tunnel: w2953 -> [w2974 w2976]
                frame "Left", Default {
                  n1499 = Increment(x=w2973) -> (x+1=w2972:u16)
                }
                frame "Right" {
                  n1500 = Increment(x=w2976) -> (x+1=w2975:u16)
                }
              }
              "nRewards_Left" <- w2955
              "nRewards_Right" <- w2954
              n1501 = Equal?(x=w2944, y=enum16{"Left", "Right"}."Left") -> (x = y?=w2943:bool)
              n1502 = Select(t=w2951, s=w2943, f=w2950) -> (s? t:f=w2949:i32)
              n1503 = call "myRIO_BRig_RT_dataExp_Tcycle_RewardPost.vi"() -> ("output_Tcycle_RewardPost"=w2962:i32)  [unwired: 11 in]
              n1504 = call "myRIO_BRig_RT_dataCurrent_nRewTrials.vi"() -> ("output_nRewTrials"=w2952:i32)  [unwired: 11 in]
              n1505 = Index Array(array=w2963, index=w2962) -> (element=w2965:u16)
              n1506 = Index Array(array=w2946, index=w2952) -> (element=w2941:u16)
              n1507 = Replace Array Subset(array=w2946, new element #1=u16 0 ("new element/subarray"), index #1=w2968, new element #2=w2965, index #2=w2966) -> (w2964:u16[])
              n1508 = Replace Array Subset(array=w2948, new element=w2941, index (row)=w2942, index (col)=w2949) -> (w2947:u16[][])
              n1509 = local write "nRewards_cur"(w2941) -> ()
            }
            frame "SelectRewardPost" {
              n1510 = call "myRIO_BRig_RT__Case_Exp_State_RewardPost.vi"("input_state"=w2988, "input_dataCurrent"=w2991) -> ("output_state"=w2989:T2, "output_dataCurrent"=w2990:u16[])  [unwired: 8 in]
            }
            frame "SelectWrong_pre" {
              # "iState"
              # "Tcycle"
              # "counter"
              n1511 = call "myRIO_BRig_RT_dataCurrent_Tcycle_generic.vi"() -> ("output_Tcycle_generic"=w3012:i32)  [unwired: 11 in]
              n1512 = call "myRIO_BRig_RT_dataCurrent_count_generic.vi"() -> ("output_count_generic"=w3014:i32)  [unwired: 11 in]
              n1513 = call "myRIO_BRig_RT_dataExp_Tcycle_Wrong.vi"() -> ("output_Tcycle_Wrong"=w3010:i32)  [unwired: 11 in]
              n1514 = call "myRIO_BRig_RT__Case_Exp_subState_LC__Wrong.vi"("input_spout"=w3006, "input_dataCurrent"=w3007, "input_dataLC"=w3004) -> ()  [unwired: 6 in, 2 out]
              n1515 = Index Array(array=w3008, index=w3010) -> (element=w3011:u16)
              n1516 = call "myRIO_BRig_RT_dataCurrent_iState.vi"() -> ("output_iState"=w3002:i32)  [unwired: 11 in]
              n1517 = Replace Array Subset(array=w3007, new element #1=u16 0 ("new element/subarray"), index #1=w3014, new element #2=w3011, index #2=w3012, new element #3=u16 2 ("new element/subarray"), index #3=w3002) -> (w3009:u16[])
            }
            frame "SelectWrong" {
              n1518 = call "myRIO_BRig_RT__Case_Exp_State_Wrong.vi"("input_state"=w3028, "input_dataCurrent"=w3033) -> ("output_state"=w3025:T2, "output_dataCurrent"=w3032:u16[])  [unwired: 8 in]
              n1519 = Not Equal?(x=w3028, y=w3025) -> (x != y?=w3027:bool)
              n1520 = Select(t=myRIO_BRig_RT__Case_Exp_stateList."SelectWrong_post" ("Enum"), s=w3027, f=w3025) -> (s? t:f=w3024:T2)
            }
            frame "SelectWrong_post" {
            }
            frame "SelectTimeout_pre" {
              # "iState"
              # "Tcycle"
              # "counter"
              n1521 = xnode "Read/Write Control"("FPGA VI Reference In"=w3056, "error in"=w3055, "SelectionState"=FALSE) -> ("error out"=w3053:errorcluster)  [unwired: 1 out]
              n1522 = call "myRIO_BRig_RT_dataCurrent_Tcycle_generic.vi"() -> ("output_Tcycle_generic"=w3074:i32)  [unwired: 11 in]
              n1523 = call "myRIO_BRig_RT_dataCurrent_count_generic.vi"() -> ("output_count_generic"=w3072:i32)  [unwired: 11 in]
              n1524 = call "myRIO_BRig_RT_dataExp_Tcycle_Timeout.vi"() -> ("output_Tcycle_Timeout"=w3076:i32)  [unwired: 11 in]
              n1525 = local write "error out"(w3053) -> ()
              n1526 = call "myRIO_BRig_RT__Case_Exp_subState_LC__Timeout.vi"("input_spout"=w3067, "input_dataCurrent"=w3068, "input_dataLC"=w3066) -> ()  [unwired: 6 in, 2 out]
              n1527 = Index Array(array=w3070, index=w3076) -> (element=w3075:u16)
              n1528 = call "myRIO_BRig_RT_dataCurrent_iState.vi"() -> ("output_iState"=w3064:i32)  [unwired: 11 in]
              n1529 = Replace Array Subset(array=w3068, new element #1=u16 0 ("new element/subarray"), index #1=w3072, new element #2=w3075, index #2=w3074, new element #3=u16 3 ("new element/subarray"), index #3=w3064) -> (w3071:u16[])
            }
            frame "SelectTimeout" {
              n1530 = call "myRIO_BRig_RT__Case_Exp_State_Timeout.vi"("input_dataLC"=w3091, "input_state"=w3086, "input_dataCurrent"=w3096) -> ("output_state"=w3087:T2, "output_dataCurrent"=w3095:u16[])  [unwired: 6 in, 1 out]
              n1531 = Not Equal?(x=w3086, y=w3087) -> (x != y?=w3090:bool)
              n1532 = Select(t=myRIO_BRig_RT__Case_Exp_stateList."SelectTimeout_post" ("Enum"), s=w3090, f=w3087) -> (s? t:f=w3088:T2)
            }
            frame "SelectTimeout_post" {
            }
            frame "endTrial1" {
              # "Update dataBlock"
              n1533 = call "myRIO_BRig_RT__Case_Exp_State_endTrial1.vi"("input_spout"=w3125, "input_dataBlock"=w3124, "input_dataCurrent"=w3122) -> ("output_dataBlock"=w3123:u16[][], "output_dataCurrent"=w3121:u16[])  [unwired: 7 in]
            }
            frame "endTrial2" {
              # "update dataTrial"
              n1534 = call "myRIO_BRig_RT__Case_Exp_State_endTrial2.vi"("input_dataExp"=w3132, "input_spout"=w3141, "input_dataTrial"=w3145, "input_dataCurrent"=w3143) -> ("output_dataTrial"=w3144:u16[][], "output_dataCurrent"=w3142:u16[])  [unwired: 6 in]
            }
            frame "endTrial3" {
              # "nRewTrials"
              # "iTrial"
              # "I_blockUntilReward"
              # "TPB"
              # "end block?"
              n1535 = local read "STOP_endTrial"() -> (w3166:bool)
              n1536 = local read "STOP_abort"() -> (w3165:bool)
              n1537 = xnode "Read/Write Control"("FPGA VI Reference In"=w3156, "error in"=w3155, "SelectionState"=FALSE) -> ("error out"=w3149:errorcluster)  [unwired: 1 out]
              n1538 = local read "START"() -> (w3163:bool)
              n1539 = call "myRIO_BRig_RT_dataExp_IblockUntilReward.vi"() -> ("output_I_blockUntilReward"=w3173:i32)  [unwired: 11 in]
              n1540 = Index Array(array=w3159, index=w3173) -> (element=w3157:u16)
              n1541 = Not(x=w3163) -> (.not. x?=w3164:bool)
              n1542 = local write "error out"(w3149) -> ()
              n1543 = Not Equal To 0?(x=w3157) -> (x != 0?=w3171:bool)
              n1544 = Compound Arithmetic op=OR(w3166, w3164, w3165) -> (w3152:bool)
              n1545 = call "myRIO_BRig_RT_dataCurrent_nRewTrials.vi"() -> ("output_nRewTrials"=w3169:i32)  [unwired: 11 in]
              n1546 = call "myRIO_BRig_RT_dataCurrent_iTrial.vi"() -> ("output_iTrial"=w3170:i32)  [unwired: 11 in]
              n1547 = Select(t=w3169, s=w3171, f=w3170) -> (s? t:f=w3168:i32)
              n1548 = call "myRIO_BRig_RT_dataCurrent_TpB.vi"() -> ("output_TpB"=w3172:i32)  [unwired: 11 in]
              n1549 = Index Array(array=w3160, index #1=w3172, index #2=w3168) -> (element #1=w3161:u16, element #2=w3162:u16)
              n1550 = Less Or Equal?(x=w3161, y=w3162) -> (x <= y?=w3153:bool)
              n1551 = Or(x=w3152, y=w3153) -> (x .or. y?=w3150:bool)
              n1552 = Select(t=myRIO_BRig_RT__Case_Exp_stateList."saveData_dataBlock" ("Enum"), s=w3150, f=myRIO_BRig_RT__Case_Exp_stateList."dummyState" ("Enum")) -> (s? t:f=w3158:T2)
            }
            frame "endBlock" {
              # "R"
              # "L"
              # "idxDataBlock"
              n1553 = Equal?(x=w3193, y=enum16{"Left", "Right"}."Left") -> (x = y?=w3192:bool)
              n1554 = call "myRIO_BRig_RT_dataCurrent_idxDataBlockL.vi"() -> ("output_idxDataBlock__L"=w3196:i32)  [unwired: 11 in]
              n1555 = call "myRIO_BRig_RT_dataCurrent_idxDataBlockR.vi"() -> ("output_idxDataBlock__R"=w3195:i32)  [unwired: 11 in]
              n1556 = Increment(x=w3187) -> (x+1=w3186:i32)
              n1557 = local read "START"() -> (w3212:bool)
              n1558 = local read "STOP_endBlock"() -> (w3207:bool)
              n1559 = local read "STOP_endTrial"() -> (w3210:bool)
              n1560 = local read "STOP_abort"() -> (w3209:bool)
              n1561 = Select(t=w3196, s=w3192, f=w3195) -> (s? t:f=w3190:i32)
              n1562 = To Unsigned Word Integer(number=w3186) -> (unsigned 16bit integer=w3188:u16)
              n1563 = Not(x=w3212) -> (.not. x?=w3211:bool)
              n1564 = Replace Array Subset(array=w3191, new element=w3188, index=w3190) -> (w3189:u16[])
              n1565 = Compound Arithmetic op=OR(w3211, w3207, w3210, w3209) -> (w3208:bool)
              n1566 = Select(t=myRIO_BRig_RT__Case_Exp_stateList."endExp" ("Enum"), s=w3208, f=myRIO_BRig_RT__Case_Exp_stateList."dummyState_endBlock" ("Enum")) -> (s? t:f=w3216:T2)
            }
            frame "endExp" {
              n1567 = xnode "Read/Write Control"("FPGA VI Reference In"=w3219, "error in"=w3218, "A6_Act"=FALSE) -> ("error out"=w3220:errorcluster)  [unwired: 1 out]
              n1568 = local write "error out"(w3220) -> ()
            }
            frame "commConnect" {
              n1569 = call "myRIO_BRig_RT_comm_webdav_connect.vi"("input_password"="Host Password", "input_username"="Host UserName") -> ("output_Iconnected"=w3237:bool, "output_hSession"=w3251:T6)  [unwired: 7 in, 1 out]
              "Connected To Host?" <- w3237
              n1570 = case shown="False" w3237 {
                frame False {
                  n1571 = One Button Dialog(message="Connection Failed!\nData not being saved!") -> ()  [unwired: 1 in, 1 out]
                }
                frame True {
                }
              }
            }
            frame "commUpload_pre" {
              n1572 = Select(t=myRIO_BRig_RT__Case_Exp_stateList."commUpload_dataBlock" ("Enum"), s=w3258, f=myRIO_BRig_RT__Case_Exp_stateList."endBlock") -> (s? t:f=w3256:T2)
            }
            frame "commUpload_dataBlock" {
              n1573 = call "myRIO_BRig_RT_comm_webdav_uploadFile__data.vi"("input_fileName_prefix"=w3275, "input_fileName"="dataBlock" ("input_filename"), "input_hSession"=w3277) -> ()  [unwired: 8 in, 1 out]
            }
            frame "commUpload_dataCurrent" {
              n1574 = call "myRIO_BRig_RT_comm_webdav_uploadFile__data.vi"("input_fileName_prefix"=w3292, "input_fileName"="dataCurrent" ("input_filename"), "input_hSession"=w3294) -> ()  [unwired: 8 in, 1 out]
            }
            frame "commUpload_dataExp" {
              n1575 = call "myRIO_BRig_RT_comm_webdav_uploadFile__data.vi"("input_fileName_prefix"=w3309, "input_fileName"="dataExp" ("input_filename"), "input_hSession"=w3311) -> ()  [unwired: 8 in, 1 out]
            }
            frame "commUpload_dataLC" {
              n1576 = call "myRIO_BRig_RT_comm_webdav_uploadFile__data.vi"("input_fileName_prefix"=w3326, "input_fileName"="dataLC" ("input_filename"), "input_hSession"=w3328) -> ()  [unwired: 8 in, 1 out]
            }
            frame "commUpload_dataTrial" {
              n1577 = call "myRIO_BRig_RT_comm_webdav_uploadFile__data.vi"("input_fileName_prefix"=w3346, "input_fileName"="dataTrial" ("input_filename"), "input_hSession"=w3348) -> ()  [unwired: 8 in, 1 out]
            }
            frame "saveData_dataBlock" {
              # "idxDataBlockR"
              # "idxDataBlockL"
              n1578 = call "myRIO_BRig_RT_dataCurrent_idxDataBlockL.vi"() -> ("output_idxDataBlock__L"=w3368:i32)  [unwired: 11 in]
              n1579 = call "myRIO_BRig_RT_dataCurrent_idxDataBlockR.vi"() -> ("output_idxDataBlock__R"=w3369:i32)  [unwired: 11 in]
              n1580 = Index Array(array=w3370, index #1=w3368, index #2=w3369) -> (element #1=w3367:u16, element #2=w3366:u16)
              n1581 = Greater?(x=w3367, y=w3366) -> (0:w3365:bool)
              n1582 = Select(t=w3367, s=w3365, f=w3366) -> (s? t:f=w3363:u16)
              n1583 = Increment(x=w3363) -> (x+1=w3362:u16)
              n1584 = To Long Integer(number=w3362) -> (32bit integer=w3361:i32)
              n1585 = Array Subset(array=w3364, length (row)=w3361) -> (w3360:u16[][])  [unwired: 3 in]
              n1586 = call "myRIO_BRig_RT_comm_webdav_saveArrayToFile__2D_u16.vi"("Array"=w3360, "input_filename"="dataBlock") -> ()  [unwired: 10 in]
            }
            frame "saveData_dataCurrent" {
              n1587 = call "myRIO_BRig_RT_comm_webdav_saveArrayToFile__1D_u16.vi"("Array"=w3385, "input_filename"="dataCurrent") -> ()  [unwired: 10 in]
            }
            frame "saveData_dataExp" {
              # "runTime"
              n1588 = Get Date/Time In Seconds() -> (seconds since 1Jan1904=w3409:timestamp)
              n1589 = To Double Precision Float(number=w3409) -> (double precision float=w3408:dbl)
              n1590 = call "myRIO_BRig_RT_dataExp_runTime_seconds.vi"() -> ("output_RunTime_minutes"=w3407:i32)  [unwired: 11 in]
              n1591 = Subtract(x=w3408, y=w3406) -> (x-y=w3403:dbl)
              n1592 = To Unsigned Word Integer(number=w3403) -> (unsigned 16bit integer=w3402:u16)
              n1593 = Replace Array Subset(array=w3401, new element=w3402, index=w3407) -> (w3404:u16[])
              n1594 = call "myRIO_BRig_RT_comm_webdav_saveArrayToFile__1D_u16.vi"("Array"=w3404, "input_filename"="dataExp") -> ()  [unwired: 10 in]
            }
            frame "saveData_dataLC" {
              n1595 = call "myRIO_BRig_RT_comm_webdav_saveArrayToFile__1D_u16.vi"("Array"=w3424, "input_filename"="dataLC") -> ()  [unwired: 10 in]
            }
            frame "saveData_dataTrial" {
              # "idxTrial"
              n1596 = call "myRIO_BRig_RT_dataCurrent_idxDataTrial.vi"() -> ("output_idxDataTrial"=w3444:i32)  [unwired: 11 in]
              n1597 = Index Array(array=w3445, index=w3444) -> (element=w3437:u16)
              n1598 = Increment(x=w3437) -> ()  [unwired: 1 out]
              n1599 = To Long Integer(number=w3437) -> (32bit integer=w3441:i32)
              n1600 = Array Subset(array=w3442, length (row)=w3441) -> (w3443:u16[][])  [unwired: 3 in]
              n1601 = call "myRIO_BRig_RT_comm_webdav_saveArrayToFile__2D_u16.vi"("Array"=w3443, "input_filename"="dataTrial") -> ()  [unwired: 10 in]
            }
            frame "dummyState" {
              n1602 = call "myRIO_BRig_RT_dataCurrent_iTrial.vi"() -> ("output_iTrial"=w3463:i32)  [unwired: 11 in]
              n1603 = Index Array(array=w3464, index=w3463) -> (element=w3462:u16)
              n1604 = Equal?(x=w3462, y=u16 1) -> (x = y?=w3460:bool)
              n1605 = Equal To 0?(x=w3471) -> (x = 0?=w3472:bool)
              n1606 = Select(t=u16 13, s=w3460, f=u16 15) -> (s? t:f=w3457:u16)
              n1607 = Select(t=w3457, s=w3472, f=w3471) -> (s? t:f=w3470:u16)
              n1608 = Decrement(x=w3470) -> (x-1=w3469:u16)
              n1609 = Equal To 0?(x=w3469) -> (x = 0?=w3468:bool)
              n1610 = Select(t=myRIO_BRig_RT__Case_Exp_stateList."initTrial" ("Enum"), s=w3468, f=w3466) -> (s? t:f=w3465:T2)
            }
            frame "dummyState_endBlock" {
              n1611 = call "myRIO_BRig_RT_dataCurrent_iTrial.vi"() -> ("output_iTrial"=w3492:i32)  [unwired: 11 in]
              n1612 = Index Array(array=w3493, index=w3492) -> (element=w3491:u16)
              n1613 = Equal?(x=w3491, y=u16 1) -> (x = y?=w3489:bool)
              n1614 = Equal To 0?(x=w3500) -> (x = 0?=w3501:bool)
              n1615 = Select(t=u16 1, s=w3489, f=u16 3) -> (s? t:f=w3486:u16)
              n1616 = Select(t=w3486, s=w3501, f=w3500) -> (s? t:f=w3499:u16)
              n1617 = Decrement(x=w3499) -> (x-1=w3498:u16)
              n1618 = Equal To 0?(x=w3498) -> (x = 0?=w3497:bool)
              n1619 = Select(t=myRIO_BRig_RT__Case_Exp_stateList."initBlock" ("Enum"), s=w3497, f=w3495) -> (s? t:f=w3494:T2)
            }
          }
          n1620 = call "myRIO_BRig_RT_dataMTrig_main.vi"("input_dataMTrig"=w1584, "input_Solenoid_trig_L"=w1581, "input_Solenoid_trig_R"=w1580, "input_Audio_trig_L"=w1579, "input_Audio_trig_R"=w1578, "input_Laser_trig"=w1577) -> ("output_Laser"=w1518:bool, "output_dataMTrig"=w1583:u16[], "output_Solenoid_L"=w1521:bool, "output_Solenoid_R"=w1573:bool, "output_Audio_L"=w1575:bool, "output_Audio_R"=w1576:bool)  [unwired: 8 in]
          n1621 = Compound Arithmetic op=OR(w1581, w1580, w1579, w1578, w1577) -> (w1582:bool)
          n1622 = case shown="True" w1582 {
            frame False {
            }
            frame True {
              w1614 = FALSE
              n1623 = local write "MTrig_Solenoid_trig__L"(w1614) -> ()
              n1624 = local write "MTrig_Solenoid_trig__R"(w1614) -> ()
              n1625 = local write "MTrig_Audio_trig__L"(w1614) -> ()
              n1626 = local write "MTrig_Audio_trig__R"(w1614) -> ()
              n1627 = local write "MTrig_Laser_trig"(w1614) -> ()
            }
          }
          n1628 = local read "MTrig_Laser_Switch"() -> (w1516:bool)
          n1629 = Not(x=w1516) -> (.not. x?=w1517:bool)
          n1630 = And(x=w1518, y=w1517) -> (x .and. y?=w1512:bool)
          n1631 = And(x=w1518, y=w1516) -> (x .and. y?=w1514:bool)
          n1632 = Or(x=w1515, y=w1514) -> (x .or. y?=w1505:bool)
          n1633 = Or(x=w1514, y=w1513) -> (x .or. y?=w1504:bool)
          n1634 = Or(x=w1511, y=w1512) -> (x .or. y?=w1507:bool)
          n1635 = Or(x=w1512, y=w1510) -> (x .or. y?=w1506:bool)
          n1636 = Or(x=w1520, y=w1521) -> (x .or. y?=w1509:bool)
          n1637 = Or(x=w1574, y=w1573) -> (x .or. y?=w1508:bool)
          n1638 = case shown="False" w1594 {
            tunnel: w1591 -> [w1616 w1624]
            tunnel: w1593 -> [_ w1621]
            tunnel: w1592 -> [_ w1620]
            tunnel: w1495 -> [_ w1619]
            tunnel: w1571 -> [_ w1618]
            tunnel: [w1616 w1623] -> w1590
            tunnel: [w1615 w1622] -> w1589
            tunnel: w1503 -> [w1615 w1617]
            frame False {
            }
            frame True {
              n1639 = call "myRIO_BRig_RT__Case_Exp__recordLick.vi"("intput_state__trialEnd"=w1618, "intput_state__trialStart"=w1619, "input_lick__R"=w1620, "input_lick__L"=w1621, "input_dataCurrent"=w1617, "input_dataLick"=w1624) -> ("output_dataCurrent"=w1622:u16[], "output_dataLick"=w1623:u16[][])  [unwired: 4 in]
            }
          }
          n1640 = Or(x=w1575, y=w1561) -> (x .or. y?=w1551:bool)
          n1641 = Or(x=w1560, y=w1576) -> (x .or. y?=w1572:bool)
          n1642 = Or(x=w1595, y="STOP_abort") -> (x .or. y?=w1597:bool)
          n1643 = Select(t=w1541, s=w1542, f=w1540) -> (s? t:f=w1531:u16)
          n1644 = Select(t=w1502, s=w1544, f=w1543) -> (s? t:f=w1530:u16)
          n1645 = Select(t=u16 0, s=w1547, f=w1546) -> (s? t:f=w1533:u16)
          n1646 = xnode "Read/Write Control"("FPGA VI Reference In"=w1553, "error in"=w1552, "audioTrigger_L"=w1551, "audioTrigger_R"=w1572, "CueLed_Event"=w1519, "A3_SL"=w1509, "A1_SR"=w1508, "LC_Event_l1"=w1507, "LC_Laser_l1"=w1506, "LC_Event_l2"=w1505, "LC_Laser_l2"=w1504) -> ("FPGA VI Reference Out"=w1588:refnum<k20>, "error out"=w1587:errorcluster, "AnaIn_0"=w1524:i16, "AnaIn_1"=w1532:i16)
          n1647 = call "myRIO_BRig_RT_dataAnalog_enterData__PortC.vi"("input_iState"=w1495, "input_AI0"=w1524, "input_iEvent"=w1533, "input_AI1"=w1532, "input_iTrial"=w1531, "input_iBlock"=w1530, "input_index"=w1534, "input_dataAnalog"=w1550) -> ("output_dataAnalog"=w1549:u16[][])  [unwired: 3 in]
          n1648 = call "myRIO_BRig_RT_TCP__v3__PortC.vi"("input_hTCP"=w1538, "input_AI1"=w1532, "input_AI0"=w1524, "input_I_connected_TCP"=w1535, "input_iBlock"=w1530, "input_spout"=w1529, "input_iTrial"=w1531, "input_error"=w1536, "input_countTrial"=w1526, "input_iState"=w1495) -> ("output_hTCP"=w1537:refnum<k5>, "output_countTrial"=w1525:u16, "output_error"=w1499:errorcluster)  [unwired: 3 in]
          n1649 = call "test_myRIO_Exp_tLoop.vi"("input_error"=w1499, "input_Threshold"=w1496, "input_timestamp"=w1497, "input_state"=w1495) -> ("output_Threshold"=w1493:bool, "output_duration"=→"tLoop":dbl, "error out"=w1498:errorcluster)  [unwired: 5 in]
          "Threshold" <- w1493
          n1650 = node-c288() -> ()  [unwired: 1 in, 1 out]
          n1651 = Increment(x=w1533) -> (x+1=w1539:u16)
          n1652 = Increment(x=w1534) -> (x+1=w1548:i32)
          "cState" <- w1495
        }
        n1653 = node-c288(w1436) -> ()  [unwired: 1 out]
        n1654 = flat-sequence {
          tunnel: w1432 -> [w1481]
          tunnel: w1431 -> [w1480]
          tunnel: [w1479] -> w1424
          tunnel: [w1478] -> w1423
          tunnel: [w1484] -> w1425
          tunnel: [w1485] -> w1430
          tunnel: w1424 -> [w1485]
          tunnel: w1423 -> [w1484]
          frame #0 {
            w1475 = u8 0
            w1476 = u16 0 ("AudioLeft_phase_inc")
            w1477 = FALSE
            n1655 = xnode "Read/Write Control"("FPGA VI Reference In"=w1481, "error in"=w1480, "Counts_Reset"=TRUE, "audioTrigger_L"=w1477, "audioFreq_L_kHz"=w1475, "audioAmp_L"=w1476, "audioTrigger_R"=w1477, "audioFreq_R_kHz"=w1475, "audioAmp_R"=w1476, "A3_SL"=w1477, "A1_SR"=w1477, "A6_Act"=w1477) -> ("FPGA VI Reference Out"=w1479:refnum<k20>, "error out"=w1478:errorcluster)
          }
          frame #1 {
            w1483 = FALSE ("START")
            n1656 = local write "START"(w1483) -> ()
            n1657 = local write "STOP_endTrial"(w1483) -> ()
            n1658 = local write "STOP_endBlock"(w1483) -> ()
          }
        }
        n1659 = stacked-sequence {
          tunnel: w1409 -> [w1455 _]
          tunnel: w1407 -> [w1456 _]
          tunnel: w1406 -> [_ w1461]
          tunnel: w1405 -> [_ w1460]
          tunnel: w1404 -> [_ w1459]
          tunnel: w1403 -> [w1449 _]
          tunnel: w1385 -> [w1446 _]
          tunnel: w1384 -> [w1445 _]
          frame #0 {
            n1660 = call "myRIO_BRig_RT_dataCurrent_idxDataLick.vi"() -> ("output_idxDataLick"=w1450:i32)  [unwired: 11 in]
            n1661 = Index Array(array=w1449, index=w1450) -> (element=w1452:u16)
            n1662 = Array Subset(array=w1446, length (row)=w1445) -> (w1447:u16[][])  [unwired: 3 in]
            n1663 = Increment(x=w1452) -> (x+1=w1453:u16)
            n1664 = call "myRIO_BRig_RT_comm_webdav_saveArrayToFile__1D_u16.vi"("Array"=w1456, "input_filename"="dataMTrig") -> ()  [unwired: 10 in]
            n1665 = To Long Integer(number=w1453) -> (32bit integer=w1451:i32)
            n1666 = Array Subset(array=w1455, length (row)=w1451) -> (w1454:u16[][])  [unwired: 3 in]
            n1667 = call "myRIO_BRig_RT_comm_webdav_saveArrayToFile__2D_u16.vi"("Array"=w1454, "input_filename"="dataLick") -> ()  [unwired: 10 in]
            n1668 = call "myRIO_BRig_RT_comm_webdav_saveArrayToFile__2D_u16.vi"("Array"=w1447, "input_filename"="dataAnalog") -> ()  [unwired: 10 in]
          }
          frame #1 {
            n1669 = case shown="True" w1461 {
              tunnel: w1460 -> [_ w1463]
              tunnel: w1459 -> [_ w1462]
              frame False {
              }
              frame True {
                n1670 = stacked-sequence {
                  tunnel: w1463 -> [w1465 w1472 w1474]
                  tunnel: w1462 -> [w1466 w1471 _]
                  frame #0 {
                    n1671 = call "myRIO_BRig_RT_comm_webdav_uploadFile__announce.vi"("input_addText"=TRUE, "input_fileName_prefix"=w1466, "intput_fileName"="curExp_end", "intput_hSession"=w1465) -> ("output_Isuccess"=w1464:bool)  [unwired: 6 in, 1 out]
                    n1672 = case shown="True" w1464 {
                      frame False {
                        n1673 = One Button Dialog(message="!!! Warning !!! Your data is located at C:\\BehaviorRig\\commTransfer") -> ()  [unwired: 1 in, 1 out]
                      }
                      frame True {
                        n1674 = Wait (ms)(milliseconds to wait=u32 20) -> ()  [unwired: 1 out]
                      }
                    }
                  }
                  frame #1 {
                    n1675 = call "myRIO_BRig_RT__endExp_sendData.vi"("input_fileName_prefix"=w1471, "input_hSession"=w1472) -> ()  [unwired: 8 in, 2 out]
                  }
                  frame #2 {
                    n1676 = local write "Connected To Host?"(FALSE ("Connected To Host?")) -> ()
                    n1677 = call <vilib>:"Close Session.vi"("session handle"=w1474) -> ()  [unwired: 14 in, 1 out]
                  }
                }
              }
            }
          }
        }
      }
    }
    n1678 = local read "STOP_abort"() -> (w44:bool)
  }
  n1679 = case shown="True" w5 {
    tunnel: w4 -> [_ w3520]
    tunnel: w3 -> [_ w3519]
    frame False {
    }
    frame True {
      n1680 = call "myRIO__TCP_disconnect_forWrite.vi"("input_error"=w3519, "input_hTCP"=w3520) -> ()  [unwired: 9 in, 1 out]
    }
  }
  n1681 = xnode "Read/Write Control"("FPGA VI Reference In"=w16, "error in"=w15, "FPGA_Stop"=TRUE) -> ("FPGA VI Reference Out"=w21:refnum<k20>, "error out"=w22:errorcluster)
  n1682 = xnode "Close FPGA VI Reference"("FPGA VI Reference In"=w21, "error in"=w22) -> ("error out"=w20:errorcluster)
  n1683 = call <vilib>:"Reset myRIO.vi"("error in (no error)"=w20) -> ()  [unwired: 10 in, 1 out]
